vi "COD主界面（列队使用）.vi"() -> (8 "多列列表框":i32(listbox))   [LabVIEW 2016, in "斯坦道CODMn.lvlib"]
uses:
  <vilib>/Analysis/6fits.llb/Curve Fitting Criteria.ctl
  <vilib>/Utility/miscctls.llb/LVPointTypeDef.ctl
  <vilib>/Utility/config.llb/Read Key (I32).vi
  <vilib>/Utility/config.llb/Read Key (Double).vi
  <vilib>/Utility/config.llb/Read Key (Boolean).vi
  <vilib>/Utility/config.llb/Write Key (I32).vi
  <vilib>/Utility/config.llb/Write Key (Double).vi
  <vilib>/Utility/config.llb/Write Key (Boolean).vi
  <vilib>/Waveform/WDTFileIO.llb/Read Waveform from File.vi
  <vilib>/ptbypt/NI_PtbyPt.lvlib
  <vilib>/Utility/config.llb/NI_LVConfig.lvlib
  <vilib>/Analysis/NI_AALPro.lvlib
panel:
  out "氢氧化钠":dbl
  in  "序列号变更":bool
  out "模块版本号":string
  in  "更新程序":bool
  out "进样无液体告警":bool
  out "校准内容显示":string
  out "60分钟超时报警":bool
  in  "远程校准量程":enum16{"L", "H"}(ring)
  in  "远程自动校准浓度":dbl
  in  "仪器参数":bool
  out "CODMn序列号":string
  out "CODMn软件版本：":string
  in  "标样核查量程选择":enum32{"H", "L", "AUTO"}(ring)=enum."AUTO"
  in  "标样浓度":dbl
  in  "零点核查量程选择":enum32{"H", "L", "AUTO"}(ring)=enum."AUTO"
  in  "零点核查浓度":dbl
  out "序列号":string
  in  "采水泵排液时间/s:":i32
  in  "采水泵润洗时间/s:":i32
  in  "采水泵沉淀时间/s:":i32
  in  "采水泵进样时间/s:":i32
  in  "常规版/认证版":enum16{"常规版-酸性", "常规版-碱性", "认证版", "浮台版"}(ring)
  in  "释放串口":bool
  in  "打开串口":bool
  in  "保存参数":dbl[](array[numeric])
  out "报警数字":i16
  out "CODMn工作状态":T1(ring)
  out "ORP-K":string
  out "ORP-B":string
  out "ORP-A":string
  out "x = y?":bool
  out "稀释倍数解释":string
  in  "跨度量程选择":enum32{"H", "L", "AUTO"}(ring)=enum."AUTO"
  in  "跨度液浓度":dbl
  in  "水样：":dbl
  in  "蒸馏水：":dbl
  in  "标液：":dbl
  in  "零点核查样：":dbl
  in  "加标回收样：":dbl
  in  "草酸钠":dbl
  in  "高锰酸钾":dbl
  in  "硫酸":dbl
  out "量程解释说明":string
  in  "高切低阈值:":dbl
  in  "低切高阈值:":dbl
  in  "水样量程选择:":enum16{"L", "H", "自动切换测一次", "自动切换测两次"}(ring)
  in  "氢氧化钠：":dbl
  in  "标准液浓度":dbl
  in  "温度":dbl
  in  "恒温时间":dbl
  in  "当前量程：":enum16{"L", "H"}(ring)
  in  "CODMn零点核查选择":enum16{"零点核查走纯水管", "零点核查走零漂管"}(ring)
  in  "锁定按钮":bool
  in  "低量程稀释倍数:":i8=1
  in  "高量程稀释倍数:":i8=2
  in  "一键写入":bool
  in  "测量模式(公式)":u16(ring)=1 items=["水样测试"=1, "标样核查"=2, "零点核查"=3, "跨度核查"=4, "空白测试"=5, "平行样"=6, "加标回收"=7]
  out "基本量程(显示)":string
  out "测量模式(显示)":string
  out "数据时间":string
  out "断电排液标记":bool
  out "COM":string
  in  "启用5":bool
  in  "校准5":bool
  in  "泵滴定数5":dbl
  in  "浓度5":dbl
  in  "启用4":bool
  in  "校准4":bool
  in  "泵滴定数4":dbl
  in  "浓度4":dbl
  out "波形时间":timestamp
  in  "历史波形":bool
  out "滴定数-ORP值":u16[](array[numeric]) caption="数组"
  in  "关闭 3":bool
  in  "滴定曲线":bool
  out "ORP滴定曲线":u16[](graph)
  out "空白测试标记":bool
  out "跨度核查标记":bool
  in  "量程选择":enum16{"低量程", "高量程", "0-2量程"}(ring)
  in  "手动控制":bool
  in  "选用水样":enum16{"葡萄糖", "草酸钠"}(ring)
  in  "方程系数":cluster{"K":dbl, "b":dbl, "X^2":dbl} {"X^2" format="%#.6g"; "b" format="%#.6g"; "K" format="%#.6g"}
  out "多项式系数":dbl[](array[numeric])
  out "XY图":cluster{"X Values":dbl[], "Y Values":dbl[]}[](graph)
  in  "模型":enum32{"线性", "多项式"}(ring)
  out "启动时间":timestamp format="%<%Y/%m/%d %H:%M:%S>T"
  in  "关闭 2":bool
  out "r^2":dbl format="%.8g"
  out "拟合公式":string
  out "b":dbl format="%#.4g"
  out "K":dbl format="%#.4f"
  in  "启用3":bool
  in  "启用2":bool
  in  "启用1":bool
  in  "校准3":bool
  in  "校准2":bool
  in  "校准1":bool
  in  "泵滴定数3":dbl
  in  "泵滴定数2":dbl
  in  "泵滴定数1":dbl
  in  "浓度3":dbl
  in  "浓度2":dbl
  in  "浓度1":dbl
  in  "写入":bool
  out "零点核查标记":bool
  out "排液故障":bool
  out "进水样超量程":bool
  out "标样核查标记":bool
  out "平行样测量":bool
  out "加标回收测量":bool
  out "质控样测量":bool
  out "待机":bool
  out "校标错误":bool
  out "校零错误":bool
  out "测量错误":bool
  out "草酸钠报警":bool
  out "高锰酸钾报警":bool
  out "加热故障":bool
  out "温控器故障":bool
  out "ORP故障":bool
  out "排液标记":bool
  out "故障标记":bool
  out "校标标记":bool
  out "校零标记":bool
  out "通讯状态":bool
  out "水样测量":bool
  in  "读取":bool
  in  "返回":bool
  in  "校准配置":bool
  in  "零点泵计量数 2":dbl
  in  "标度泵计量数 2":dbl
  out "标度滴定值":dbl
  out "零点滴定值":dbl
  in  "保存":bool
  in  "关闭":bool
  out "仪器时间":timestamp format="%<%Y/%m/%d %H:%M:%S>T"
  out "秒":u16
  out "分":u16
  out "COD浓度（mg/L)":dbl format="%.2g"
  out "进样管":dbl
  out "高锰酸钾":dbl
  out "草酸钠":dbl
  out "硫酸":dbl
  out "实时ORP":dbl
  out "温度℃":dbl
  out "加热":bool
  out "搅拌":bool
  out "进硫酸":bool
  out "进加标回收样":bool
  out "进零点核查样":bool
  out "进标液":bool
  out "进蒸馏水":bool
  out "进水样":bool
  out "进草酸钠":bool
  out "进高锰酸钾":bool
  out "定时启动":bool
  in  "启动":bool
  in  "故障清除":bool
  in  "参数配置":bool
  in  "停止":bool
  in  "单步启动":bool
  out "系统时间":timestamp
  in  "时间校准":bool
  out "模式（受控）":u16
  # "测试时长："
  # "注：遇到加热故障和排液故障时仪器不能正常启动，\n必须排查故障并点击报警清除按钮方可运行。"
  # "mg/L"
  # "基本参数设置"
  # "校零校标结果"
  # "泵计量参数设置"
  # "校零结果："
  # "校零滴定值："
  # "加热恒温温度(℃):"
  # "高锰酸钾："
  # "校标结果："
  # "标度滴定值："
  # "恒温时间(分钟):"
  # "草酸钠："
  # "零点泵计量值："
  # "标准液浓度(mg/L):"
  # "硫酸："
  # "标度泵计量值："
  # "跨度核查浓度："
  # "跨度量程选择："
  # "零点核查浓度："
  # "标样浓度："
  # "零点量程选择："
  # "标样量程选择："
  # "远程校准配置区"
  # "公式读取写入区"
  # "mg/L"
  # "是否启用"
  # "泵滴定数"
  # "浓度"
  # "辅\n助\n计\n算\n区"
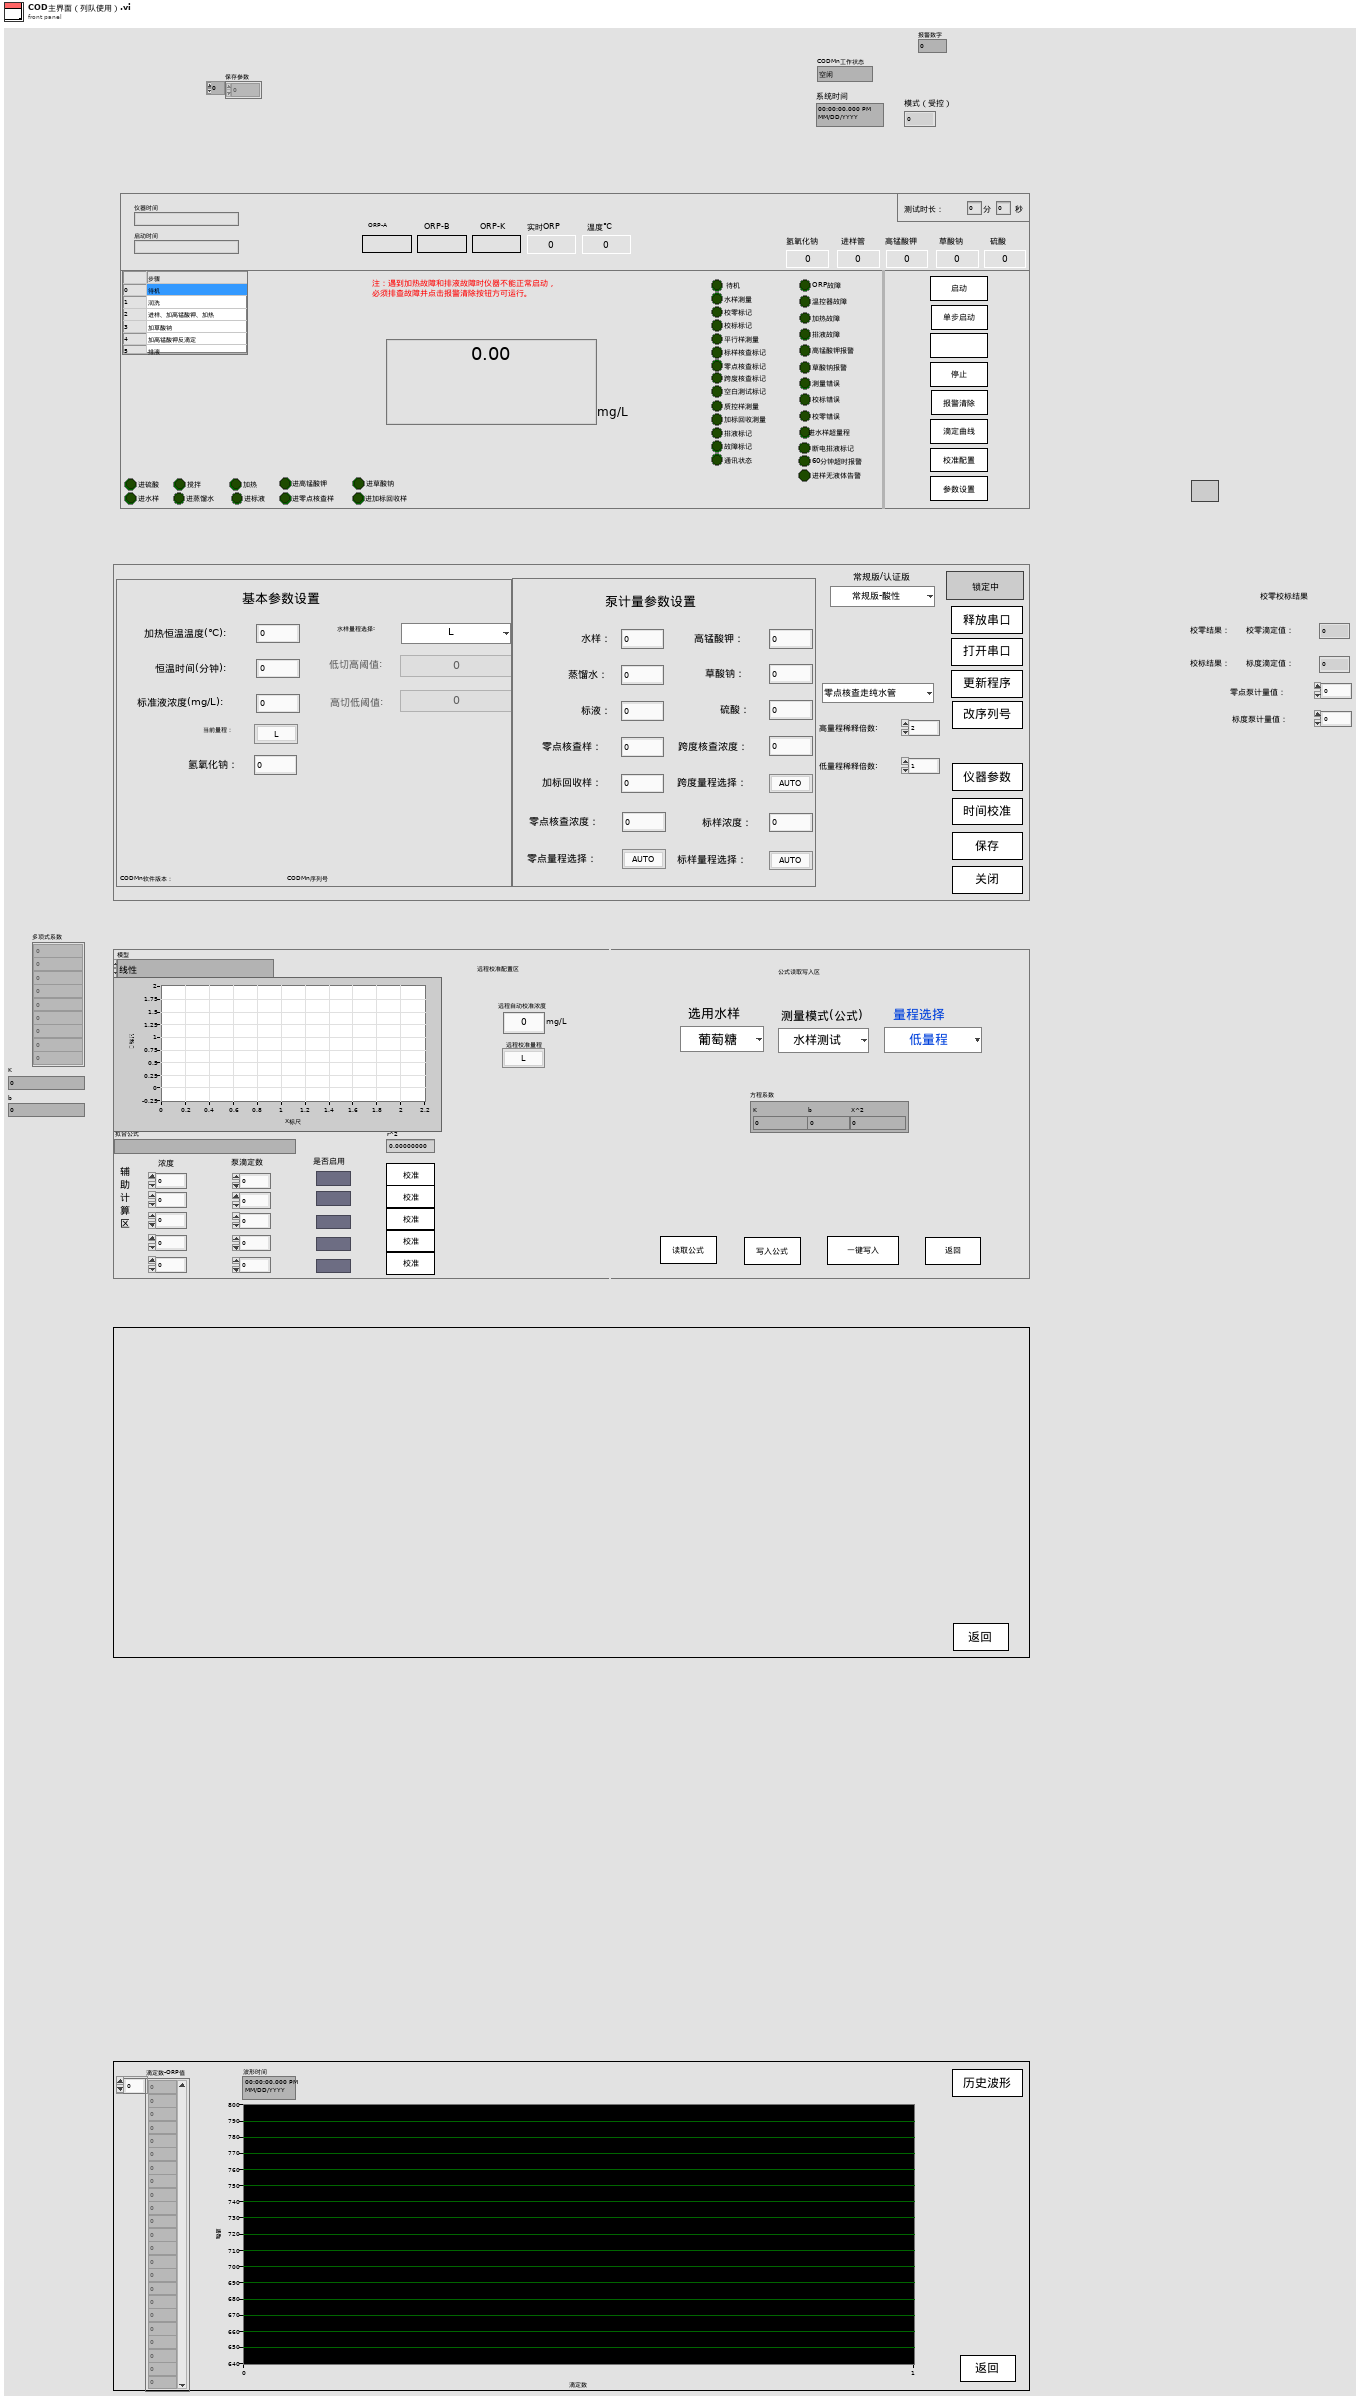
[diagram p1: front panel]
types:
  T1 = enum16{"空闲", "水样测试", "标样核查", "零点核查", "跨度核查", "空白测试", "平行样测试", "质控样", "空白校准", "标样校准", "加标回收"}
  T2 = typedef "LVPointTypeDef.ctl" = cluster{"Horizontal":i16, "Vertical":i16}
  T3 = cluster{"Major":u16, "Minor":u16, "Fix":u16, "Build":u16}
  T4 = typedef "NI_LVConfig.lvlib/Config Data RefNum.ctl" = refnum<k1>
  T5 = cluster{"时间标识":timestamp, "参数":string, "日志信息":string, "流程参数":string}
  T6 = cluster{"时间标识":timestamp, "设备":string, "日志信息":string, "流程参数":string}
  T7 = enum8{"Enabled", "Disabled", "Disabled and Grayed Out"}
  T8 = cluster{"时间":timestamp, "测量模式":string, "数据类型":string, "检测值":sgl, "单位":string, "数据标识":string, "因子编码":string, "标样参考值":sgl, "ORP-A":sgl, "ORP-B":sgl, "ORP-K":sgl, "COD滴定值":sgl, "高锰酸钾滴定数":sgl, "温度":sgl, "量程":sgl, "LastTime":timestamp, "序列号:":string}
  T9 = cluster{"因子编码":u32, "单位":u16, "标样参考值":sgl, "水样数据时间":timestamp, "水样实测值":sgl, "水样数据标识":string, "标样数据时间":timestamp, "标样实测值":sgl, "标样数据标识":string, "空白数据时间":timestamp, "空白实测值":sgl, "空白数据标识":string, "零点核查数据时间":timestamp, "零点核查实测值":sgl, "零点核查数据标识":string, "跨度核查数据时间":timestamp, "跨度核查实测值":sgl, "跨度核查数据标识":string, "加标回收数据时间":timestamp, "加标回收实测值":sgl, "加标回收数据标识":string, "平行样数据时间":timestamp, "平行样实测值":sgl, "平行样数据标识":string}
  T10 = cluster{"控制命令":enum16{"启动测量", "标样核查", "零点核查", "跨度核查", "空白测试", "平行样测试", "加标回收", "空白校准", "标样校准", "初始化（清洗）", "停止测试", "仪器重启", "校时", "模式设置", "测量间隔设置"}, "周期设置类型":enum16{"定点启动", "间隔启动"}, "定时功能启用":bool, "定时间隔":dbl, "24H周期设置":bool[], "零点核查时间":u16, "跨度核查时间":u16, "质控频次":enum16{"关闭", "每天", "星期一", "星期二", "星期三", "星期四", "星期五", "星期六", "星期日"}}
  T11 = cluster{"数组 2[0]":sgl, "数组 2[1]":sgl, "数组 2[2]":sgl, "数组 2[3]":sgl, "数组 2[4]":sgl, "数组 2[5]":sgl, "数组 2[6]":sgl, "数组 2[7]":sgl, "数组 2[8]":sgl, "数组 2[9]":sgl, "数组 2[10]":sgl, "数组 2[11]":sgl, "数组 2[12]":sgl, "数组 2[13]":sgl, "数组 2[14]":sgl, "数组 2[15]":sgl, "数组 2[16]":sgl, "数组 2[17]":sgl, "数组 2[18]":sgl, "数组 2[19]":sgl, "数组 2[20]":sgl, "数组 2[21]":sgl, "数组 2[22]":sgl, "数组 2[23]":sgl, "数组 2[24]":sgl, "数组 2[25]":sgl, "数组 2[26]":sgl, "数组 2[27]":sgl, "数组 2[28]":sgl, "数组 2[29]":sgl, "数组 2[30]":sgl, "数组 2[31]":sgl, "数组 2[32]":sgl, "数组 2[33]":sgl, "数组 2[34]":sgl, "数组 2[35]":sgl, "数组 2[36]":sgl, "数组 2[37]":sgl, "数组 2[38]":sgl, "数组 2[39]":sgl, "数组 2[40]":sgl, "数组 2[41]":sgl}
  T12 = cluster{"ORP故障":bool, "温控器故障":bool, "加热故障":bool, "高锰酸钾报警":bool, "草酸钠报警":bool, "测量错误":bool, "校零错误":bool, "校标错误":bool, " 进水样超量程":bool, "排液阀故障":bool, "60分钟超时报警":bool, "进样无液体报警":bool}
  T13 = cluster{"控制命令":enum16{"启动测量", "标样核查", "零点核查", "跨度核查", "空白测试", "平行样测试", "加标回收", "空白校准", "标样校准", "初始化（清洗）", "停止测试", "仪器重启", "校时", "模式设置", "测量间隔设置"}, "周期设置类型":enum16{"定点启动", "间隔启动"}, "定时功能启用":bool, "定时间隔":dbl, "24H周期设置":bool[], "空白核查时间":u16, "跨度核查时间":u16, "质控频次":enum16{"关闭", "每天", "星期一", "星期二", "星期三", "星期四", "星期五", "星期六", "星期日"}}
  T14 = cluster{"测量量程":dbl, "测量精度":dbl, "测量间隔":dbl, "消解温度":dbl, "消解时长":dbl, "空白校准时间":timestamp, "曲线截距":dbl, "曲线斜率":dbl, "测量检出限":dbl, "测量信号值":dbl, "线性相关系数":dbl, "二次多项式系数":dbl, "标样校准时间":timestamp, "稀释倍数":dbl, "三项式系数":dbl, "空白标定系数":dbl, "量程系数":dbl, "F0/ORPA":dbl, "F1/ORPB":dbl, "F2/ORPK":dbl, "F3":dbl, "F4":dbl, "F5":dbl, "F6":dbl, "F7":dbl, "X0/滴定数":dbl, "量程":dbl}
  T15 = cluster{"确定":bool, "测量量程":dbl, "测量精度":dbl, "测量间隔":dbl, "消解温度":dbl, "消解时长":dbl, "空白校准时间":timestamp, "曲线截距":dbl, "曲线斜率":dbl, "测量检出限":dbl, "测量信号值":dbl, "线性相关系数":dbl, "二次多项式系数":dbl, "标样校准时间":timestamp, "稀释倍数":dbl, "三项式系数":dbl, "空白标定系数":dbl, "量程系数":dbl, "F0/ORPA":dbl, "F1/ORPB":dbl, "F2/ORPK":dbl, "F3":dbl, "F4":dbl, "F5":dbl, "F6":dbl, "F7":dbl, "X0/滴定数":dbl, "量程":dbl}
  T16 = typedef "NI_AALPro.lvlib/Curve Fitting Criteria.ctl" = u16
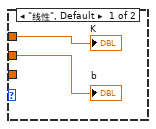
[diagram p5: hidden frame]
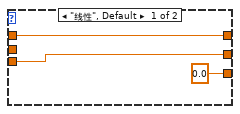
[diagram p7: hidden frame]
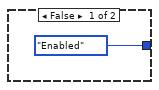
[diagram p8: hidden frame]
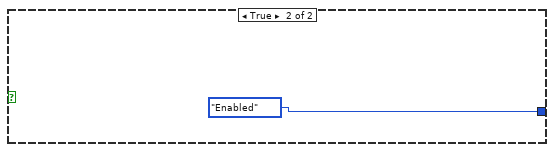
[diagram p9: hidden frame]
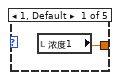
[diagram p14: hidden frame]
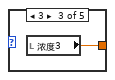
[diagram p15: hidden frame]
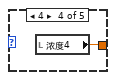
[diagram p16: hidden frame]
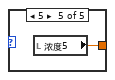
[diagram p17: hidden frame]
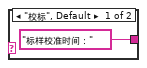
[diagram p18: hidden frame]
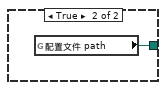
[diagram p19: hidden frame]
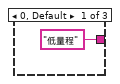
[diagram p20: hidden frame]
diagram:
  n1 = flat-sequence {
    tunnel: [w69] -> w17
    tunnel: [errorcluster {"status"=FALSE, "code"=0, "source"=""} ("错误输出")] -> w54
    tunnel: [w71] -> w16
    frame #0 {
      w93 = "192.168.1.100" ("名称")
      n2 = global write "COD内部交互全局.vi" "量程切换次数"(u8 0 ("量程切换次数")) -> ()
      n3 = global write "COD内部交互全局.vi" "切换量程连续测两次"(FALSE ("切换量程连续测两次")) -> ()
      n4 = global read "COD内部交互全局.vi" "序列号:"() -> (w100:string)
      n5 = property on="窗格" class="Pane"("Origin"=T2 {"Horizontal"=0, "Vertical"=0} ("原点")) -> ()  [unwired: 2 in, 2 out]
      n6 = Empty String/Path?(string/path=w100) -> (empty?=w68:bool)
      n7 = case shown="真" w68 {
        tunnel: w100 -> [w115 _]
        tunnel: [w114 "data\\CODMnSet.ini" ("名称或相对路径")] -> w81
        frame False {
          # "与生产用上位机交互"
          n8 = Concatenate Strings("data\\" ("字符串"), "序列号" ("字符串"), w115, "Set.ini" ("名称或相对路径")) -> (w114:string)
        }
        frame True {
        }
      }
      n9 = String To IP(1:w93) -> (0:w86:u32)
      n10 = IP To String(2:w86) -> (0:w89:string)  [unwired: 1 in]
      n11 = Not Equal?(x=w93, y=w89) -> (x != y?=w94:bool)
      n12 = Concatenate Strings("\\\\" ("字符串"), w89) -> (w88:string)
      n13 = global write "CODMN外部API.vi" "ping"(w94) -> ()
      n14 = String To Path(string=w88) -> (path=w95:path)
      n15 = Build Path(base path=w95, name or relative path=w81) -> (appended path=w90:path)
      n16 = local write "量程选择"(enum16{"低量程", "高量程", "0-2量程"}."低量程" ("量程选择")) -> ()
      n17 = local write "选用水样"(enum16{"葡萄糖", "草酸钠"}."葡萄糖" ("选用水样")) -> ()
      n18 = global write "COD内部交互全局.vi" "配置文件ini"(w81) -> ()
      n19 = case shown="真" w94 {
        tunnel: w90 -> [w105 w109]
        tunnel: [w105 w108] -> w91
        tunnel: [FALSE w107] -> w92
        frame False {
        }
        frame True {
          n20 = call <vilib>:"Check if File or Folder Exists.vi"("path"=w109) -> ("file or folder exists?"=w107:bool, "dup path"=w108:path)  [unwired: 8 in, 1 out]
        }
      }
      n21 = control-ref of="本VI"() -> (w80:refnum<vi>)
      n22 = case shown="假" w92 {
        tunnel: w91 -> [_ w113]
        tunnel: [w111 w113] -> w72
        tunnel: w81 -> [w110 _]
        frame False {
          # "本地文件地址"
          n23 = call <vilib>:"Application Directory.vi"() -> ("Application Directory"=w112:path)
          n24 = Build Path(base path=w112, name or relative path=w110) -> (appended path=w111:path)
        }
        frame True {
          # "网络共享地址"
        }
      }
      n25 = property class="VI"(reference=w80) -> ("Library.Version"=w79:T3)  [unwired: 1 in, 2 out]
      n26 = Unbundle By Name(w79) -> ("Major"=w77:u16, "Minor"=w76:u16, "Fix"=w75:u16, "Build"=w74:u16)
      n27 = Format Into String(format string="模块版本号：%d.%d.%d.%d" ("格式字符串"), w77, w76, w75, w74) -> (resulting string=→"模块版本号":string)  [unwired: 2 in, 1 out]
      n28 = global write "CODMN外部API.vi" "配置文件 path"(w72) -> ()
      n29 = call <vilib>:"Open Config Data.vi"("configuration file path"=w72) -> ("error out"=w82:errorcluster, "refnum"=w83:T4)  [unwired: 8 in, 1 out]
      n30 = vi-ref "斯坦道CODMn.lvlib:CODMn断电保存全局变量.vi"() -> (w96:refnum<vi>)
      n31 = call <userlib>:"Read Panel from INI__ogtk.vi"("error in (no error)"=w82, "VI ref"=w96, "refnum"=w83) -> ("error out"=w84:errorcluster, "refnum out"=w85:T4)  [unwired: 7 in]
      n32 = call <vilib>:"Close Config Data.vi"("error in (no error)"=w84, "refnum"=w85) -> ("error out"=w70:errorcluster)  [unwired: 8 in, 1 out]
      n33 = call <vilib>:"Clear Errors.vi"("error in (no error)"=w70) -> ("error out"=w67:errorcluster)  [unwired: 5 in, 1 out]
      n34 = Read from Text File(file (use dialog)=w72, error in=w67) -> (text=w71:string, error out=w69:errorcluster)  [unwired: 2 in, 2 out]
      "稀释倍数解释" <- "稀释倍数解释：\n稀释倍数选择1，表示不稀释\n默认低量程系数倍数1，高量程系数倍数2\n则低量程为0~8，高量程为0~16" ("稀释倍数解释")
    }
  }
  n35 = Obtain Queue(name (unnamed)="CODMn" ("名称（未命名）"), element data type=cluster{"命令":string} {"命令"="启用模块"} ("元素")) -> (queue out=w64:refnum<queue>, error out=w63:errorcluster)  [unwired: 3 in, 1 out]
  n36 = while {
    tunnel: [w126] -> _
    shift-right: [w124] -> _
    shift-left: w16 -> [w123]
    tunnel: w17 -> [_]
    stop <- FALSE stop-if-true
    n37 = global read "CODMN外部API.vi" "配置文件 path"() -> (w120:path)
    n38 = Wait (ms)(milliseconds to wait=u32 1000 ("等待时间（毫秒）")) -> ()  [unwired: 1 out]
    n39 = Read from Text File(file (use dialog)=w120) -> (text=w124:string, error out=w121:errorcluster)  [unwired: 3 in, 2 out]
    n40 = Not Equal?(x=w124, y=w123) -> (x != y?=w122:bool)
    n41 = case shown="真" w122 {
      tunnel: [w128 w135] -> w126
      tunnel: w120 -> [_ w129]
      tunnel: w121 -> [w128 _]
      frame False {
      }
      frame True {
        # "文件发生改变进行更新，远端和本地都更新"
        n42 = vi-ref "斯坦道CODMn.lvlib:CODMn断电保存全局变量.vi"() -> (w130:refnum<vi>)
        n43 = call <vilib>:"Open Config Data.vi"("configuration file path"=w129) -> ("error out"=w134:errorcluster, "refnum"=w133:T4)  [unwired: 8 in, 1 out]
        n44 = call <userlib>:"Read Panel from INI__ogtk.vi"("error in (no error)"=w134, "VI ref"=w130, "refnum"=w133) -> ("error out"=w132:errorcluster, "refnum out"=w131:T4)  [unwired: 7 in]
        n45 = call <vilib>:"Close Config Data.vi"("error in (no error)"=w132, "refnum"=w131) -> ("error out"=w135:errorcluster)  [unwired: 8 in, 1 out]
      }
    }
  }
  n46 = vi-ref "CODMn通讯.vi"() -> (w55:refnum<vi>)
  n47 = vi-ref "斯坦道CODMn.lvlib:待机状态数据存储写入和切换量程(子VI).vi"() -> (w53:refnum<vi>)
  n48 = vi-ref "斯坦道CODMn.lvlib:定时启动 (子VI).vi"() -> (w40:refnum<vi>)
  n49 = vi-ref "斯坦道CODMn.lvlib:日志报警状态存储 (子VI).vi"() -> (w39:refnum<vi>)
  n50 = vi-ref "斯坦道CODMn.lvlib:高锰酸钾-ORP滴定曲线(子VI).vi"() -> (w26:refnum<vi>)
  n51 = while {
    stop <- FALSE stop-if-true
    # "相差60秒自动校时"
    n52 = global read "运行时序全局变量.vi" "多列列表框"() -> (w137:i32)
    n53 = local read "仪器时间"() -> (w144:timestamp)
    n54 = local read "系统时间"() -> (w145:timestamp)
    n55 = Wait (ms)(milliseconds to wait=u32 1000 ("等待时间（毫秒）")) -> ()  [unwired: 1 out]
    n56 = Build Array(w144) -> (w143:timestamp[])
    n57 = Build Array(w145) -> (w162:timestamp[])
    n58 = Equal?(x=w137, y=u16 5) -> (x = y?=w139:bool)
    n59 = call <vilib>:"Boolean Crossing PtByPt.vi"("direction"=enum16{"either", "false-true", "true-false"}."false-true", "input"=w139) -> ("crossing"=w136:bool)  [unwired: 1 in]
    n60 = call "DateToHex.vi"("DATE"=w143) -> ("数组"=w156:u16[])  [unwired: 10 in]
    n61 = call "DateToHex.vi"("DATE"=w162) -> ("数组"=w161:u16[])  [unwired: 10 in]
    n62 = case shown="真" w136 {
      frame False {
      }
      frame True {
        # "校准结束后自动更新曲线泵滴定数"
        n63 = global read "COD测量模式全局.vi" "测量模式文字实时"() -> (w163:string)
        n64 = global read "COD测量模式全局.vi" "测量模式文字实时"() -> (w168:string)
        n65 = global read "CODMN外部API.vi" "远程反控校准CODMn"() -> (w167:bool)
        n66 = global read "COD内部交互全局.vi" "高锰酸钾"() -> (w171:dbl)
        n67 = Equal?(x=w163, y="校零") -> (x = y?=w164:bool)
        n68 = Equal?(x=w168, y="校标") -> (x = y?=w170:bool)
        n69 = Or(x=w164, y=w170) -> (x .or. y?=w166:bool)
        n70 = case shown="真" w166 {
          tunnel: w171 -> [_ w178]
          tunnel: w163 -> [_ w175]
          frame False {
          }
          frame True {
            w202 = "量程选择" ("section")
            n71 = global read "CODMN外部API.vi" "ping"() -> (w213:bool)
            n72 = case shown="\"校零\"" w175 {
              tunnel: ["标样校准时间：" "空白校准时间："] -> w181
              frame "校标", Default {
              }
              frame "校零" {
              }
            }
            n73 = case shown="假" w213 {
              tunnel: [w222 w225] -> w214
              frame False {
                n74 = global read "COD内部交互全局.vi" "配置文件ini"() -> (w224:string)
                n75 = call <vilib>:"Application Directory.vi"() -> ("Application Directory"=w223:path)
                n76 = Build Path(base path=w223, name or relative path=w224) -> (appended path=w222:path)
              }
              frame True {
                n77 = global read "CODMN外部API.vi" "配置文件 path"() -> (w225:path)
              }
            }
            n78 = Number To Fractional String(number=w178) -> (F-format string=w183:string)  [unwired: 3 in]
            n79 = call <vilib>:"Open Config Data.vi"("configuration file path"=w214) -> ("error out"=w201:errorcluster, "refnum"=w200:T4)  [unwired: 8 in, 1 out]
            n80 = Get Date/Time In Seconds() -> (seconds since 1Jan1904=w179:timestamp)
            n81 = Format Date/Time String(time format string (%c)="%Y/%m/%d %H:%M:%S" ("时间格式字符串(%c)"), seconds (now)=w179) -> (date/time string=w180:string)  [unwired: 1 in]
            n82 = call-poly <vilib>:"Read Key.vi"("section"="标线选择", "error in (no error)"=w201, "key"="选用水样", "refnum"=w200) -> ("error out"=w203:errorcluster, "value"=w196:i32, "refnum out"=w204:T4)  [unwired: 4 in, 1 out]
            n83 = local write "选用水样"(w196) -> ()
            n84 = call-poly <vilib>:"Read Key.vi"("section"=w202, "error in (no error)"=w203, "key"=w202, "refnum"=w204) -> ("error out"=w197:errorcluster, "value"=w199:i32, "refnum out"=w198:T4)  [unwired: 4 in, 1 out]
            n85 = case shown="1" w196 {
              tunnel: ["葡萄糖标线" ("section") "草酸钠标线" ("section")] -> w211
              frame 0, Default {
              }
              frame 1 {
              }
            }
            n86 = local write "量程选择"(w199) -> ()
            n87 = case shown="2" w199 {
              tunnel: ["低量程" "高量程" "0-2量程"] -> w210
              frame 0, Default {
              }
              frame 1 {
              }
              frame 2 {
              }
            }
            n88 = Concatenate Strings(w211, w210) -> (w212:string)
            n89 = call-poly <vilib>:"Read Key.vi"("section"=w212, "error in (no error)"=w197, "key"="当前选用的校准" ("section"), "refnum"=w198) -> ("error out"=w209:errorcluster, "value"=w174:i32, "refnum out"=w208:T4)  [unwired: 4 in, 1 out]
            n90 = call <vilib>:"Close Config Data.vi"("error in (no error)"=w209, "refnum"=w208) -> ()  [unwired: 8 in, 2 out]
            n91 = case shown="2" w174 {
              tunnel: [w215 w216 w217 w218 w219] -> w173
              frame 1, Default {
                n92 = local read "浓度1"() -> (w215:dbl)
              }
              frame 2 {
                n93 = local read "浓度2"() -> (w216:dbl)
              }
              frame 3 {
                n94 = local read "浓度3"() -> (w217:dbl)
              }
              frame 4 {
                n95 = local read "浓度4"() -> (w218:dbl)
              }
              frame 5 {
                n96 = local read "浓度5"() -> (w219:dbl)
              }
            }
            n97 = Number To Fractional String(number=w173) -> (F-format string=w185:string)  [unwired: 3 in]
            n98 = Concatenate Strings("信息：校准结果：\n", "校准浓度：", w185, "滴定数：", w183, w181, w180) -> (w177:string)
            n99 = Bundle(cluster=T5 {"时间标识"=timestamp(0 s since 1904-01-01), "参数"="", "日志信息"="", "流程参数"=""} ("data in"), "时间标识"=w179, "参数"="CODMn" ("table输入"), "日志信息"=w177, "流程参数"="" ("table输入")) -> (w189:T5)
            n100 = call "流程日志字段定义.vi"("table输入"="校准记录", "data in"=w189) -> ("table输出"=w193:string, "columns"=w194:string[], "data out"=w195:T6)  [unwired: 7 in]
            n101 = call "插入数据.vi"("data"=w195, "columns"=w194, "database"="database3.mdb", "table"=w193) -> ()  [unwired: 7 in, 1 out]
            n102 = global write "COD内部交互全局.vi" "当前校准"(w174) -> ()
            n103 = case shown="1, 默认" w174 {
              tunnel: w178 -> [w231 w232 w233 w234 w235]
              frame 1, Default {
                n104 = property on="泵滴定数1" class="DigNum (严格)"("Val(Sgnl)"=w231) -> ()  [unwired: 2 in, 2 out]
              }
              frame 2 {
                n105 = property on="泵滴定数2" class="DigNum (严格)"("Val(Sgnl)"=w232) -> ()  [unwired: 2 in, 2 out]
              }
              frame 3 {
                n106 = property on="泵滴定数3" class="DigNum (严格)"("Val(Sgnl)"=w233) -> ()  [unwired: 2 in, 2 out]
              }
              frame 4 {
                n107 = property on="泵滴定数4" class="DigNum (严格)"("Val(Sgnl)"=w234) -> ()  [unwired: 2 in, 2 out]
              }
              frame 5 {
                n108 = property on="泵滴定数5" class="DigNum (严格)"("Val(Sgnl)"=w235) -> ()  [unwired: 2 in, 2 out]
              }
            }
          }
        }
        n109 = case shown="真" w167 {
          frame False {
          }
          frame True {
            # "校准完自动写入公式"
            n110 = global write "CODMN外部API.vi" "远程反控校准CODMn"(FALSE ("远程反控校准CODMn")) -> ()
          }
        }
      }
    }
    n111 = Index Array(array=w156, index=2 ("索引")) -> (element=w158:u16)
    n112 = Index Array(array=w161, index=2 ("索引")) -> (element=w159:u16)
    n113 = Split Number(x=w158) -> (hi(x)=w152:u8)  [unwired: 1 out]
    n114 = Split Number(x=w159) -> (hi(x)=w155:u8)  [unwired: 1 out]
    n115 = To Byte Integer(number=w152) -> (8bit integer=w151:i8)
    n116 = To Byte Integer(number=w155) -> (8bit integer=w154:i8)
    n117 = Subtract(x=w151, y=w154) -> (x-y=w153:i8)
    n118 = Absolute Value(x=w153) -> (abs(x)=w150:i8)
    n119 = local read "通讯状态"() -> (w147:bool)
    n120 = Greater Or Equal?(x=w150, y=i8 5) -> (x >= y?=w148:bool)
    n121 = And(x=w148, y=w147) -> (x .and. y?=w146:bool)
    n122 = case shown="真" w146 {
      frame False {
      }
      frame True {
        # "相差60秒时间自动校准"
        n123 = flat-sequence {
          frame #0 {
            n124 = property on="时间校准" class="Bool (严格)"("Val(Sgnl)"=TRUE ("值(信号)")) -> ()  [unwired: 2 in, 2 out]
          }
          frame #1 {
            n125 = Wait (ms)(milliseconds to wait=u32 500 ("等待时间（毫秒）")) -> ()  [unwired: 1 out]
          }
          frame #2 {
            n126 = property on="时间校准" class="Bool (严格)"("Val(Sgnl)"=FALSE ("值(信号)")) -> ()  [unwired: 2 in, 2 out]
          }
        }
      }
    }
  }
  n127 = while {
    tunnel: w17 -> [_]
    stop <- FALSE stop-if-true
    # "赋值循环"
    n128 = flat-sequence {
      frame #0 {
        # "测量数据区"
        n129 = global read "COD内部交互全局.vi" "data"() -> (w483:T8)
        n130 = global read "COD测量模式全局.vi" "测量模式文字实时"() -> (w469:string)
        "测量模式(显示)" <- w469
        n131 = global read "CODMn断电保存全局变量.vi" "测量数据区"() -> (w478:T9)
        n132 = Unbundle By Name(w483) -> ("时间"=w482:timestamp, "检测值"=w481:sgl, "数据标识"=w480:string)
        n133 = case shown="\"水样测试\"" w469 {
          tunnel: w478 -> [w484 w489 w494 w499 w504 w509 w514 w519 w524 w529]
          tunnel: [w484 w488 w493 w495 w503 w508 w513 w518 w520 w528] -> w479
          tunnel: w482 -> [_ w487 w492 w498 w502 w507 w512 w517 w523 w527]
          tunnel: w481 -> [_ w486 w491 w497 w501 w506 w511 w516 w522 w526]
          tunnel: w480 -> [_ w485 w490 w496 w500 w505 w510 w515 w521 w525]
          frame "", Default {
          }
          frame "水样测试" {
            n134 = Bundle By Name(cluster=w489, "水样数据时间"=w487, "水样实测值"=w486, "水样数据标识"=w485) -> (w488:T9)
          }
          frame "标样核查" {
            n135 = Bundle By Name(cluster=w494, "标样数据时间"=w492, "标样实测值"=w491, "标样数据标识"=w490) -> (w493:T9)
          }
          frame "跨度核查" {
            n136 = Bundle By Name(cluster=w499, "跨度核查数据时间"=w498, "跨度核查实测值"=w497, "跨度核查数据标识"=w496) -> (w495:T9)
          }
          frame "零点核查" {
            n137 = Bundle By Name(cluster=w504, "零点核查数据时间"=w502, "零点核查实测值"=w501, "零点核查数据标识"=w500) -> (w503:T9)
          }
          frame "空白测试" {
            n138 = Bundle By Name(cluster=w509, "空白数据时间"=w507, "空白实测值"=w506, "空白数据标识"=w505) -> (w508:T9)
          }
          frame "加标回收" {
            n139 = Bundle By Name(cluster=w514, "加标回收数据时间"=w512, "加标回收实测值"=w511, "加标回收数据标识"=w510) -> (w513:T9)
          }
          frame "平行样" {
            n140 = Bundle By Name(cluster=w519, "平行样数据时间"=w517, "平行样实测值"=w516, "平行样数据标识"=w515) -> (w518:T9)
          }
          frame "校零" {
            n141 = Bundle By Name(cluster=w524, "空白数据时间"=w523, "空白实测值"=w522, "空白数据标识"=w521) -> (w520:T9)
          }
          frame "校标" {
            n142 = Bundle By Name(cluster=w529, "标样数据时间"=w527, "标样实测值"=w526, "标样数据标识"=w525) -> (w528:T9)
          }
        }
        n143 = Unbundle By Name(w478) -> ("水样实测值"=w475:sgl)
        n144 = feedback-in #1(w478) -> ()
        n145 = feedback #1(w478) -> (w477:T9)
        n146 = global read "CODMn断电保存全局变量.vi" "水样测试量程"() -> (w471:enum16{"L", "H"})
        n147 = Unbundle By Name(w477) -> ("水样实测值"=w476:sgl)
        n148 = feedback #2(w471) -> (w472:enum16{"L", "H"})
        n149 = feedback-in #2(w471) -> ()
        n150 = Not Equal?(x=w472, y=w471) -> (x != y?=w470:bool)
        n151 = Not Equal?(x=w475, y=w476) -> (x != y?=w474:bool)
        n152 = global write "CODMn断电保存全局变量.vi" "测量数据区"(w479) -> ()
        n153 = Or(x=w474, y=w470) -> (x .or. y?=w473:bool)
        n154 = case shown="真" w473 {
          frame False {
          }
          frame True {
            # "水样值发送改变存储本地"
            n155 = call "配置文件保存.vi"() -> ()  [unwired: 12 in]
          }
        }
      }
    }
    n156 = flat-sequence {
      frame #0 {
        # "局部变量给内部交互用全局变量"
        n157 = local read "温度℃"() -> (w265:dbl)
        n158 = local read "COD浓度（mg/L)"() -> (w271:dbl)
        n159 = local read "CODMn工作状态"() -> (w274:T1)
        n160 = local read "多列列表框"() -> (w272:i32)
        n161 = local read "标准液浓度"() -> (w270:dbl)
        n162 = local read "高锰酸钾报警"() -> (w268:bool)
        n163 = local read "断电排液标记"() -> (w267:bool)
        n164 = local read "实时ORP"() -> (w264:dbl)
        n165 = local read "故障标记"() -> (w273:bool)
        n166 = local read "高锰酸钾"() -> (w266:dbl)
        n167 = global write "COD内部交互全局.vi" "实时温度"(w265) -> ()
        n168 = local read "待机"() -> (w269:bool)
        n169 = global write "运行时序全局变量.vi" "多列列表框"(w272) -> ()
        n170 = global write "COD内部交互全局.vi" "故障标记"(w273) -> ()
        n171 = global write "COD内部交互全局.vi" "ORP显示"(w264) -> ()
        n172 = global write "COD浓度全局变量.vi" "标准液浓度"(w270) -> ()
        n173 = global write "COD内部交互全局.vi" "高锰酸钾"(w266) -> ()
        n174 = global write "COD内部交互全局.vi" "待机"(w269) -> ()
        n175 = global write "COD测量模式全局.vi" "CODMn工作状态"(w274) -> ()
        n176 = global write "COD内部交互全局.vi" "高锰酸钾报警"(w268) -> ()
        n177 = global write "COD内部交互全局.vi" "断电排液标记"(w267) -> ()
        n178 = global write "COD浓度全局变量.vi" "COD浓度（mg/L)"(w271) -> ()
      }
    }
    n179 = flat-sequence {
      frame #0 {
        # "断电保存全局给局部变量"
        n180 = global read "CODMn断电保存全局变量.vi" "高切低阈值:"() -> (w544:dbl)
        n181 = global read "CODMn断电保存全局变量.vi" "低切高阈值:"() -> (w543:dbl)
        n182 = global read "CODMn断电保存全局变量.vi" "跨度液浓度"() -> (w541:dbl)
        n183 = global read "COD内部交互全局.vi" "波形时间"() -> (→"波形时间":timestamp)
        n184 = global read "CODMn断电保存全局变量.vi" "启动时间"() -> (→"启动时间":timestamp)
        n185 = global read "CODMn断电保存全局变量.vi" "标样浓度"() -> (w539:dbl)
        n186 = global read "CODMn断电保存全局变量.vi" "定时控制"() -> (w534:T10)
        n187 = global read "CODMn断电保存全局变量.vi" "CODMn跨度量程选择"() -> (w545:enum32{"H", "L", "AUTO"})
        n188 = global read "CODMn断电保存全局变量.vi" "标样核查量程选择"() -> (w536:enum32{"H", "L", "AUTO"})
        n189 = global read "CODMn断电保存全局变量.vi" "零点核查量程选择"() -> (w538:enum32{"H", "L", "AUTO"})
        n190 = global read "CODMn断电保存全局变量.vi" "测量模式(公式)"() -> (w546:u16)
        n191 = global read "COD内部交互全局.vi" "滴定数-ORP值"() -> (→"滴定数-ORP值":u16[])
        n192 = global read "CODMn断电保存全局变量.vi" "常规版/认证版"() -> (w540:enum16{"常规版-酸性", "常规版-碱性", "认证版", "浮台版"})
        n193 = global read "CODMn断电保存全局变量.vi" "自动切换量程:"() -> (w542:enum16{"L", "H", "自动切换测一次", "自动切换测两次"})
        n194 = global read "CODMn断电保存全局变量.vi" "零点核查浓度"() -> (w537:dbl)
        n195 = global read "COD内部交互全局.vi" "ORP滴定曲线"() -> (→"ORP滴定曲线":u16[])
        n196 = local write "高切低阈值:"(w544) -> ()
        n197 = local write "标样浓度"(w539) -> ()
        n198 = Unbundle By Name(w534) -> ("定时功能启用"=→"定时启动":bool)
        n199 = local write "跨度液浓度"(w541) -> ()
        n200 = local write "低切高阈值:"(w543) -> ()
        n201 = local write "标样核查量程选择"(w536) -> ()
        n202 = local write "水样量程选择:"(w542) -> ()
        n203 = local write "常规版/认证版"(w540) -> ()
        n204 = local write "零点核查浓度"(w537) -> ()
        n205 = local write "零点核查量程选择"(w538) -> ()
        n206 = local write "测量模式(公式)"(w546) -> ()
        n207 = local write "跨度量程选择"(w545) -> ()
      }
    }
    n208 = flat-sequence {
      frame #0 {
        # "保存参数赋值"
        n209 = Multiply(x="温度", y=10.0) -> (x*y=w249:dbl)
        n210 = Multiply(x="标准液浓度", y=100.0) -> (x*y=w246:dbl)
        n211 = Build Array(w249, "恒温时间", w246, "氢氧化钠：", "当前量程：", "水样：", "蒸馏水：", "标液：", "零点核查样：", "加标回收样：", "高锰酸钾", "草酸钠", "硫酸", "零点泵计量数 2", "标度泵计量数 2", "高量程稀释倍数:", "低量程稀释倍数:", "CODMn零点核查选择") -> (w243:dbl[])
        n212 = local write "保存参数"(w243) -> ()
      }
    }
    n213 = flat-sequence {
      frame #0 {
        # "显示量程说明"
        n214 = global read "COD内部交互全局.vi" "通讯状态"() -> (→"通讯状态":bool)
        n215 = global read "CODMn断电保存全局变量.vi" "MB通信方式选择"() -> (w547:enum16{"串口", "TCP"})
        n216 = local read "低量程稀释倍数:"() -> (w561:i8)
        n217 = local read "高量程稀释倍数:"() -> (w551:i8)
        n218 = case shown="\"TCP\"" w547 {
          tunnel: [w564 w565] -> w552
          frame "串口", Default {
            n219 = global read "CODMn断电保存全局变量.vi" "VISA resource name"() -> (w564:refnum<visa-resource-name>)
          }
          frame "TCP" {
            n220 = global read "CODMn断电保存全局变量.vi" "IP"() -> (w565:string)
          }
        }
        "COM" <- w552
        n221 = Multiply(x=w561, y=i8 8) -> (x*y=w553:i8)
        n222 = Multiply(x=w551, y=i8 8) -> (x*y=w549:i8)
        n223 = Number To Decimal String(number=w553) -> (decimal integer string=w558:string)  [unwired: 1 in]
        n224 = Number To Decimal String(number=w549) -> (decimal integer string=w556:string)  [unwired: 1 in]
        n225 = Concatenate Strings("L低量程范围:0~" ("量程解释说明"), w558, "(mg/L)\n\nH高量程范围:" ("量程解释说明"), "0" ("字符串"), "~" ("量程解释说明"), w556, "(mg/L)" ("量程解释说明")) -> (→"量程解释说明":string)
      }
    }
    n226 = flat-sequence {
      frame #0 {
        # "参数赋值（只在读取参数时候改变一次）"
        n227 = global read "COD内部交互全局.vi" "读取浮台参数显示"() -> (w276:bool)
        n228 = global read "COD内部交互全局.vi" "读取浮台参数"() -> (w275:u16[])
        n229 = global read "COD内部交互全局.vi" "读取参数显示"() -> (w277:bool)
        n230 = global read "COD内部交互全局.vi" "读取参数"() -> (w278:u16[])
        n231 = case shown="真" w276 {
          tunnel: w275 -> [_ w284]
          frame False {
          }
          frame True {
            n232 = Index Array(array=w284) -> (element #1=w283:u16, element #2=w282:u16, element #3=w281:u16, element #4=w280:u16)  [unwired: 4 in]
            n233 = global write "COD内部交互全局.vi" "读取浮台参数显示"(FALSE ("读取参数显示")) -> ()
            n234 = local write "采水泵进样时间/s:"(w283) -> ()
            n235 = local write "采水泵润洗时间/s:"(w282) -> ()
            n236 = local write "采水泵沉淀时间/s:"(w281) -> ()
            n237 = local write "采水泵排液时间/s:"(w280) -> ()
          }
        }
        n238 = case shown="真" w277 {
          tunnel: w278 -> [_ w302]
          frame False {
          }
          frame True {
            n239 = Index Array(array=w302) -> (element #1=w311:u16, element #2=w323:u16, element #3=w307:u16, element #4=w285:u16, element #5=w310:u16, element #6=w309:u16, element #7=w322:u16, element #8=w321:u16, element #9=w320:u16, element #10=w319:u16, element #11=w318:u16, element #12=w317:u16, element #13=w316:u16, element #14=w315:u16, element #15=w314:u16, element #16=w305:u16, element #17=w304:u16, element #18=w303:u16, element #19=w300:u16, element #20=w299:u16, element #21=w298:u16, element #22=w297:u16, element #23=w296:u16, element #27=w292:u16, element #28=w291:u16, element #29=w290:u16, element #30=w289:u16, element #31=w288:u16)  [unwired: 31 in, 3 out]
            n240 = global write "COD内部交互全局.vi" "读取参数显示"(FALSE ("读取参数显示")) -> ()
            n241 = local write "水样："(w309) -> ()
            n242 = local write "标液："(w321) -> ()
            n243 = local write "硫酸"(w316) -> ()
            n244 = local write "零点核查样："(w320) -> ()
            n245 = local write "加标回收样："(w319) -> ()
            n246 = local write "当前量程："(w310) -> ()
            n247 = local write "蒸馏水："(w322) -> ()
            n248 = local write "恒温时间"(w323) -> ()
            n249 = local write "高锰酸钾"(w318) -> ()
            n250 = local write "草酸钠"(w317) -> ()
            n251 = local write "零点泵计量数 2"(w315) -> ()
            n252 = local write "标度泵计量数 2"(w314) -> ()
            n253 = local write "高量程稀释倍数:"(w305) -> ()
            n254 = local write "低量程稀释倍数:"(w304) -> ()
            n255 = local write "CODMn零点核查选择"(w303) -> ()
            n256 = Build Array(w300, w299, w298, w297, w296) -> (w295:u16[])
            n257 = Build Array(w292, w291, w290, w289, w288) -> (w287:u16[])
            n258 = Divide(x=w311, y=u16 10) -> (x/y=w312:dbl)
            n259 = Divide(x=w307, y=u16 100) -> (x/y=w306:dbl)
            n260 = local write "氢氧化钠："(w285) -> ()
            n261 = local write "温度"(w312) -> ()
            n262 = local write "标准液浓度"(w306) -> ()
            n263 = call "HexToString.vi"("数组"=w287) -> ("字符串"=w286:string)  [unwired: 10 in]
            "CODMn序列号" <- w286
            "序列号" <- w286
            n264 = call "FATEK_HexToString.vi"("数组"=w295) -> ("STRING"=w294:string[])  [unwired: 10 in]
            n265 = Index Array(array=w294) -> (element=→"CODMn软件版本：":string)  [unwired: 1 in]
            n266 = global write "COD内部交互全局.vi" "序列号:"(w286) -> ()
          }
        }
      }
    }
    n267 = flat-sequence {
      frame #0 {
        # "权限隐藏和显示功能"
        n268 = local read "x = y?"() -> (w567:bool)
        n269 = property on="更新程序" class="Bool (严格)"("Visible"=w567) -> ()  [unwired: 2 in, 2 out]
        n270 = property on="释放串口" class="Bool"("Visible"=w567) -> ()  [unwired: 2 in, 2 out]
        n271 = property on="打开串口" class="Bool"("Visible"=w567) -> ()  [unwired: 2 in, 2 out]
        n272 = property on="序列号变更" class="Bool"("Visible"=w567) -> ()  [unwired: 2 in, 2 out]
        n273 = property on="常规版/认证版" class="Enum (严格)"("Visible"=w567) -> ()  [unwired: 2 in, 2 out]
        n274 = property on="CODMn零点核查选择" class="Enum (严格)"("Visible"=w567) -> ()  [unwired: 2 in, 2 out]
        n275 = property on="低量程稀释倍数:" class="DigNum (严格)"("Visible"=w567) -> ()  [unwired: 2 in, 2 out]
        n276 = property on="稀释倍数解释" class="Str"("Visible"=w567) -> ()  [unwired: 2 in, 2 out]
        n277 = property on="高量程稀释倍数:" class="DigNum (严格)"("Visible"=w567) -> ()  [unwired: 2 in, 2 out]
        n278 = local read "常规版/认证版"() -> (w582:enum16{"常规版-酸性", "常规版-碱性", "认证版", "浮台版"})
        n279 = case shown="\"浮台版\"" w582 {
          tunnel: [T7."Enabled" ("禁用") T7."Enabled" ("禁用") T7."Disabled and Grayed Out" ("禁用") T7."Enabled" ("禁用")] -> w581
          tunnel: [i32[] [2] ("禁用项[]") i32[] [2] ("禁用项[]") i32[] [] ("禁用项[]") i32[] [2] ("禁用项[]")] -> w580
          tunnel: [w591 w596 T7."Disabled and Grayed Out" ("禁用") w607] -> w579
          tunnel: [w590 FALSE FALSE TRUE] -> w578
          tunnel: [w591 w596 T7."Disabled and Grayed Out" ("禁用") w607] -> w568
          tunnel: [w590 TRUE FALSE FALSE] -> w566
          frame "常规版-酸性", Default {
            w590 = FALSE
            w591 = T7."Enabled" ("禁用")
          }
          frame "常规版-碱性" {
            w596 = T7."Enabled" ("禁用")
          }
          frame "认证版" {
            w602 = u16 1 items=["水样测试"=1, "标样核查"=2, "零点核查"=3, "跨度核查"=4, "空白测试"=5, "平行样"=6, "加标回收"=7] ("测量模式(公式)")
            n280 = global write "CODMn断电保存全局变量.vi" "测量模式(公式)"(w602) -> ()
          }
          frame "浮台版" {
            w607 = T7."Enabled" ("禁用")
          }
        }
        n281 = control-ref of="水样："() -> (w577:refnum<vi>)
        n282 = control-ref of="蒸馏水："() -> (w576:refnum<vi>)
        n283 = control-ref of="标液："() -> (w575:refnum<vi>)
        n284 = control-ref of="零点核查样："() -> (w574:refnum<vi>)
        n285 = control-ref of="加标回收样："() -> (w573:refnum<vi>)
        n286 = local read "水样量程选择:"() -> (w584:enum16{"L", "H", "自动切换测一次", "自动切换测两次"})
        n287 = control-ref of="量程解释说明"() -> (w571:refnum<vi>)
        n288 = control-ref of="氢氧化钠："() -> (w572:refnum<vi>)
        n289 = Not Equal To 0?(x=w584) -> (x != 0?=w583:bool)
        n290 = control-ref of="进样管"() -> (w569:refnum<vi>)
        n291 = Build Array(w577, w576, w575, w574, w573, w571, w572, w569) -> (w570:refnum<vi>[])
        n292 = Select(t=T7."Enabled" ("禁用"), s=w583, f=T7."Disabled and Grayed Out" ("禁用")) -> (s? t:f=w585:T7)
        n293 = for {
          tunnel: w570 -> [w589] mode=indexing
          tunnel: w568 -> [w588]
          n294 = property class="Ctl"(reference=w589, "DisabledEnum"=w588) -> ()  [unwired: 1 in, 2 out]
        }
        n295 = property on="低切高阈值:" class="DigNum (严格)"("DisabledEnum"=w585) -> ()  [unwired: 2 in, 2 out]
        n296 = property on="高切低阈值:" class="DigNum (严格)"("DisabledEnum"=w585) -> ()  [unwired: 2 in, 2 out]
        n297 = property on="采水泵润洗时间/s:" class="DigNum (严格)"("Visible"=w578) -> ()  [unwired: 2 in, 2 out]
        n298 = property on="采水泵沉淀时间/s:" class="DigNum (严格)"("Visible"=w578) -> ()  [unwired: 2 in, 2 out]
        n299 = property on="采水泵排液时间/s:" class="DigNum (严格)"("Visible"=w578) -> ()  [unwired: 2 in, 2 out]
        n300 = property on="采水泵进样时间/s:" class="DigNum (严格)"("Visible"=w578) -> ()  [unwired: 2 in, 2 out]
        n301 = property on="一键写入" class="Bool (严格)"("DisabledEnum"=w579) -> ()  [unwired: 2 in, 2 out]
        n302 = property on="量程选择" class="Enum (严格)"("Disabled Items []"=w580) -> ()  [unwired: 2 in, 2 out]
        n303 = property on="测量模式(公式)" class="Ring (严格)"("DisabledEnum"=w581) -> ()  [unwired: 2 in, 2 out]
        n304 = property on="氢氧化钠：" class="DigNum (严格)"("Visible"=w566) -> ()  [unwired: 2 in, 2 out]
        n305 = property on="氢氧化钠" class="DigNum (严格)"("Visible"=w566) -> ()  [unwired: 2 in, 2 out]
      }
    }
    n306 = flat-sequence {
      frame #0 {
        # "公式读取显示（只在读取公式的时候改变一次）"
        n307 = global read "COD内部交互全局.vi" "读取公式显示"() -> (w324:bool)
        n308 = case shown="真" w324 {
          frame False {
          }
          frame True {
            n309 = global write "COD内部交互全局.vi" "读取公式显示"(FALSE ("读取参数显示")) -> ()
            n310 = global read "COD内部交互全局.vi" "读取公式"() -> (w334:u16[])
            n311 = Array Subset(array=w334, index=10 ("索引"), length=84 ("长度")) -> (w329:u16[])
            n312 = One Button Dialog(message="公式读取成功！" ("消息")) -> ()  [unwired: 1 in, 1 out]
            n313 = local read "测量模式(公式)"() -> (w332:u16)
            n314 = call "浮点CDAB转换COD.vi"("数组"=w329) -> ("数组 2"=w330:sgl[])  [unwired: 10 in]
            n315 = Array To Cluster(array=w330) -> (cluster=w333:T11)
            n316 = case shown="1" w332 {
              tunnel: [cluster{"X":dbl, "b":dbl, "X^2":dbl} {"X"=999.0, "b"=999.0, "X^2"=999.0} ("方程系数") w337 w356 w375 w394 w413 w432 w451] -> w331
              tunnel: w333 -> [_ w336 w355 w374 w393 w412 w431 w450]
              frame 0, Default {
              }
              frame 1 {
                n317 = local read "量程选择"() -> (w339:enum16{"低量程", "高量程", "0-2量程"})
                n318 = case shown="\"低量程\", 默认" w339 {
                  tunnel: w336 -> [w346 w350 w354]
                  tunnel: [w345 w349 w353] -> w342
                  tunnel: [w344 w348 w352] -> w341
                  tunnel: [w343 w347 w351] -> w340
                  frame "低量程", Default {
                    n319 = Unbundle By Name(w346) -> ("数组 2[0]"=w345:sgl, "数组 2[1]"=w344:sgl, "数组 2[2]"=w343:sgl)
                  }
                  frame "高量程" {
                    n320 = Unbundle By Name(w350) -> ("数组 2[3]"=w349:sgl, "数组 2[4]"=w348:sgl, "数组 2[5]"=w347:sgl)
                  }
                  frame "0-2量程" {
                    n321 = Unbundle By Name(w354) -> ("数组 2[6]"=w353:sgl, "数组 2[7]"=w352:sgl, "数组 2[8]"=w351:sgl)
                  }
                }
                n322 = Bundle By Name(cluster=cluster{"X":dbl, "b":dbl, "X^2":dbl} {"X"=0.0, "b"=0.0, "X^2"=0.0} ("方程系数"), "X"=w342, "b"=w341, "X^2"=w340) -> (w337:cluster{"X":dbl, "b":dbl, "X^2":dbl})
              }
              frame 2 {
                n323 = local read "量程选择"() -> (w358:enum16{"低量程", "高量程", "0-2量程"})
                n324 = case shown="\"高量程\"" w358 {
                  tunnel: w355 -> [w365 w369 w373]
                  tunnel: [w364 w368 w372] -> w361
                  tunnel: [w363 w367 w371] -> w360
                  tunnel: [w362 w366 w370] -> w359
                  frame "低量程", Default {
                    n325 = Unbundle By Name(w365) -> ("数组 2[6]"=w364:sgl, "数组 2[7]"=w363:sgl, "数组 2[8]"=w362:sgl)
                  }
                  frame "高量程" {
                    n326 = Unbundle By Name(w369) -> ("数组 2[9]"=w368:sgl, "数组 2[10]"=w367:sgl, "数组 2[11]"=w366:sgl)
                  }
                  frame "0-2量程" {
                    n327 = Unbundle By Name(w373) -> ("数组 2[6]"=w372:sgl, "数组 2[7]"=w371:sgl, "数组 2[8]"=w370:sgl)
                  }
                }
                n328 = Bundle By Name(cluster=cluster{"X":dbl, "b":dbl, "X^2":dbl} {"X"=0.0, "b"=0.0, "X^2"=0.0} ("方程系数"), "X"=w361, "b"=w360, "X^2"=w359) -> (w356:cluster{"X":dbl, "b":dbl, "X^2":dbl})
              }
              frame 3 {
                n329 = local read "量程选择"() -> (w377:enum16{"低量程", "高量程", "0-2量程"})
                n330 = case shown="\"高量程\"" w377 {
                  tunnel: w374 -> [w384 w388 w392]
                  tunnel: [w383 w387 w391] -> w380
                  tunnel: [w382 w386 w390] -> w379
                  tunnel: [w381 w385 w389] -> w378
                  frame "低量程", Default {
                    n331 = Unbundle By Name(w384) -> ("数组 2[12]"=w383:sgl, "数组 2[13]"=w382:sgl, "数组 2[14]"=w381:sgl)
                  }
                  frame "高量程" {
                    n332 = Unbundle By Name(w388) -> ("数组 2[15]"=w387:sgl, "数组 2[16]"=w386:sgl, "数组 2[17]"=w385:sgl)
                  }
                  frame "0-2量程" {
                    n333 = Unbundle By Name(w392) -> ("数组 2[6]"=w391:sgl, "数组 2[7]"=w390:sgl, "数组 2[8]"=w389:sgl)
                  }
                }
                n334 = Bundle By Name(cluster=cluster{"X":dbl, "b":dbl, "X^2":dbl} {"X"=0.0, "b"=0.0, "X^2"=0.0} ("方程系数"), "X"=w380, "b"=w379, "X^2"=w378) -> (w375:cluster{"X":dbl, "b":dbl, "X^2":dbl})
              }
              frame 4 {
                n335 = local read "量程选择"() -> (w396:enum16{"低量程", "高量程", "0-2量程"})
                n336 = case shown="\"高量程\"" w396 {
                  tunnel: w393 -> [w403 w407 w411]
                  tunnel: [w402 w406 w410] -> w399
                  tunnel: [w401 w405 w409] -> w398
                  tunnel: [w400 w404 w408] -> w397
                  frame "低量程", Default {
                    n337 = Unbundle By Name(w403) -> ("数组 2[18]"=w402:sgl, "数组 2[19]"=w401:sgl, "数组 2[20]"=w400:sgl)
                  }
                  frame "高量程" {
                    n338 = Unbundle By Name(w407) -> ("数组 2[21]"=w406:sgl, "数组 2[22]"=w405:sgl, "数组 2[23]"=w404:sgl)
                  }
                  frame "0-2量程" {
                    n339 = Unbundle By Name(w411) -> ("数组 2[6]"=w410:sgl, "数组 2[7]"=w409:sgl, "数组 2[8]"=w408:sgl)
                  }
                }
                n340 = Bundle By Name(cluster=cluster{"X":dbl, "b":dbl, "X^2":dbl} {"X"=0.0, "b"=0.0, "X^2"=0.0} ("方程系数"), "X"=w399, "b"=w398, "X^2"=w397) -> (w394:cluster{"X":dbl, "b":dbl, "X^2":dbl})
              }
              frame 5 {
                n341 = local read "量程选择"() -> (w415:enum16{"低量程", "高量程", "0-2量程"})
                n342 = case shown="\"高量程\"" w415 {
                  tunnel: w412 -> [w422 w426 w430]
                  tunnel: [w421 w425 w429] -> w418
                  tunnel: [w420 w424 w428] -> w417
                  tunnel: [w419 w423 w427] -> w416
                  frame "低量程", Default {
                    n343 = Unbundle By Name(w422) -> ("数组 2[24]"=w421:sgl, "数组 2[25]"=w420:sgl, "数组 2[26]"=w419:sgl)
                  }
                  frame "高量程" {
                    n344 = Unbundle By Name(w426) -> ("数组 2[27]"=w425:sgl, "数组 2[28]"=w424:sgl, "数组 2[29]"=w423:sgl)
                  }
                  frame "0-2量程" {
                    n345 = Unbundle By Name(w430) -> ("数组 2[6]"=w429:sgl, "数组 2[7]"=w428:sgl, "数组 2[8]"=w427:sgl)
                  }
                }
                n346 = Bundle By Name(cluster=cluster{"X":dbl, "b":dbl, "X^2":dbl} {"X"=0.0, "b"=0.0, "X^2"=0.0} ("方程系数"), "X"=w418, "b"=w417, "X^2"=w416) -> (w413:cluster{"X":dbl, "b":dbl, "X^2":dbl})
              }
              frame 6 {
                n347 = local read "量程选择"() -> (w434:enum16{"低量程", "高量程", "0-2量程"})
                n348 = case shown="\"高量程\"" w434 {
                  tunnel: w431 -> [w441 w445 w449]
                  tunnel: [w440 w444 w448] -> w437
                  tunnel: [w439 w443 w447] -> w436
                  tunnel: [w438 w442 w446] -> w435
                  frame "低量程", Default {
                    n349 = Unbundle By Name(w441) -> ("数组 2[30]"=w440:sgl, "数组 2[31]"=w439:sgl, "数组 2[32]"=w438:sgl)
                  }
                  frame "高量程" {
                    n350 = Unbundle By Name(w445) -> ("数组 2[33]"=w444:sgl, "数组 2[34]"=w443:sgl, "数组 2[35]"=w442:sgl)
                  }
                  frame "0-2量程" {
                    n351 = Unbundle By Name(w449) -> ("数组 2[6]"=w448:sgl, "数组 2[7]"=w447:sgl, "数组 2[8]"=w446:sgl)
                  }
                }
                n352 = Bundle By Name(cluster=cluster{"X":dbl, "b":dbl, "X^2":dbl} {"X"=0.0, "b"=0.0, "X^2"=0.0} ("方程系数"), "X"=w437, "b"=w436, "X^2"=w435) -> (w432:cluster{"X":dbl, "b":dbl, "X^2":dbl})
              }
              frame 7 {
                n353 = local read "量程选择"() -> (w453:enum16{"低量程", "高量程", "0-2量程"})
                n354 = case shown="\"高量程\"" w453 {
                  tunnel: w450 -> [w460 w464 w468]
                  tunnel: [w459 w463 w467] -> w456
                  tunnel: [w458 w462 w466] -> w455
                  tunnel: [w457 w461 w465] -> w454
                  frame "低量程", Default {
                    n355 = Unbundle By Name(w460) -> ("数组 2[36]"=w459:sgl, "数组 2[37]"=w458:sgl, "数组 2[38]"=w457:sgl)
                  }
                  frame "高量程" {
                    n356 = Unbundle By Name(w464) -> ("数组 2[39]"=w463:sgl, "数组 2[40]"=w462:sgl, "数组 2[41]"=w461:sgl)
                  }
                  frame "0-2量程" {
                    n357 = Unbundle By Name(w468) -> ("数组 2[6]"=w467:sgl, "数组 2[7]"=w466:sgl, "数组 2[8]"=w465:sgl)
                  }
                }
                n358 = Bundle By Name(cluster=cluster{"X":dbl, "b":dbl, "X^2":dbl} {"X"=0.0, "b"=0.0, "X^2"=0.0} ("方程系数"), "X"=w456, "b"=w455, "X^2"=w454) -> (w451:cluster{"X":dbl, "b":dbl, "X^2":dbl})
              }
            }
            n359 = local write "方程系数"(w331) -> ()
          }
        }
      }
    }
    n360 = Wait (ms)(milliseconds to wait=u32 1000 ("等待时间（毫秒）")) -> ()  [unwired: 1 out]
  }
  n361 = while {
    tunnel: w64 -> [w620]
    tunnel: w63 -> [w619]
    tunnel: w17 -> [_]
    stop <- FALSE stop-if-true
    # "主循环界面显示"
    n362 = flat-sequence {
      frame #0 {
        # "A，B，K"
        # "CODMn读取状态"
        n363 = global read "COD内部交互全局.vi" "ORP、时间"() -> (w749:u16[])
        n364 = To Word Integer(number=w749) -> (16bit integer=w770:i16[])
        n365 = Split 1D Array(array=w770, index=3 ("索引")) -> (first subarray=w751:i16[], second subarray=w769:i16[])
        n366 = Index Array(array=w751) -> (element #1=w755:i16, element #2=w754:i16, element #3=w753:i16)  [unwired: 3 in]
        n367 = Index Array(array=w769) -> (element #1=w764:i16, element #2=w768:i16, element #3=w767:i16, element #4=w766:i16)  [unwired: 4 in]
        n368 = To Single Precision Float(number=w766) -> (single precision float=w757:sgl)
        n369 = Build Array(w755, w754, w753) -> (w752:i16[])
        n370 = To Single Precision Float(number=w764) -> (single precision float=w763:sgl)
        n371 = To Single Precision Float(number=w768) -> (single precision float=w762:sgl)
        n372 = To Single Precision Float(number=w767) -> (single precision float=w758:sgl)
        n373 = call "HexToDate.vi"("数组"=w752) -> ("DATE"=w756:timestamp[])  [unwired: 10 in]
        n374 = Number To Decimal String(number=w762) -> (decimal integer string=→"ORP-A":string)  [unwired: 1 in]
        n375 = Number To Decimal String(number=w758) -> (decimal integer string=→"ORP-B":string)  [unwired: 1 in]
        n376 = Number To Decimal String(number=w757) -> (decimal integer string=→"ORP-K":string)  [unwired: 1 in]
        n377 = Divide(x=w763, y=sgl 100.0) -> (x/y=→"COD浓度（mg/L)":sgl)
        n378 = Index Array(array=w756) -> (element=w750:timestamp)  [unwired: 1 in]
        n379 = Format Date/Time String(seconds (now)=w750) -> (date/time string=→"数据时间":string)  [unwired: 2 in]
      }
    }
    n380 = flat-sequence {
      frame #0 {
        # "测量状态显示"
        n381 = global read "COD内部交互全局.vi" "测量状态"() -> (w669:u16[])
        n382 = To Word Integer(number=w669) -> (16bit integer=w679:i16[])
        n383 = Index Array(array=w679, index #1=0 ("索引"), index #4=3 ("索引"), index #14=13 ("索引"), index #15=14 ("索引"), index #21=20 ("索引"), index #32=31 ("索引")) -> (element #1=w683:i16, element #2=w682:i16, element #3=w681:i16, element #4=w665:i16, element #5=→"模式（受控）":i16, element #6=→"进样管":i16, element #7=→"高锰酸钾":i16, element #8=→"草酸钠":i16, element #9=→"硫酸":i16, element #10=w678:i16, element #11=w698:i16, element #12=w674:i16, element #13=→"报警数字":i16, element #14=w704:i16, element #15=w689:i16, element #16=→"多列列表框":i16, element #20=→"氢氧化钠":i16, element #21=w662:i16, element #33=→"分":i16, element #34=→"秒":i16)  [unwired: 28 in, 14 out]
        "CODMn工作状态" <- w665
        n384 = global write "COD内部交互全局.vi" "基本量程实时读取"(w662) -> ()
        n385 = Build Array(w683, w682, w681) -> (w684:i16[])
        n386 = To Single Precision Float(number=w678) -> (single precision float=→"实时ORP":sgl)
        n387 = Number To Decimal String(number=w662) -> (decimal integer string=→"基本量程(显示)":string)  [unwired: 1 in]
        n388 = Equal?(x=w674, y=u16 1) -> (x = y?=→"排液标记":bool)
        n389 = Equal?(x=w674, y=u16 2) -> (x = y?=→"断电排液标记":bool)
        n390 = Divide(x=w698, y=u16 10) -> (x/y=→"温度℃":dbl)
        n391 = Divide(x=w704, y=u16 1000) -> (x/y=→"零点滴定值":dbl)
        n392 = Divide(x=w689, y=u16 1000) -> (x/y=→"标度滴定值":dbl)
        n393 = Equal?(x=w665, y=T1."水样测试" ("CODMn工作状态")) -> (x = y?=w663:bool)
        n394 = call "HexToDate.vi"("数组"=w684) -> ("DATE"=w680:timestamp[])  [unwired: 10 in]
        n395 = case shown="真" w663 {
          tunnel: w662 -> [_ w707]
          frame False {
          }
          frame True {
            n396 = global write "CODMn断电保存全局变量.vi" "水样测试量程"(w707) -> ()
          }
        }
        n397 = Index Array(array=w680) -> (element=→"仪器时间":timestamp)  [unwired: 1 in]
      }
    }
    n398 = flat-sequence {
      frame #0 {
        # "报警状态显示"
        n399 = global read "COD内部交互全局.vi" "报警点位"() -> (w722:bool[])
        n400 = Index Array(array=w722, index #1=0 ("索引")) -> (element #1=w719:bool, element #2=w718:bool, element #3=w717:bool, element #4=w716:bool, element #5=w715:bool, element #6=w714:bool, element #7=w713:bool, element #8=w712:bool, element #9=w711:bool, element #11=w710:bool, element #13=w709:bool, element #14=w708:bool)  [unwired: 13 in, 2 out]
        "ORP故障" <- w719
        "温控器故障" <- w718
        "加热故障" <- w711
        "高锰酸钾报警" <- w713
        "草酸钠报警" <- w712
        "测量错误" <- w717
        "校零错误" <- w716
        "校标错误" <- w715
        "进水样超量程" <- w714
        "排液故障" <- w710
        "60分钟超时报警" <- w709
        "进样无液体告警" <- w708
        n401 = Compound Arithmetic op=OR ("复合运算")(w719, w718, w711, w713, w712, w717, w715, w716, w714, w710, w709) -> (→"故障标记":bool)
        n402 = Bundle By Name(cluster=T12 {"ORP故障"=FALSE, "温控器故障"=FALSE, "加热故障"=FALSE, "高锰酸钾报警"=FALSE, "草酸钠报警"=FALSE, "测量错误"=FALSE, "校零错误"=FALSE, "校标错误"=FALSE, " 进水样超量程"=FALSE, "排液阀故障"=FALSE, "60分钟超时报警"=FALSE, "进样无液体报警"=FALSE} ("报警簇"), "ORP故障"=w719, "温控器故障"=w718, "加热故障"=w711, "高锰酸钾报警"=w713, "草酸钠报警"=w712, "测量错误"=w717, "校零错误"=w716, "校标错误"=w715, "进水样超量程"=w714, "排液阀故障"=w710, "60分钟超时报警"=w709, "进样无液体报警"=w708) -> (w720:T12)
        n403 = global write "COD内部交互全局.vi" "报警簇"(w720) -> ()
      }
    }
    n404 = flat-sequence {
      frame #0 {
        # "CODMn读取状态"
        n405 = global read "COD内部交互全局.vi" "温度"() -> (w746:bool[])
        n406 = global read "COD内部交互全局.vi" "M输出点"() -> (w745:bool[])
        n407 = Index Array(array=w746) -> (element=→"加热":bool)  [unwired: 1 in]
        n408 = Index Array(array=w745) -> (element #1=→"搅拌":bool, element #4=→"进水样":bool, element #5=→"进蒸馏水":bool, element #6=→"进标液":bool, element #7=→"进零点核查样":bool, element #8=→"进加标回收样":bool, element #9=→"进高锰酸钾":bool, element #10=→"进草酸钠":bool, element #11=→"进硫酸":bool)  [unwired: 11 in, 2 out]
      }
    }
    n409 = flat-sequence {
      frame #0 {
        # "工作状态显示"
        n410 = local read "CODMn工作状态"() -> (w630:T1)
        n411 = case shown="\"标样校准\"" w630 {
          tunnel: [_ u16 0 ("y") u16 1 ("y") u16 2 ("y") u16 3 ("y") u16 4 ("y") u16 6 ("y") _ u16 7 ("y") u16 8 ("y") u16 5 ("y")] -> w629
          frame "空闲", Default {
          }
          frame "水样测试" {
          }
          frame "标样核查" {
          }
          frame "零点核查" {
          }
          frame "跨度核查" {
          }
          frame "空白测试" {
          }
          frame "平行样测试" {
          }
          frame "质控样" {
          }
          frame "空白校准" {
          }
          frame "标样校准" {
          }
          frame "加标回收" {
          }
        }
        n412 = Equal?(x=w630, y=u16 8) -> (x = y?=→"校零标记":bool)
        n413 = Equal?(x=w630, y=u16 4) -> (x = y?=→"跨度核查标记":bool)
        n414 = Equal?(x=w630, y=u16 0) -> (x = y?=→"待机":bool)
        n415 = Equal?(x=w630, y=u16 3) -> (x = y?=→"零点核查标记":bool)
        n416 = Equal?(x=w630, y=u16 7) -> (x = y?=→"质控样测量":bool)
        n417 = Equal?(x=w630, y=u16 1) -> (x = y?=→"水样测量":bool)
        n418 = Equal?(x=w630, y=u16 2) -> (x = y?=→"标样核查标记":bool)
        n419 = Equal?(x=w630, y=u16 6) -> (x = y?=→"平行样测量":bool)
        n420 = Equal?(x=w630, y=u16 9) -> (x = y?=→"校标标记":bool)
        n421 = Equal?(x=w630, y=u16 5) -> (x = y?=→"空白测试标记":bool)
        n422 = Equal?(x=w630, y=u16 10) -> (x = y?=→"加标回收测量":bool)
        n423 = global write "COD内部交互全局.vi" "测量模式数字"(w629) -> ()
      }
    }
    n424 = Get Date/Time In Seconds() -> (seconds since 1Jan1904=→"系统时间":timestamp)
    n425 = First Call?() -> (First Call?: T/F=w618:bool)
    n426 = Wait (ms)(milliseconds to wait=u32 1000 ("等待时间（毫秒）")) -> ()  [unwired: 1 out]
    n427 = case shown="真" w618 {
      tunnel: w620 -> [w726 w731]
      tunnel: w619 -> [w725 w730]
      tunnel: [w726 w729] -> w616
      tunnel: [w725 w728] -> w615
      frame False {
      }
      frame True {
        n428 = Bundle By Name(cluster=cluster{"命令":string} {"命令"=""} ("元素"), "命令"="CODMn读取参数" ("名称（未命名）")) -> (w734:cluster{"命令":string})
        n429 = Enqueue Element(queue=w731, element=w734, timeout in ms (-1)=1000 ("超时毫秒(-1)"), error in (no error)=w730) -> (queue out=w729:refnum<queue>, error out=w728:errorcluster)  [unwired: 1 out]
      }
    }
    n430 = Get Queue Status(queue=w616, error in (no error)=w615) -> (queue out=w612:refnum<queue>, error out=w611:errorcluster, # elements in queue=w614:i32)  [unwired: 1 in, 5 out]
    n431 = Equal To 0?(x=w614) -> (x = 0?=w613:bool)
    n432 = case shown="真" w613 {
      tunnel: w612 -> [_ w624]
      tunnel: w611 -> [_ w623]
      frame False {
      }
      frame True {
        n433 = Bundle By Name(cluster=cluster{"命令":string} {"命令"=""} ("元素"), "命令"="CODMn读取" ("名称（未命名）")) -> (w626:cluster{"命令":string})
        n434 = Enqueue Element(queue=w624, element=w626, timeout in ms (-1)=1000 ("超时毫秒(-1)"), error in (no error)=w623) -> ()  [unwired: 3 out]
      }
    }
  }
  n435 = while {
    stop <- FALSE stop-if-true
    # "数字键盘输入"
    n436 = event shown="[23] \"泵滴定数1\": 鼠标按下" {
      selector: _ -> [_ _ _ _ _ _ _ _ _ _ _ _ _ _ _ _ _ _ _ _ _ _ _ _ _ _ _ _ _ _]
      dyn-events: _ -> [_ _ _ _ _ _ _ _ _ _ _ _ _ _ _ _ _ _ _ _ _ _ _ _ _ _ _ _ _ _]
      timeout: _ -> [_ _ _ _ _ _ _ _ _ _ _ _ _ _ _ _ _ _ _ _ _ _ _ _ _ _ _ _ _ _]
      event Timeout {
        n437 = event-data() -> ()  [unwired: 1 in, 3 out]
      }
      event "温度": Mouse Down {
        n438 = event-data() -> ()  [unwired: 1 in, 8 out]
        n439 = local read "温度"() -> (w774:dbl)
        n440 = call "数字键盘.vi"("OldNumber"=w774) -> ("NewNumber"=w773:sgl)
        n441 = local write "温度"(w773) -> ()
      }
      event "恒温时间": Mouse Down {
        n442 = event-data() -> ()  [unwired: 1 in, 8 out]
        n443 = local read "恒温时间"() -> (w775:dbl)
        n444 = call "数字键盘.vi"("OldNumber"=w775) -> ("NewNumber"=w776:sgl)
        n445 = local write "恒温时间"(w776) -> ()
      }
      event "标准液浓度": Mouse Down {
        n446 = event-data() -> ()  [unwired: 1 in, 8 out]
        n447 = local read "标准液浓度"() -> (w778:dbl)
        n448 = call "数字键盘.vi"("OldNumber"=w778) -> ("NewNumber"=w777:sgl)
        n449 = local write "标准液浓度"(w777) -> ()
      }
      event "氢氧化钠：": Mouse Down {
        n450 = event-data() -> ()  [unwired: 1 in, 8 out]
        n451 = local read "氢氧化钠："() -> (w779:dbl)
        n452 = call "数字键盘.vi"("OldNumber"=w779) -> ("NewNumber"=w780:sgl)
        n453 = local write "氢氧化钠："(w780) -> ()
      }
      event "水样：": Mouse Down {
        n454 = event-data() -> ()  [unwired: 1 in, 8 out]
        n455 = local read "水样："() -> (w781:dbl)
        n456 = call "数字键盘.vi"("OldNumber"=w781) -> ("NewNumber"=w782:sgl)
        n457 = local write "水样："(w782) -> ()
      }
      event "蒸馏水：": Mouse Down {
        n458 = event-data() -> ()  [unwired: 1 in, 8 out]
        n459 = local read "蒸馏水："() -> (w783:dbl)
        n460 = call "数字键盘.vi"("OldNumber"=w783) -> ("NewNumber"=w784:sgl)
        n461 = local write "蒸馏水："(w784) -> ()
      }
      event "标液：": Mouse Down {
        n462 = event-data() -> ()  [unwired: 1 in, 8 out]
        n463 = local read "标液："() -> (w785:dbl)
        n464 = call "数字键盘.vi"("OldNumber"=w785) -> ("NewNumber"=w786:sgl)
        n465 = local write "标液："(w786) -> ()
      }
      event "零点核查样：": Mouse Down {
        n466 = event-data() -> ()  [unwired: 1 in, 8 out]
        n467 = local read "零点核查样："() -> (w787:dbl)
        n468 = call "数字键盘.vi"("OldNumber"=w787) -> ("NewNumber"=w788:sgl)
        n469 = local write "零点核查样："(w788) -> ()
      }
      event "加标回收样：": Mouse Down {
        n470 = event-data() -> ()  [unwired: 1 in, 8 out]
        n471 = local read "加标回收样："() -> (w789:dbl)
        n472 = call "数字键盘.vi"("OldNumber"=w789) -> ("NewNumber"=w790:sgl)
        n473 = local write "加标回收样："(w790) -> ()
      }
      event "草酸钠": Mouse Down {
        n474 = event-data() -> ()  [unwired: 1 in, 8 out]
        n475 = local read "草酸钠"() -> (w791:dbl)
        n476 = call "数字键盘.vi"("OldNumber"=w791) -> ("NewNumber"=w792:sgl)
        n477 = local write "草酸钠"(w792) -> ()
      }
      event "高锰酸钾": Mouse Down {
        n478 = event-data() -> ()  [unwired: 1 in, 8 out]
        n479 = local read "高锰酸钾"() -> (w793:dbl)
        n480 = call "数字键盘.vi"("OldNumber"=w793) -> ("NewNumber"=w794:sgl)
        n481 = local write "高锰酸钾"(w794) -> ()
      }
      event "硫酸": Mouse Down {
        n482 = event-data() -> ()  [unwired: 1 in, 8 out]
        n483 = local read "硫酸"() -> (w795:dbl)
        n484 = call "数字键盘.vi"("OldNumber"=w795) -> ("NewNumber"=w796:sgl)
        n485 = local write "硫酸"(w796) -> ()
      }
      event "零点泵计量数 2": Mouse Down {
        n486 = event-data() -> ()  [unwired: 1 in, 8 out]
        n487 = local read "零点泵计量数 2"() -> (w797:dbl)
        n488 = call "数字键盘.vi"("OldNumber"=w797) -> ("NewNumber"=w798:sgl)
        n489 = local write "零点泵计量数 2"(w798) -> ()
      }
      event "标度泵计量数 2": Mouse Down {
        n490 = event-data() -> ()  [unwired: 1 in, 8 out]
        n491 = local read "标度泵计量数 2"() -> (w799:dbl)
        n492 = call "数字键盘.vi"("OldNumber"=w799) -> ("NewNumber"=w800:sgl)
        n493 = local write "标度泵计量数 2"(w800) -> ()
      }
      event "高量程稀释倍数:": Mouse Down {
        n494 = event-data() -> ()  [unwired: 1 in, 8 out]
        n495 = local read "高量程稀释倍数:"() -> (w802:i8)
        n496 = call "数字键盘.vi"("OldNumber"=w802) -> ("NewNumber"=w801:sgl)
        n497 = local write "高量程稀释倍数:"(w801) -> ()
      }
      event "低量程稀释倍数:": Mouse Down {
        n498 = event-data() -> ()  [unwired: 1 in, 8 out]
        n499 = local read "低量程稀释倍数:"() -> (w804:i8)
        n500 = call "数字键盘.vi"("OldNumber"=w804) -> ("NewNumber"=w803:sgl)
        n501 = local write "低量程稀释倍数:"(w803) -> ()
      }
      event "浓度1": Mouse Down {
        n502 = event-data() -> ()  [unwired: 1 in, 8 out]
        n503 = local read "浓度1"() -> (w806:dbl)
        n504 = call "数字键盘.vi"("OldNumber"=w806) -> ("NewNumber"=w805:sgl)
        n505 = property on="浓度1" class="DigNum (严格)"("Val(Sgnl)"=w805) -> ()  [unwired: 2 in, 2 out]
      }
      event "浓度2": Mouse Down {
        n506 = event-data() -> ()  [unwired: 1 in, 8 out]
        n507 = local read "浓度2"() -> (w808:dbl)
        n508 = call "数字键盘.vi"("OldNumber"=w808) -> ("NewNumber"=w807:sgl)
        n509 = property on="浓度2" class="DigNum (严格)"("Val(Sgnl)"=w807) -> ()  [unwired: 2 in, 2 out]
      }
      event "浓度3": Mouse Down {
        n510 = event-data() -> ()  [unwired: 1 in, 8 out]
        n511 = local read "浓度3"() -> (w810:dbl)
        n512 = call "数字键盘.vi"("OldNumber"=w810) -> ("NewNumber"=w809:sgl)
        n513 = property on="浓度3" class="DigNum (严格)"("Val(Sgnl)"=w809) -> ()  [unwired: 2 in, 2 out]
      }
      event "浓度4": Mouse Down {
        n514 = event-data() -> ()  [unwired: 1 in, 8 out]
        n515 = local read "浓度4"() -> (w812:dbl)
        n516 = call "数字键盘.vi"("OldNumber"=w812) -> ("NewNumber"=w811:sgl)
        n517 = property on="浓度4" class="DigNum (严格)"("Val(Sgnl)"=w811) -> ()  [unwired: 2 in, 2 out]
      }
      event "浓度5": Mouse Down {
        n518 = event-data() -> ()  [unwired: 1 in, 8 out]
        n519 = local read "浓度5"() -> (w814:dbl)
        n520 = call "数字键盘.vi"("OldNumber"=w814) -> ("NewNumber"=w813:sgl)
        n521 = property on="浓度5" class="DigNum (严格)"("Val(Sgnl)"=w813) -> ()  [unwired: 2 in, 2 out]
      }
      event "跨度液浓度", "零点核查浓度", "标样浓度": Mouse Down {
        n522 = event-data() -> ("CtlRef"=w818:refnum<vi>)  [unwired: 1 in, 7 out]
        n523 = property class="DigNum (严格)"(reference=w818) -> (reference out=w815:refnum<vi>, "Value"=w817:dbl)  [unwired: 1 in, 1 out]
        n524 = call "数字键盘.vi"("OldNumber"=w817) -> ("NewNumber"=w816:sgl)
        n525 = property class="DigNum (严格)"(reference=w815, "Val(Sgnl)"=w816) -> ()  [unwired: 1 in, 2 out]
      }
      event "泵滴定数1": Mouse Down {
        n526 = event-data() -> ()  [unwired: 1 in, 8 out]
        n527 = local read "泵滴定数1"() -> (w820:dbl)
        n528 = call "数字键盘.vi"("OldNumber"=w820) -> ("NewNumber"=w819:sgl)
        n529 = property on="泵滴定数1" class="DigNum (严格)"("Val(Sgnl)"=w819) -> ()  [unwired: 2 in, 2 out]
      }
      event "泵滴定数2": Mouse Down {
        n530 = event-data() -> ()  [unwired: 1 in, 8 out]
        n531 = local read "泵滴定数2"() -> (w822:dbl)
        n532 = call "数字键盘.vi"("OldNumber"=w822) -> ("NewNumber"=w821:sgl)
        n533 = property on="泵滴定数2" class="DigNum (严格)"("Val(Sgnl)"=w821) -> ()  [unwired: 2 in, 2 out]
      }
      event "泵滴定数3": Mouse Down {
        n534 = event-data() -> ()  [unwired: 1 in, 8 out]
        n535 = local read "泵滴定数3"() -> (w824:dbl)
        n536 = call "数字键盘.vi"("OldNumber"=w824) -> ("NewNumber"=w823:sgl)
        n537 = property on="泵滴定数3" class="DigNum (严格)"("Val(Sgnl)"=w823) -> ()  [unwired: 2 in, 2 out]
      }
      event "泵滴定数4": Mouse Down {
        n538 = event-data() -> ()  [unwired: 1 in, 8 out]
        n539 = local read "泵滴定数4"() -> (w826:dbl)
        n540 = call "数字键盘.vi"("OldNumber"=w826) -> ("NewNumber"=w825:sgl)
        n541 = property on="泵滴定数4" class="DigNum (严格)"("Val(Sgnl)"=w825) -> ()  [unwired: 2 in, 2 out]
      }
      event "泵滴定数5": Mouse Down {
        n542 = event-data() -> ()  [unwired: 1 in, 8 out]
        n543 = local read "泵滴定数5"() -> (w828:dbl)
        n544 = call "数字键盘.vi"("OldNumber"=w828) -> ("NewNumber"=w827:sgl)
        n545 = property on="泵滴定数5" class="DigNum (严格)"("Val(Sgnl)"=w827) -> ()  [unwired: 2 in, 2 out]
      }
      event "低切高阈值:", "高切低阈值:": Mouse Down {
        n546 = event-data() -> ("CtlRef"=w832:refnum<vi>)  [unwired: 1 in, 7 out]
        n547 = property class="DigNum (严格)"(reference=w832) -> (reference out=w831:refnum<vi>, "Value"=w830:dbl)  [unwired: 1 in, 1 out]
        n548 = call "数字键盘.vi"("OldNumber"=w830) -> ("NewNumber"=w829:sgl)
        n549 = property class="DigNum (严格)"(reference=w831, "Val(Sgnl)"=w829) -> ()  [unwired: 1 in, 2 out]
      }
      event "远程自动校准浓度": Mouse Down {
        n550 = event-data() -> ("CtlRef"=w833:refnum<vi>)  [unwired: 1 in, 7 out]
        n551 = One Button Dialog(message="请输入其中一个在拟合公式中的非零浓度，用于远程校标！" ("消息")) -> (true=w835:bool)  [unwired: 1 in]
        n552 = case shown="真" w835 {
          tunnel: w833 -> [_ w842]
          frame False {
          }
          frame True {
            n553 = property class="DigNum (严格)"(reference=w842) -> (reference out=w837:refnum<vi>, "Value"=w843:dbl)  [unwired: 1 in, 1 out]
            n554 = global read "COD内部交互全局.vi" "启用的浓度数组"() -> (w839:dbl[])
            n555 = call "数字键盘.vi"("OldNumber"=w843) -> ("NewNumber"=w836:sgl)
            n556 = Search 1D Array(1D array=w839, element=w836) -> (index of element=w840:i32)  [unwired: 1 in]
            n557 = Equal?(x=w840, y=-1) -> (x = y?=w838:bool)
            n558 = case shown="真" w838 {
              tunnel: w837 -> [w845 _]
              tunnel: w836 -> [w844 _]
              frame False {
                n559 = property class="DigNum (严格)"(reference=w845, "Val(Sgnl)"=w844) -> ()  [unwired: 1 in, 2 out]
              }
              frame True {
                n560 = One Button Dialog(message="该浓度不属于校准浓度范围，请重新输入！" ("消息")) -> ()  [unwired: 1 in, 1 out]
              }
            }
          }
        }
      }
    }
  }
  n561 = while {
    tunnel: w64 -> [w848]
    tunnel: w63 -> [w847]
    stop <- FALSE stop-if-true
    # "主线事件"
    n562 = event shown="[17] \"仪器参数\": 值改变" {
      selector: _ -> [_ _ _ _ _ _ _ _ _ _ _ _ _ _ _ _ _ _ _ _ _ _ _ _ _ _ _ _ _ _ _ _ _ _ _]
      dyn-events: _ -> [_ _ _ _ _ _ _ _ _ _ _ _ _ _ _ _ _ _ _ _ _ _ _ _ _ _ _ _ _ _ _ _ _ _ _]
      timeout: _ -> [_ _ _ _ _ _ _ _ _ _ _ _ _ _ _ _ _ _ _ _ _ _ _ _ _ _ _ _ _ _ _ _ _ _ _]
      tunnel: w848 -> [_ _ _ _ _ w937 _ _ _ _ _ _ _ _ _ _ _ _ _ _ _ w1379 _ _ _ w1591 _ _ _ _ w1864 w1871 w1893 w1936 _]
      tunnel: w847 -> [_ _ _ _ _ w936 _ _ _ _ _ _ _ _ _ _ _ _ _ _ _ w1376 _ _ _ w1590 _ _ _ _ w1863 w1870 w1892 w1935 _]
      event "单步启动": Value Change {
        n563 = event-data() -> ()  [unwired: 1 in, 6 out]
        n564 = call "CODMn手动控制框.vi"() -> ()  [unwired: 12 in]
      }
      event "启动": Mouse Down {
        n565 = event-data() -> ()  [unwired: 1 in, 8 out]
        n566 = global read "COD内部交互全局.vi" "基本量程实时读取"() -> (w852:enum16{"L", "H", "AUTO"})
        n567 = call "启动测量模式选择对话框.vi"("量程选择"=w852) -> ("标样浓度输出"=w850:dbl, "量程选择输出"=w851:enum16{"L", "H", "AUTO"}, "启动选择输出"=w856:u16)  [unwired: 8 in]
        n568 = Not Equal?(x=w856, y=u16 8) -> (x != y?=w853:bool)
        n569 = Not Equal?(x=w856, y=u16 7) -> (x != y?=w854:bool)
        n570 = And(x=w854, y=w853) -> (x .and. y?=w858:bool)
        n571 = case shown="真" w858 {
          tunnel: w856 -> [_ w871]
          tunnel: w851 -> [_ w862]
          tunnel: w850 -> [_ w860]
          frame False {
            n572 = One Button Dialog(message="请到校准配置里面进行校准操作！" ("消息")) -> ()  [unwired: 1 in, 1 out]
          }
          frame True {
            n573 = Not Equal?(x=w871, y=u16 9) -> (x != y?=w866:bool)
            n574 = case shown="\"AUTO\"" w862 {
              tunnel: [w872 w876 errorcluster {"status"=FALSE, "code"=0, "source"=""} ("error out")] -> w861
              frame "L", Default {
                n575 = call "CODMnMB_api.vi"("STEP"=enum16{"open", "read", "write", "close"}."write", "values"=u16[] [0], "starting address"=u16 4276) -> ("error out"=w872:errorcluster)  [unwired: 6 in, 2 out]
              }
              frame "H" {
                n576 = call "CODMnMB_api.vi"("STEP"=enum16{"open", "read", "write", "close"}."write", "values"=u16[] [1], "starting address"=u16 4276) -> ("error out"=w876:errorcluster)  [unwired: 6 in, 2 out]
              }
              frame "AUTO" {
              }
            }
            n577 = global write "CODMN外部API.vi" "手动启动CODMn"(w866) -> ()
            n578 = case shown="1" w871 {
              tunnel: [u16 4608 ("address") u16 4608 ("address") u16 4608 ("address") u16 4608 ("address") u16 4608 ("address") u16 4608 ("address") u16 4608 ("address") u16 4608 ("address") u16 4608 ("address") u16 4608 ("address")] -> w864
              tunnel: [u16 1 ("address") u16 2 ("address") u16 3 ("address") u16 4 ("address") u16 5 ("address") u16 7 ("address") u16 6 ("address") u16 8 ("address") u16 9 ("address") u16 0 ("address")] -> w868
              tunnel: w860 -> [_ w884 _ _ _ _ _ _ _ _]
              frame 0 {
              }
              frame 1 {
                n579 = property on="标样浓度" class="DigNum (严格)"("Val(Sgnl)"=w884) -> ()  [unwired: 2 in, 2 out]
              }
              frame 2 {
              }
              frame 3 {
              }
              frame 4 {
              }
              frame 5 {
              }
              frame 6 {
              }
              frame 7 {
              }
              frame 8 {
              }
              frame 9, Default {
              }
            }
            n580 = Insert Into Array(array=u16[] [] ("values"), index=0 ("索引"), new element=w868) -> (w863:u16[])
            n581 = call "CODMnMB_api.vi"("STEP"=enum16{"open", "read", "write", "close"}."write", "Error in"=w861, "values"=w863, "starting address"=w864) -> ()  [unwired: 5 in, 3 out]
          }
        }
      }
      event "停止": Value Change {
        n582 = event-data() -> ()  [unwired: 1 in, 6 out]
        n583 = Two Button Dialog(message="确认是否停止？" ("消息"), 1:"否" ("F按钮名称（“取消”）"), 2:"是" ("T按钮名称（“确定”）")) -> (T button?=w904:bool)
        n584 = case shown="真" w904 {
          frame False {
          }
          frame True {
            n585 = Obtain Notifier(name (unnamed)="CODMn" ("名称（未命名）"), notification data type=FALSE) -> (notifier out=w910:refnum<notifier>, error out=w908:errorcluster)  [unwired: 2 in, 1 out]
            n586 = Send Notification(notification=TRUE ("通知"), notifier=w910, error in (no error)=w908) -> (notifier out=w907:refnum<notifier>, error out=w906:errorcluster)
            n587 = Release Notifier(notifier=w907, error in (no error)=w906) -> ()  [unwired: 1 in, 3 out]
            n588 = call "CODMnMB_api.vi"("STEP"=enum16{"open", "read", "write", "close"}."write", "values"=u16[] [11], "starting address"=u16 4608) -> ()  [unwired: 6 in, 3 out]
          }
        }
      }
      event "手动控制": Value Change {
        n589 = event-data() -> ()  [unwired: 1 in, 6 out]
        n590 = call "数字密码键盘.vi"() -> ("NewNumber"=w916:sgl)  [unwired: 1 in]
        n591 = Equal?(x=w916, y=8.0) -> (x = y?=w917:bool)
        n592 = case shown="假" w917 {
          frame False {
            n593 = call "窗口弹出对话框(子VI).vi"("消息"="密码错误") -> ()  [unwired: 10 in, 1 out]
          }
          frame True {
          }
        }
      }
      event "锁定按钮": Mouse Down {
        n594 = event-data() -> ("CtlRef"=w922:refnum<vi>)  [unwired: 1 in, 7 out]
        n595 = property class="Bool (严格)"(reference=w922) -> ("Value"=w921:bool)  [unwired: 1 in, 2 out]
        n596 = case shown="真" w921 {
          selector: w921 -> [w923 _]
          tunnel: [w923 w927] -> w920
          frame False {
          }
          frame True {
            n597 = call "数字密码键盘.vi"() -> ("NewNumber"=w924:sgl)  [unwired: 1 in]
            n598 = Equal?(x=w924, y=23506.0) -> (x = y?=w928:bool)
            n599 = Equal?(x=w924, y=8.0) -> (x = y?=w925:bool)
            n600 = Or(x=w928, y=w925) -> (x .or. y?=w927:bool)
            n601 = case shown="假" w927 {
              selector: w927 -> [w931 _]
              frame False {
                n602 = local write "锁定按钮"(w931) -> ()
                n603 = One Button Dialog(message="密码错误!" ("消息")) -> ()  [unwired: 1 in, 1 out]
              }
              frame True {
                n604 = One Button Dialog(message="解锁成功!" ("消息")) -> ()  [unwired: 1 in, 1 out]
              }
            }
          }
        }
        "x = y?" <- w920
      }
      event "参数配置": Value Change {
        (unwired) u16 20 ("number of holding registers")
        (unwired) u16 4272 ("starting address")
        n605 = event-data() -> ()  [unwired: 1 in, 6 out]
        n606 = global read "CODMN外部API.vi" "ping"() -> (w935:bool)
        n607 = property on="窗格" class="Pane"("Origin"=T2 {"Horizontal"=0, "Vertical"=650} ("原点")) -> ()  [unwired: 2 in, 2 out]
        n608 = case shown="假" w935 {
          tunnel: [w947 w950] -> w934
          frame False {
            n609 = global read "COD内部交互全局.vi" "配置文件ini"() -> (w949:string)
            n610 = call <vilib>:"Application Directory.vi"() -> ("Application Directory"=w948:path)
            n611 = Build Path(base path=w948, name or relative path=w949) -> (appended path=w947:path)
          }
          frame True {
            n612 = global read "CODMN外部API.vi" "配置文件 path"() -> (w950:path)
          }
        }
        n613 = Bundle By Name(cluster=cluster{"命令":string} {"命令"=""} ("元素"), "命令"="CODMn读取参数" ("名称（未命名）")) -> (w938:cluster{"命令":string})
        n614 = call <vilib>:"Open Config Data.vi"("configuration file path"=w934) -> ("error out"=w944:errorcluster, "refnum"=w941:T4)  [unwired: 8 in, 1 out]
        n615 = Enqueue Element(queue=w937, element=w938, error in (no error)=w936) -> ()  [unwired: 1 in, 3 out]
        n616 = vi-ref "斯坦道CODMn.lvlib:CODMn断电保存全局变量.vi"() -> (w942:refnum<vi>)
        n617 = call <userlib>:"Read Panel from INI__ogtk.vi"("error in (no error)"=w944, "VI ref"=w942, "refnum"=w941) -> ("error out"=w945:errorcluster, "refnum out"=w943:T4)  [unwired: 7 in]
        n618 = call <vilib>:"Close Config Data.vi"("error in (no error)"=w945, "refnum"=w943) -> ("error out"=w933:errorcluster)  [unwired: 8 in, 1 out]
        n619 = call <vilib>:"Clear Errors.vi"("error in (no error)"=w933) -> ()  [unwired: 5 in, 2 out]
      }
      event "保存": Mouse Down {
        n620 = event-data() -> ()  [unwired: 1 in, 8 out]
        n621 = local read "通讯状态"() -> (w951:bool)
        n622 = Two Button Dialog(message="确定保存参数，保存参数将会替换原有参数！" ("消息")) -> (T button?=w953:bool)  [unwired: 2 in]
        n623 = case shown="真" w953 {
          tunnel: w951 -> [_ w954]
          frame False {
          }
          frame True {
            n624 = case shown="真" w954 {
              frame False {
                n625 = One Button Dialog(message="保存失败，当前无通讯！" ("消息")) -> ()  [unwired: 1 in, 1 out]
              }
              frame True {
                n626 = One Button Dialog(message="参数保存成功！" ("消息")) -> ()  [unwired: 1 in, 1 out]
                n627 = Build Array("采水泵进样时间/s:", "采水泵润洗时间/s:", "采水泵沉淀时间/s:", "采水泵排液时间/s:") -> (w957:i32[])
                n628 = call "CODMnMB_api.vi"("STEP"=enum16{"open", "read", "write", "close"}."write", "values"="保存参数", "starting address"=u16 4272) -> ("error out"=w963:errorcluster)  [unwired: 6 in, 2 out]
                n629 = call "CODMnMB_api.vi"("STEP"=enum16{"open", "read", "write", "close"}."write", "Error in"=w963, "values"=w957, "starting address"=u16 5596) -> ()  [unwired: 5 in, 3 out]
              }
            }
          }
        }
      }
      event "常规版/认证版": Value Change {
        n630 = event-data() -> ()  [unwired: 1 in, 6 out]
        n631 = flat-sequence {
          frame #0 {
            n632 = global write "CODMn断电保存全局变量.vi" "常规版/认证版"("常规版/认证版") -> ()
          }
          frame #1 {
            n633 = call "配置文件保存.vi"() -> ()  [unwired: 12 in]
          }
        }
      }
      event "校准配置": Value Change {
        w978 = "量程选择" ("section")
        n634 = event-data() -> ()  [unwired: 1 in, 6 out]
        n635 = global read "CODMN外部API.vi" "ping"() -> (w982:bool)
        n636 = property on="窗格" class="Pane"("Origin"=T2 {"Horizontal"=0, "Vertical"=1300} ("原点")) -> ()  [unwired: 2 in, 2 out]
        n637 = case shown="假" w982 {
          tunnel: [w1060 w1063] -> w981
          frame False {
            n638 = global read "COD内部交互全局.vi" "配置文件ini"() -> (w1062:string)
            n639 = call <vilib>:"Application Directory.vi"() -> ("Application Directory"=w1061:path)
            n640 = Build Path(base path=w1061, name or relative path=w1062) -> (appended path=w1060:path)
          }
          frame True {
            n641 = global read "CODMN外部API.vi" "配置文件 path"() -> (w1063:path)
          }
        }
        n642 = call <vilib>:"Open Config Data.vi"("configuration file path"=w981) -> ("error out"=w999:errorcluster, "refnum"=w1000:T4)  [unwired: 8 in, 1 out]
        n643 = call-poly <vilib>:"Read Key.vi"("section"="CODMn模型选择" ("key"), "error in (no error)"=w999, "key"="线性和多项式", "refnum"=w1000) -> ("error out"=w996:errorcluster, "value"=w998:i32, "refnum out"=w997:T4)  [unwired: 4 in, 1 out]
        n644 = local write "模型"(w998) -> ()
        n645 = call-poly <vilib>:"Read Key.vi"("section"="标线选择", "error in (no error)"=w996, "key"="选用水样", "refnum"=w997) -> ("error out"=w979:errorcluster, "value"=w983:i32, "refnum out"=w980:T4)  [unwired: 4 in, 1 out]
        n646 = local write "选用水样"(w983) -> ()
        n647 = case shown="0, 默认" w983 {
          tunnel: ["葡萄糖标线" ("section") "草酸钠标线" ("section")] -> w1005
          frame 0, Default {
          }
          frame 1 {
          }
        }
        n648 = call-poly <vilib>:"Read Key.vi"("section"=w978, "error in (no error)"=w979, "key"=w978, "refnum"=w980) -> ("error out"=w976:errorcluster, "value"=w975:i32, "refnum out"=w977:T4)  [unwired: 4 in, 1 out]
        n649 = local write "量程选择"(w975) -> ()
        n650 = case shown="2" w975 {
          tunnel: ["低量程" "高量程" "0-2量程"] -> w1004
          frame 0, Default {
          }
          frame 1 {
          }
          frame 2 {
          }
        }
        n651 = Concatenate Strings(w1005, w1004) -> (w1003:string)
        n652 = call-poly <vilib>:"Read Key.vi"("section"=w1003, "error in (no error)"=w976, "key"="浓度1", "refnum"=w977) -> ("error out"=w1030:errorcluster, "value"=w1028:dbl, "refnum out"=w1029:T4)  [unwired: 4 in, 1 out]
        n653 = local write "浓度1"(w1028) -> ()
        n654 = call-poly <vilib>:"Read Key.vi"("section"=w1003, "error in (no error)"=w1030, "key"="浓度2", "refnum"=w1029) -> ("error out"=w1044:errorcluster, "value"=w1031:dbl, "refnum out"=w1043:T4)  [unwired: 4 in, 1 out]
        n655 = local write "浓度2"(w1031) -> ()
        n656 = call-poly <vilib>:"Read Key.vi"("section"=w1003, "error in (no error)"=w1044, "key"="浓度3", "refnum"=w1043) -> ("error out"=w1045:errorcluster, "value"=w1033:dbl, "refnum out"=w1042:T4)  [unwired: 4 in, 1 out]
        n657 = local write "浓度3"(w1033) -> ()
        n658 = call-poly <vilib>:"Read Key.vi"("section"=w1003, "error in (no error)"=w1045, "key"="泵滴定数1", "refnum"=w1042) -> ("error out"=w1046:errorcluster, "value"=w1035:dbl, "refnum out"=w1041:T4)  [unwired: 4 in, 1 out]
        n659 = local write "泵滴定数1"(w1035) -> ()
        n660 = call-poly <vilib>:"Read Key.vi"("section"=w1003, "error in (no error)"=w1046, "key"="泵滴定数2", "refnum"=w1041) -> ("error out"=w1040:errorcluster, "value"=w1038:dbl, "refnum out"=w1047:T4)  [unwired: 4 in, 1 out]
        n661 = local write "泵滴定数2"(w1038) -> ()
        n662 = call-poly <vilib>:"Read Key.vi"("section"=w1003, "error in (no error)"=w1040, "key"="泵滴定数3", "refnum"=w1047) -> ("error out"=w1052:errorcluster, "value"=w1051:dbl, "refnum out"=w1048:T4)  [unwired: 4 in, 1 out]
        n663 = local write "泵滴定数3"(w1051) -> ()
        n664 = call-poly <vilib>:"Read Key.vi"("section"=w1003, "error in (no error)"=w1052, "key"="浓度4", "refnum"=w1048) -> ("error out"=w1053:errorcluster, "value"=w989:dbl, "refnum out"=w1049:T4)  [unwired: 4 in, 1 out]
        n665 = local write "浓度4"(w989) -> ()
        n666 = call-poly <vilib>:"Read Key.vi"("section"=w1003, "error in (no error)"=w1053, "key"="浓度5", "refnum"=w1049) -> ("error out"=w994:errorcluster, "value"=w988:dbl, "refnum out"=w995:T4)  [unwired: 4 in, 1 out]
        n667 = local write "浓度5"(w988) -> ()
        n668 = call-poly <vilib>:"Read Key.vi"("section"=w1003, "error in (no error)"=w994, "key"="泵滴定数4", "refnum"=w995) -> ("error out"=w1054:errorcluster, "value"=w987:dbl, "refnum out"=w1050:T4)  [unwired: 4 in, 1 out]
        n669 = local write "泵滴定数4"(w987) -> ()
        n670 = call-poly <vilib>:"Read Key.vi"("section"=w1003, "error in (no error)"=w1054, "key"="泵滴定数5", "refnum"=w1050) -> ("error out"=w992:errorcluster, "value"=w986:dbl, "refnum out"=w993:T4)  [unwired: 4 in, 1 out]
        n671 = local write "泵滴定数5"(w986) -> ()
        n672 = call-poly <vilib>:"Read Key.vi"("section"=w1003, "error in (no error)"=w992, "key"="当前选用的校准", "refnum"=w993) -> ("error out"=w1024:errorcluster, "refnum out"=w1025:T4)  [unwired: 4 in, 2 out]
        n673 = call-poly <vilib>:"Read Key.vi"("section"=w1003, "error in (no error)"=w1024, "key"="启用1", "refnum"=w1025) -> ("error out"=w1021:errorcluster, "value"=w1010:bool, "refnum out"=w1022:T4)  [unwired: 4 in, 1 out]
        n674 = local write "启用1"(w1010) -> ()
        n675 = call-poly <vilib>:"Read Key.vi"("section"=w1003, "error in (no error)"=w1021, "key"="启用2", "refnum"=w1022) -> ("error out"=w1019:errorcluster, "value"=w1009:bool, "refnum out"=w1020:T4)  [unwired: 4 in, 1 out]
        n676 = local write "启用2"(w1009) -> ()
        n677 = call-poly <vilib>:"Read Key.vi"("section"=w1003, "error in (no error)"=w1019, "key"="启用3", "refnum"=w1020) -> ("error out"=w1017:errorcluster, "value"=w1008:bool, "refnum out"=w1018:T4)  [unwired: 4 in, 1 out]
        n678 = local write "启用3"(w1008) -> ()
        n679 = call-poly <vilib>:"Read Key.vi"("section"=w1003, "error in (no error)"=w1017, "key"="启用4", "refnum"=w1018) -> ("error out"=w1015:errorcluster, "value"=w985:bool, "refnum out"=w1016:T4)  [unwired: 4 in, 1 out]
        n680 = local write "启用4"(w985) -> ()
        n681 = call-poly <vilib>:"Read Key.vi"("section"=w1003, "error in (no error)"=w1015, "key"="启用5", "refnum"=w1016) -> ("error out"=w990:errorcluster, "value"=w984:bool, "refnum out"=w991:T4)  [unwired: 4 in, 1 out]
        n682 = local write "启用5"(w984) -> ()
        n683 = call <vilib>:"Close Config Data.vi"("error in (no error)"=w990, "refnum"=w991) -> ("error out"=w969:errorcluster, "file path"=w970:path)  [unwired: 8 in]
        n684 = Open/Create/Replace File(file path (use dialog)=w970, error in=w969) -> (refnum out=w972:refnum<file>, error out=w971:errorcluster)  [unwired: 4 in, 1 out]
        n685 = Flush File(refnum=w972, error in=w971) -> (refnum out=w973:refnum<file>, error out=w974:errorcluster)
        n686 = Close File(refnum=w973, error in=w974) -> ()  [unwired: 2 out]
      }
      event "选用水样": Value Change {
        (unwired) "浓度6" ("key")
        n687 = event-data() -> ()  [unwired: 1 in, 6 out]
        n688 = local read "量程选择"() -> (w1097:enum16{"低量程", "高量程", "0-2量程"})
        n689 = property on="窗格" class="Pane"("Origin"=T2 {"Horizontal"=0, "Vertical"=1300} ("原点")) -> ()  [unwired: 2 in, 2 out]
        n690 = case shown="\"葡萄糖\", 默认" "选用水样" {
          tunnel: ["葡萄糖标线" ("section") "草酸钠标线" ("section")] -> w1099
          frame "葡萄糖", Default {
          }
          frame "草酸钠" {
          }
        }
        n691 = global read "CODMN外部API.vi" "ping"() -> (w1083:bool)
        n692 = case shown="\"0-2量程\"" w1097 {
          tunnel: ["低量程" "高量程" "0-2量程"] -> w1098
          frame "低量程", Default {
          }
          frame "高量程" {
          }
          frame "0-2量程" {
          }
        }
        n693 = case shown="假" w1083 {
          tunnel: [w1152 w1155] -> w1082
          frame False {
            n694 = global read "COD内部交互全局.vi" "配置文件ini"() -> (w1154:string)
            n695 = call <vilib>:"Application Directory.vi"() -> ("Application Directory"=w1153:path)
            n696 = Build Path(base path=w1153, name or relative path=w1154) -> (appended path=w1152:path)
          }
          frame True {
            n697 = global read "CODMN外部API.vi" "配置文件 path"() -> (w1155:path)
          }
        }
        n698 = Concatenate Strings(w1099, w1098) -> (w1096:string)
        n699 = call <vilib>:"Open Config Data.vi"("configuration file path"=w1082) -> ("error out"=w1078:errorcluster, "refnum"=w1079:T4)  [unwired: 8 in, 1 out]
        n700 = call-poly <vilib>:"Write Key.vi"("section"="标线选择", "error in (no error)"=w1078, "value"="选用水样", "key"="选用水样", "refnum"=w1079) -> ("error out"=w1075:errorcluster, "refnum out"=w1076:T4)  [unwired: 4 in, 1 out]
        n701 = call-poly <vilib>:"Read Key.vi"("section"=w1096, "error in (no error)"=w1075, "key"="浓度1", "refnum"=w1076) -> ("error out"=w1122:errorcluster, "value"=w1120:dbl, "refnum out"=w1121:T4)  [unwired: 4 in, 1 out]
        n702 = local write "浓度1"(w1120) -> ()
        n703 = call-poly <vilib>:"Read Key.vi"("section"=w1096, "error in (no error)"=w1122, "key"="浓度2", "refnum"=w1121) -> ("error out"=w1136:errorcluster, "value"=w1123:dbl, "refnum out"=w1135:T4)  [unwired: 4 in, 1 out]
        n704 = local write "浓度2"(w1123) -> ()
        n705 = call-poly <vilib>:"Read Key.vi"("section"=w1096, "error in (no error)"=w1136, "key"="浓度3", "refnum"=w1135) -> ("error out"=w1137:errorcluster, "value"=w1125:dbl, "refnum out"=w1134:T4)  [unwired: 4 in, 1 out]
        n706 = local write "浓度3"(w1125) -> ()
        n707 = call-poly <vilib>:"Read Key.vi"("section"=w1096, "error in (no error)"=w1137, "key"="泵滴定数1", "refnum"=w1134) -> ("error out"=w1138:errorcluster, "value"=w1127:dbl, "refnum out"=w1133:T4)  [unwired: 4 in, 1 out]
        n708 = local write "泵滴定数1"(w1127) -> ()
        n709 = call-poly <vilib>:"Read Key.vi"("section"=w1096, "error in (no error)"=w1138, "key"="泵滴定数2", "refnum"=w1133) -> ("error out"=w1132:errorcluster, "value"=w1130:dbl, "refnum out"=w1139:T4)  [unwired: 4 in, 1 out]
        n710 = local write "泵滴定数2"(w1130) -> ()
        n711 = call-poly <vilib>:"Read Key.vi"("section"=w1096, "error in (no error)"=w1132, "key"="泵滴定数3", "refnum"=w1139) -> ("error out"=w1144:errorcluster, "value"=w1143:dbl, "refnum out"=w1140:T4)  [unwired: 4 in, 1 out]
        n712 = local write "泵滴定数3"(w1143) -> ()
        n713 = call-poly <vilib>:"Read Key.vi"("section"=w1096, "error in (no error)"=w1144, "key"="浓度4", "refnum"=w1140) -> ("error out"=w1145:errorcluster, "value"=w1091:dbl, "refnum out"=w1141:T4)  [unwired: 4 in, 1 out]
        n714 = local write "浓度4"(w1091) -> ()
        n715 = call-poly <vilib>:"Read Key.vi"("section"=w1096, "error in (no error)"=w1145, "key"="浓度5", "refnum"=w1141) -> ("error out"=w1094:errorcluster, "value"=w1090:dbl, "refnum out"=w1095:T4)  [unwired: 4 in, 1 out]
        n716 = local write "浓度5"(w1090) -> ()
        n717 = call-poly <vilib>:"Read Key.vi"("section"=w1096, "error in (no error)"=w1094, "key"="泵滴定数4", "refnum"=w1095) -> ("error out"=w1146:errorcluster, "value"=w1089:dbl, "refnum out"=w1142:T4)  [unwired: 4 in, 1 out]
        n718 = local write "泵滴定数4"(w1089) -> ()
        n719 = call-poly <vilib>:"Read Key.vi"("section"=w1096, "error in (no error)"=w1146, "key"="泵滴定数5", "refnum"=w1142) -> ("error out"=w1092:errorcluster, "value"=w1088:dbl, "refnum out"=w1093:T4)  [unwired: 4 in, 1 out]
        n720 = local write "泵滴定数5"(w1088) -> ()
        n721 = call-poly <vilib>:"Read Key.vi"("section"=w1096, "error in (no error)"=w1092, "key"="当前选用的校准", "refnum"=w1093) -> ("error out"=w1116:errorcluster, "refnum out"=w1117:T4)  [unwired: 4 in, 2 out]
        n722 = call-poly <vilib>:"Read Key.vi"("section"=w1096, "error in (no error)"=w1116, "key"="启用1", "refnum"=w1117) -> ("error out"=w1113:errorcluster, "value"=w1102:bool, "refnum out"=w1114:T4)  [unwired: 4 in, 1 out]
        n723 = local write "启用1"(w1102) -> ()
        n724 = call-poly <vilib>:"Read Key.vi"("section"=w1096, "error in (no error)"=w1113, "key"="启用2", "refnum"=w1114) -> ("error out"=w1111:errorcluster, "value"=w1101:bool, "refnum out"=w1112:T4)  [unwired: 4 in, 1 out]
        n725 = local write "启用2"(w1101) -> ()
        n726 = call-poly <vilib>:"Read Key.vi"("section"=w1096, "error in (no error)"=w1111, "key"="启用3", "refnum"=w1112) -> ("error out"=w1109:errorcluster, "value"=w1100:bool, "refnum out"=w1110:T4)  [unwired: 4 in, 1 out]
        n727 = local write "启用3"(w1100) -> ()
        n728 = call-poly <vilib>:"Read Key.vi"("section"=w1096, "error in (no error)"=w1109, "key"="启用4", "refnum"=w1110) -> ("error out"=w1107:errorcluster, "value"=w1085:bool, "refnum out"=w1108:T4)  [unwired: 4 in, 1 out]
        n729 = local write "启用4"(w1085) -> ()
        n730 = call-poly <vilib>:"Read Key.vi"("section"=w1096, "error in (no error)"=w1107, "key"="启用5", "refnum"=w1108) -> ("error out"=w1086:errorcluster, "value"=w1084:bool, "refnum out"=w1087:T4)  [unwired: 4 in, 1 out]
        n731 = local write "启用5"(w1084) -> ()
        n732 = call <vilib>:"Close Config Data.vi"("error in (no error)"=w1086, "refnum"=w1087) -> ("error out"=w1069:errorcluster, "file path"=w1070:path)  [unwired: 8 in]
        n733 = Open/Create/Replace File(file path (use dialog)=w1070, error in=w1069) -> (refnum out=w1072:refnum<file>, error out=w1071:errorcluster)  [unwired: 4 in, 1 out]
        n734 = Flush File(refnum=w1072, error in=w1071) -> (refnum out=w1073:refnum<file>, error out=w1074:errorcluster)
        n735 = Close File(refnum=w1073, error in=w1074) -> ()  [unwired: 2 out]
      }
      event "量程选择": Value Change {
        w1172 = "量程选择" ("section")
        n736 = event-data() -> ()  [unwired: 1 in, 6 out]
        n737 = local read "选用水样"() -> (w1190:enum16{"葡萄糖", "草酸钠"})
        n738 = property on="窗格" class="Pane"("Origin"=T2 {"Horizontal"=0, "Vertical"=1300} ("原点")) -> ()  [unwired: 2 in, 2 out]
        n739 = case shown="\"葡萄糖\", 默认" w1190 {
          tunnel: ["葡萄糖标线" ("section") "草酸钠标线" ("section")] -> w1189
          frame "葡萄糖", Default {
          }
          frame "草酸钠" {
          }
        }
        n740 = case shown="\"0-2量程\"" "量程选择" {
          tunnel: ["低量程" "高量程" "0-2量程"] -> w1187
          frame "低量程", Default {
          }
          frame "高量程" {
          }
          frame "0-2量程" {
          }
        }
        n741 = global read "CODMN外部API.vi" "ping"() -> (w1174:bool)
        n742 = case shown="假" w1174 {
          tunnel: [w1243 w1246] -> w1173
          frame False {
            n743 = global read "COD内部交互全局.vi" "配置文件ini"() -> (w1245:string)
            n744 = call <vilib>:"Application Directory.vi"() -> ("Application Directory"=w1244:path)
            n745 = Build Path(base path=w1244, name or relative path=w1245) -> (appended path=w1243:path)
          }
          frame True {
            n746 = global read "CODMN外部API.vi" "配置文件 path"() -> (w1246:path)
          }
        }
        n747 = Concatenate Strings(w1189, w1187) -> (w1188:string)
        n748 = call <vilib>:"Open Config Data.vi"("configuration file path"=w1173) -> ("error out"=w1171:errorcluster, "refnum"=w1170:T4)  [unwired: 8 in, 1 out]
        n749 = call-poly <vilib>:"Write Key.vi"("section"=w1172, "error in (no error)"=w1171, "value"="量程选择", "key"=w1172, "refnum"=w1170) -> ("error out"=w1167:errorcluster, "refnum out"=w1169:T4)  [unwired: 4 in, 1 out]
        n750 = call-poly <vilib>:"Read Key.vi"("section"=w1188, "error in (no error)"=w1167, "key"="浓度1", "refnum"=w1169) -> ("error out"=w1213:errorcluster, "value"=w1211:dbl, "refnum out"=w1212:T4)  [unwired: 4 in, 1 out]
        n751 = local write "浓度1"(w1211) -> ()
        n752 = call-poly <vilib>:"Read Key.vi"("section"=w1188, "error in (no error)"=w1213, "key"="浓度2", "refnum"=w1212) -> ("error out"=w1227:errorcluster, "value"=w1214:dbl, "refnum out"=w1226:T4)  [unwired: 4 in, 1 out]
        n753 = local write "浓度2"(w1214) -> ()
        n754 = call-poly <vilib>:"Read Key.vi"("section"=w1188, "error in (no error)"=w1227, "key"="浓度3", "refnum"=w1226) -> ("error out"=w1228:errorcluster, "value"=w1216:dbl, "refnum out"=w1225:T4)  [unwired: 4 in, 1 out]
        n755 = local write "浓度3"(w1216) -> ()
        n756 = call-poly <vilib>:"Read Key.vi"("section"=w1188, "error in (no error)"=w1228, "key"="泵滴定数1", "refnum"=w1225) -> ("error out"=w1229:errorcluster, "value"=w1218:dbl, "refnum out"=w1224:T4)  [unwired: 4 in, 1 out]
        n757 = local write "泵滴定数1"(w1218) -> ()
        n758 = call-poly <vilib>:"Read Key.vi"("section"=w1188, "error in (no error)"=w1229, "key"="泵滴定数2", "refnum"=w1224) -> ("error out"=w1223:errorcluster, "value"=w1221:dbl, "refnum out"=w1230:T4)  [unwired: 4 in, 1 out]
        n759 = local write "泵滴定数2"(w1221) -> ()
        n760 = call-poly <vilib>:"Read Key.vi"("section"=w1188, "error in (no error)"=w1223, "key"="泵滴定数3", "refnum"=w1230) -> ("error out"=w1235:errorcluster, "value"=w1234:dbl, "refnum out"=w1231:T4)  [unwired: 4 in, 1 out]
        n761 = local write "泵滴定数3"(w1234) -> ()
        n762 = call-poly <vilib>:"Read Key.vi"("section"=w1188, "error in (no error)"=w1235, "key"="浓度4", "refnum"=w1231) -> ("error out"=w1236:errorcluster, "value"=w1178:dbl, "refnum out"=w1232:T4)  [unwired: 4 in, 1 out]
        n763 = local write "浓度4"(w1178) -> ()
        n764 = call-poly <vilib>:"Read Key.vi"("section"=w1188, "error in (no error)"=w1236, "key"="浓度5", "refnum"=w1232) -> ("error out"=w1185:errorcluster, "value"=w1177:dbl, "refnum out"=w1186:T4)  [unwired: 4 in, 1 out]
        n765 = local write "浓度5"(w1177) -> ()
        n766 = call-poly <vilib>:"Read Key.vi"("section"=w1188, "error in (no error)"=w1185, "key"="泵滴定数4", "refnum"=w1186) -> ("error out"=w1237:errorcluster, "value"=w1176:dbl, "refnum out"=w1233:T4)  [unwired: 4 in, 1 out]
        n767 = local write "泵滴定数4"(w1176) -> ()
        n768 = call-poly <vilib>:"Read Key.vi"("section"=w1188, "error in (no error)"=w1237, "key"="泵滴定数5", "refnum"=w1233) -> ("error out"=w1183:errorcluster, "value"=w1175:dbl, "refnum out"=w1184:T4)  [unwired: 4 in, 1 out]
        n769 = local write "泵滴定数5"(w1175) -> ()
        n770 = call-poly <vilib>:"Read Key.vi"("section"=w1188, "error in (no error)"=w1183, "key"="当前选用的校准", "refnum"=w1184) -> ("error out"=w1207:errorcluster, "refnum out"=w1208:T4)  [unwired: 4 in, 2 out]
        n771 = call-poly <vilib>:"Read Key.vi"("section"=w1188, "error in (no error)"=w1207, "key"="启用1", "refnum"=w1208) -> ("error out"=w1204:errorcluster, "value"=w1193:bool, "refnum out"=w1205:T4)  [unwired: 4 in, 1 out]
        n772 = local write "启用1"(w1193) -> ()
        n773 = call-poly <vilib>:"Read Key.vi"("section"=w1188, "error in (no error)"=w1204, "key"="启用2", "refnum"=w1205) -> ("error out"=w1202:errorcluster, "value"=w1192:bool, "refnum out"=w1203:T4)  [unwired: 4 in, 1 out]
        n774 = local write "启用2"(w1192) -> ()
        n775 = call-poly <vilib>:"Read Key.vi"("section"=w1188, "error in (no error)"=w1202, "key"="启用3", "refnum"=w1203) -> ("error out"=w1200:errorcluster, "value"=w1191:bool, "refnum out"=w1201:T4)  [unwired: 4 in, 1 out]
        n776 = local write "启用3"(w1191) -> ()
        n777 = call-poly <vilib>:"Read Key.vi"("section"=w1188, "error in (no error)"=w1200, "key"="启用4", "refnum"=w1201) -> ("error out"=w1198:errorcluster, "value"=w1180:bool, "refnum out"=w1199:T4)  [unwired: 4 in, 1 out]
        n778 = local write "启用4"(w1180) -> ()
        n779 = call-poly <vilib>:"Read Key.vi"("section"=w1188, "error in (no error)"=w1198, "key"="启用5", "refnum"=w1199) -> ("error out"=w1181:errorcluster, "value"=w1179:bool, "refnum out"=w1182:T4)  [unwired: 4 in, 1 out]
        n780 = local write "启用5"(w1179) -> ()
        n781 = call <vilib>:"Close Config Data.vi"("error in (no error)"=w1181, "refnum"=w1182) -> ("error out"=w1161:errorcluster, "file path"=w1162:path)  [unwired: 8 in]
        n782 = Open/Create/Replace File(file path (use dialog)=w1162, error in=w1161) -> (refnum out=w1164:refnum<file>, error out=w1163:errorcluster)  [unwired: 4 in, 1 out]
        n783 = Flush File(refnum=w1164, error in=w1163) -> (refnum out=w1165:refnum<file>, error out=w1166:errorcluster)
        n784 = Close File(refnum=w1165, error in=w1166) -> ()  [unwired: 2 out]
      }
      event "返回": Value Change {
        w1273 = "CODMn" ("section")
        n785 = event-data() -> ()  [unwired: 1 in, 6 out]
        n786 = property on="窗格" class="Pane"("Origin"=T2 {"Horizontal"=0, "Vertical"=0} ("原点")) -> ()  [unwired: 2 in, 2 out]
        n787 = global read "CODMN外部API.vi" "ping"() -> (w1259:bool)
        n788 = case shown="假" w1259 {
          tunnel: [w1324 w1327] -> w1258
          frame False {
            n789 = global read "COD内部交互全局.vi" "配置文件ini"() -> (w1326:string)
            n790 = call <vilib>:"Application Directory.vi"() -> ("Application Directory"=w1325:path)
            n791 = Build Path(base path=w1325, name or relative path=w1326) -> (appended path=w1324:path)
          }
          frame True {
            n792 = global read "CODMN外部API.vi" "配置文件 path"() -> (w1327:path)
          }
        }
        n793 = call <vilib>:"Open Config Data.vi"("configuration file path"=w1258) -> ("error out"=w1322:errorcluster, "refnum"=w1323:T4)  [unwired: 8 in, 1 out]
        n794 = local read "浓度1"() -> (w1320:dbl)
        n795 = call-poly <vilib>:"Write Key.vi"("section"=w1273, "error in (no error)"=w1322, "value"=w1320, "key"="浓度1", "refnum"=w1323) -> ("error out"=w1319:errorcluster, "refnum out"=w1318:T4)  [unwired: 4 in, 1 out]
        n796 = local read "浓度2"() -> (w1304:dbl)
        n797 = call-poly <vilib>:"Write Key.vi"("section"=w1273, "error in (no error)"=w1319, "value"=w1304, "key"="浓度2", "refnum"=w1318) -> ("error out"=w1317:errorcluster, "refnum out"=w1316:T4)  [unwired: 4 in, 1 out]
        n798 = local read "浓度3"() -> (w1300:dbl)
        n799 = local read "泵滴定数1"() -> (w1298:dbl)
        n800 = call-poly <vilib>:"Write Key.vi"("section"=w1273, "error in (no error)"=w1317, "value"=w1300, "key"="浓度3", "refnum"=w1316) -> ("error out"=w1315:errorcluster, "refnum out"=w1314:T4)  [unwired: 4 in, 1 out]
        n801 = local read "泵滴定数2"() -> (w1296:dbl)
        n802 = call-poly <vilib>:"Write Key.vi"("section"=w1273, "error in (no error)"=w1315, "value"=w1298, "key"="泵滴定数1", "refnum"=w1314) -> ("error out"=w1313:errorcluster, "refnum out"=w1312:T4)  [unwired: 4 in, 1 out]
        n803 = local read "泵滴定数3"() -> (w1294:dbl)
        n804 = call-poly <vilib>:"Write Key.vi"("section"=w1273, "error in (no error)"=w1313, "value"=w1296, "key"="泵滴定数2", "refnum"=w1312) -> ("error out"=w1311:errorcluster, "refnum out"=w1310:T4)  [unwired: 4 in, 1 out]
        n805 = call-poly <vilib>:"Write Key.vi"("section"=w1273, "error in (no error)"=w1311, "value"=w1294, "key"="泵滴定数3", "refnum"=w1310) -> ("error out"=w1309:errorcluster, "refnum out"=w1308:T4)  [unwired: 4 in, 1 out]
        n806 = local read "浓度4"() -> (w1261:dbl)
        n807 = call-poly <vilib>:"Write Key.vi"("section"=w1273, "error in (no error)"=w1309, "value"=w1261, "key"="浓度4", "refnum"=w1308) -> ("error out"=w1302:errorcluster, "refnum out"=w1303:T4)  [unwired: 4 in, 1 out]
        n808 = local read "浓度5"() -> (w1260:dbl)
        n809 = local read "泵滴定数4"() -> (w1262:dbl)
        n810 = call-poly <vilib>:"Write Key.vi"("section"=w1273, "error in (no error)"=w1302, "value"=w1260, "key"="浓度5", "refnum"=w1303) -> ("error out"=w1270:errorcluster, "refnum out"=w1271:T4)  [unwired: 4 in, 1 out]
        n811 = local read "泵滴定数5"() -> (w1263:dbl)
        n812 = call-poly <vilib>:"Write Key.vi"("section"=w1273, "error in (no error)"=w1270, "value"=w1262, "key"="泵滴定数4", "refnum"=w1271) -> ("error out"=w1307:errorcluster, "refnum out"=w1306:T4)  [unwired: 4 in, 1 out]
        n813 = call-poly <vilib>:"Write Key.vi"("section"=w1273, "error in (no error)"=w1307, "value"=w1263, "key"="泵滴定数5", "refnum"=w1306) -> ("error out"=w1268:errorcluster, "refnum out"=w1269:T4)  [unwired: 4 in, 1 out]
        n814 = local read "启用1"() -> (w1282:bool)
        n815 = call-poly <vilib>:"Write Key.vi"("section"=w1273, "error in (no error)"=w1268, "value"=w1282, "key"="启用1", "refnum"=w1269) -> ("error out"=w1278:errorcluster, "refnum out"=w1281:T4)  [unwired: 4 in, 1 out]
        n816 = local read "启用2"() -> (w1279:bool)
        n817 = call-poly <vilib>:"Write Key.vi"("section"=w1273, "error in (no error)"=w1278, "value"=w1279, "key"="启用2", "refnum"=w1281) -> ("error out"=w1289:errorcluster, "refnum out"=w1288:T4)  [unwired: 4 in, 1 out]
        n818 = local read "启用3"() -> (w1277:bool)
        n819 = call-poly <vilib>:"Write Key.vi"("section"=w1273, "error in (no error)"=w1289, "value"=w1277, "key"="启用3", "refnum"=w1288) -> ("error out"=w1287:errorcluster, "refnum out"=w1286:T4)  [unwired: 4 in, 1 out]
        n820 = local read "启用4"() -> (w1265:bool)
        n821 = call-poly <vilib>:"Write Key.vi"("section"=w1273, "error in (no error)"=w1287, "value"=w1265, "key"="启用4", "refnum"=w1286) -> ("error out"=w1285:errorcluster, "refnum out"=w1284:T4)  [unwired: 4 in, 1 out]
        n822 = local read "启用5"() -> (w1264:bool)
        n823 = call-poly <vilib>:"Write Key.vi"("section"=w1273, "error in (no error)"=w1285, "value"=w1264, "key"="启用5", "refnum"=w1284) -> ("error out"=w1266:errorcluster, "refnum out"=w1267:T4)  [unwired: 4 in, 1 out]
        n824 = call <vilib>:"Close Config Data.vi"("error in (no error)"=w1266, "refnum"=w1267) -> ("error out"=w1252:errorcluster, "file path"=w1253:path)  [unwired: 8 in]
        n825 = Open/Create/Replace File(file path (use dialog)=w1253, error in=w1252) -> (refnum out=w1255:refnum<file>, error out=w1254:errorcluster)  [unwired: 4 in, 1 out]
        n826 = Flush File(refnum=w1255, error in=w1254) -> (refnum out=w1256:refnum<file>, error out=w1257:errorcluster)
        n827 = Close File(refnum=w1256, error in=w1257) -> ()  [unwired: 2 out]
      }
      event "关闭", "关闭 2", "关闭 3": Value Change {
        n828 = event-data() -> ()  [unwired: 1 in, 6 out]
        n829 = property on="窗格" class="Pane"("Origin"=T2 {"Horizontal"=0, "Vertical"=0} ("原点")) -> ()  [unwired: 2 in, 2 out]
      }
      event Application Instance Close {
        n830 = event-data() -> ()  [unwired: 1 in, 4 out]
      }
      event "时间校准": Value Change {
        n831 = event-data() -> ()  [unwired: 1 in, 6 out]
        n832 = Get Date/Time In Seconds() -> (seconds since 1Jan1904=w1337:timestamp)
        n833 = Build Array(w1337) -> (w1336:timestamp[])
        n834 = call "DateToHex.vi"("DATE"=w1336) -> ("数组"=w1334:u16[])  [unwired: 10 in]
        n835 = Insert Into Array(array=u16[] [1] ("values"), index=1 ("索引"), new element=w1334) -> (w1330:u16[])
        n836 = call "CODMnMB_api.vi"("STEP"=enum16{"open", "read", "write", "close"}."write", "values"=w1330, "starting address"=u16 4612) -> ("error out"=w1329:errorcluster)  [unwired: 6 in, 2 out]
        n837 = call <vilib>:"Clear Errors.vi"("error in (no error)"=w1329) -> ()  [unwired: 5 in, 2 out]
      }
      event "故障清除": Value Change {
        n838 = event-data() -> ()  [unwired: 1 in, 6 out]
        n839 = call "CODMnMB_api.vi"("STEP"=enum16{"open", "read", "write", "close"}."write", "values"=u16[] [1], "starting address"=u16 4611) -> ()  [unwired: 6 in, 3 out]
      }
      event "定时启动": Mouse Down {
        n840 = event-data() -> ()  [unwired: 1 in, 8 out]
        n841 = flat-sequence {
          frame #0 {
            n842 = global read "CODMn断电保存全局变量.vi" "间隔已启动次数"() -> (w1342:dbl)
            n843 = global read "CODMn断电保存全局变量.vi" "间隔设定次数"() -> (w1341:dbl)
            n844 = global read "CODMn断电保存全局变量.vi" "定时控制"() -> (w1344:T10)
            n845 = call "周期设置.vi"("间隔已启动次数"=w1342, "间隔设定启动次数"=w1341, "定时控制输入"=w1344) -> ("定时控制输出"=w1343:T13)  [unwired: 8 in]
            n846 = global write "CODMn断电保存全局变量.vi" "定时控制"(w1343) -> ()
          }
          frame #1 {
            n847 = call "配置文件保存.vi"() -> ()  [unwired: 12 in]
          }
        }
      }
      event "仪器参数": Value Change {
        n848 = event-data() -> ()  [unwired: 1 in, 6 out]
        n849 = global read "CODMn断电保存全局变量.vi" "CODMn仪器参数"() -> (w1345:T14)
        n850 = call "仪器参数设置.vi"("氨氮仪器参数"=w1345) -> ("仪器参数设置输出"=w1346:T15)  [unwired: 10 in]
        n851 = Unbundle By Name(w1346) -> ("确定"=w1347:bool)
        n852 = case shown="真" w1347 {
          tunnel: w1346 -> [_ w1349]
          tunnel: w1345 -> [_ w1348]
          frame False {
          }
          frame True {
            n853 = flat-sequence {
              tunnel: w1349 -> [w1366]
              tunnel: w1348 -> [w1365]
              frame #0 {
                n854 = Unbundle By Name(w1366) -> ("测量量程"=w1364:dbl, "测量精度"=w1363:dbl, "测量间隔"=w1362:dbl, "消解温度"=w1361:dbl, "消解时长"=w1360:dbl, "空白校准时间"=w1359:timestamp, "曲线截距"=w1358:dbl, "曲线斜率"=w1357:dbl, "测量检出限"=w1356:dbl, "测量信号值"=w1355:dbl, "线性相关系数"=w1354:dbl, "二次多项式系数"=w1353:dbl, "标样校准时间"=w1352:timestamp, "稀释倍数"=w1351:dbl)
                n855 = Bundle By Name(cluster=w1365, "测量量程"=w1364, "测量精度"=w1363, "测量间隔"=w1362, "消解温度"=w1361, "消解时长"=w1360, "空白校准时间"=w1359, "曲线截距"=w1358, "曲线斜率"=w1357, "测量检出限"=w1356, "测量信号值"=w1355, "线性相关系数"=w1354, "二次多项式系数"=w1353, "标样校准时间"=w1352, "稀释倍数"=w1351) -> (w1350:T14)
                n856 = global write "CODMn断电保存全局变量.vi" "CODMn仪器参数"(w1350) -> ()
              }
              frame #1 {
                n857 = call "配置文件保存.vi"() -> ()  [unwired: 12 in]
              }
            }
          }
        }
      }
      event "远程自动校准浓度", "远程校准量程": Value Change {
        n858 = event-data() -> ()  [unwired: 1 in, 6 out]
        n859 = flat-sequence {
          frame #0 {
            n860 = global write "CODMn断电保存全局变量.vi" "远程校准量程"("远程校准量程") -> ()
            n861 = global write "CODMn断电保存全局变量.vi" "远程自动校准浓度"("远程自动校准浓度") -> ()
          }
          frame #1 {
            n862 = call "配置文件保存.vi"() -> ()  [unwired: 12 in]
          }
        }
      }
      event "测量模式(公式)": Value Change {
        n863 = event-data() -> ()  [unwired: 1 in, 6 out]
        n864 = flat-sequence {
          frame #0 {
            n865 = global write "CODMn断电保存全局变量.vi" "测量模式(公式)"("测量模式(公式)") -> ()
          }
          frame #1 {
            n866 = call "配置文件保存.vi"() -> ()  [unwired: 12 in]
          }
        }
      }
      event "跨度量程选择", "跨度液浓度", "零点核查量程选择", "零点核查浓度", "标样浓度", "标样核查量程选择": Value Change {
        n867 = event-data() -> ()  [unwired: 1 in, 6 out]
        n868 = flat-sequence {
          frame #0 {
            n869 = global write "CODMn断电保存全局变量.vi" "标样浓度"("标样浓度") -> ()
            n870 = global write "CODMn断电保存全局变量.vi" "零点核查浓度"("零点核查浓度") -> ()
            n871 = global write "CODMn断电保存全局变量.vi" "跨度液浓度"("跨度液浓度") -> ()
            n872 = global write "CODMn断电保存全局变量.vi" "CODMn跨度量程选择"("跨度量程选择") -> ()
            n873 = global write "CODMn断电保存全局变量.vi" "标样核查量程选择"("标样核查量程选择") -> ()
            n874 = global write "CODMn断电保存全局变量.vi" "零点核查量程选择"("零点核查量程选择") -> ()
          }
          frame #1 {
            n875 = call "配置文件保存.vi"() -> ()  [unwired: 12 in]
          }
        }
      }
      event "校准1", "校准2", "校准3", "校准4", "校准5": Value Change {
        n876 = event-data() -> ()  [unwired: 1 in, 6 out]
        n877 = flat-sequence {
          tunnel: w1379 -> [w1388]
          tunnel: [w1388] -> w1381
          tunnel: w1376 -> [w1387]
          tunnel: [w1387] -> w1378
          tunnel: w1381 -> [w1424]
          tunnel: [w1424] -> w1380
          tunnel: w1378 -> [w1423]
          tunnel: [w1423] -> w1377
          tunnel: w1380 -> [w1451]
          tunnel: w1377 -> [w1450]
          frame #0 {
            n878 = Build Array("校准1", "校准2", "校准3", "校准4", "校准5") -> (w1391:bool[])
            n879 = for {
              tunnel: w1391 -> [w1406] mode=indexing
              tunnel: [w1398] -> w1382
              i -> [w1399]
              n880 = case shown="4" w1399 {
                tunnel: ["浓度1" "浓度2" "浓度3" "浓度4" "浓度5"] -> w1402
                frame 0, Default {
                }
                frame 1 {
                }
                frame 2 {
                }
                frame 3 {
                }
                frame 4 {
                }
              }
              n881 = Multiply(x=w1402, y=100.0) -> (x*y=w1400:dbl)
              n882 = Insert Into Array(array=u16[] [] ("values"), index=0 ("索引"), new element=w1400) -> (w1403:u16[])
              n883 = case shown="真" w1406 {
                tunnel: w1403 -> [_ w1415]
                tunnel: w1399 -> [_ w1417]
                tunnel: [_ w1412] -> w1398
                frame False {
                }
                frame True {
                  n884 = Increment(x=w1417) -> (x+1=w1413:i32)
                  n885 = global write "COD内部交互全局.vi" "当前校准"(w1413) -> ()
                  n886 = call "CODMnMB_api.vi"("STEP"=enum16{"open", "read", "write", "close"}."write", "values"=w1415, "starting address"=u16 4274) -> ("error out"=w1412:errorcluster)  [unwired: 6 in, 2 out]
                }
              }
            }
            n887 = local read "量程选择"() -> (w1384:enum16{"低量程", "高量程", "0-2量程"})
            n888 = case shown="\"高量程\"" w1384 {
              tunnel: [u16[] [0] ("values") u16[] [1] ("values") u16[] [0] ("values")] -> w1383
              frame "低量程", Default {
              }
              frame "高量程" {
              }
              frame "0-2量程" {
              }
            }
            n889 = call "CODMnMB_api.vi"("STEP"=enum16{"open", "read", "write", "close"}."write", "Error in"=w1382, "values"=w1383, "starting address"=u16 4276) -> ()  [unwired: 5 in, 3 out]
          }
          frame #1 {
            n890 = global read "COD内部交互全局.vi" "当前校准"() -> (w1425:i32)
            n891 = case shown="5" w1425 {
              tunnel: [w1433 w1434 w1435 w1436 w1437] -> w1421
              frame 1, Default {
                n892 = local read "浓度1"() -> (w1433:dbl)
              }
              frame 2 {
                n893 = local read "浓度2"() -> (w1434:dbl)
              }
              frame 3 {
                n894 = local read "浓度3"() -> (w1435:dbl)
              }
              frame 4 {
                n895 = local read "浓度4"() -> (w1436:dbl)
              }
              frame 5 {
                n896 = local read "浓度5"() -> (w1437:dbl)
              }
            }
            n897 = Number To Decimal String(number=w1421) -> (decimal integer string=w1420:string)  [unwired: 1 in]
            n898 = Concatenate Strings("仪器校准中!\n当前校准浓度为:", w1420, "mg/L" ("字符串")) -> (w1418:string)
            n899 = Not Equal To 0?(x=w1421) -> (x != 0?=w1429:bool)
            n900 = global write "COD内部交互全局.vi" "校准内容显示"(w1418) -> ()
            n901 = case shown="真" w1429 {
              tunnel: [u16 8 ("address") u16 9 ("address")] -> w1432
              tunnel: ["校零" ("测量模式") "校标" ("测量模式")] -> _
              frame False {
              }
              frame True {
              }
            }
            n902 = Insert Into Array(array=u16[] [] ("values"), index=0 ("索引"), new element=w1432) -> (w1426:u16[])
            n903 = call "CODMnMB_api.vi"("STEP"=enum16{"open", "read", "write", "close"}."write", "values"=w1426, "starting address"=u16 4608 ("address")) -> ()  [unwired: 6 in, 3 out]
          }
          frame #2 {
            n904 = local read "选用水样"() -> (w1459:enum16{"葡萄糖", "草酸钠"})
            n905 = global read "CODMN外部API.vi" "ping"() -> (w1449:bool)
            n906 = case shown="假" w1449 {
              tunnel: [w1467 w1470] -> w1448
              frame False {
                n907 = global read "COD内部交互全局.vi" "配置文件ini"() -> (w1469:string)
                n908 = call <vilib>:"Application Directory.vi"() -> ("Application Directory"=w1468:path)
                n909 = Build Path(base path=w1468, name or relative path=w1469) -> (appended path=w1467:path)
              }
              frame True {
                n910 = global read "CODMN外部API.vi" "配置文件 path"() -> (w1470:path)
              }
            }
            n911 = local read "量程选择"() -> (w1458:enum16{"低量程", "高量程", "0-2量程"})
            n912 = case shown="\"葡萄糖\", 默认" w1459 {
              tunnel: ["葡萄糖标线" ("section") "草酸钠标线" ("section")] -> w1460
              frame "葡萄糖", Default {
              }
              frame "草酸钠" {
              }
            }
            n913 = Bundle By Name(cluster=cluster{"命令":string} {"命令"=""} ("元素"), "命令"="CODMn读取参数" ("名称（未命名）")) -> (w1455:cluster{"命令":string})
            n914 = case shown="\"0-2量程\"" w1458 {
              tunnel: ["低量程" "高量程" "0-2量程"] -> w1461
              frame "低量程", Default {
              }
              frame "高量程" {
              }
              frame "0-2量程" {
              }
            }
            n915 = global read "COD内部交互全局.vi" "当前校准"() -> (w1456:i32)
            n916 = Enqueue Element(queue=w1451, element=w1455, timeout in ms (-1)=1000 ("超时毫秒(-1)"), error in (no error)=w1450) -> ()  [unwired: 3 out]
            n917 = Concatenate Strings(w1460, w1461) -> (w1457:string)
            n918 = call <vilib>:"Open Config Data.vi"("configuration file path"=w1448) -> ("error out"=w1465:errorcluster, "refnum"=w1466:T4)  [unwired: 8 in, 1 out]
            n919 = call-poly <vilib>:"Write Key.vi"("section"=w1457, "error in (no error)"=w1465, "value"=w1456, "key"="当前选用的校准" ("section"), "refnum"=w1466) -> ("error out"=w1462:errorcluster, "refnum out"=w1463:T4)  [unwired: 4 in, 1 out]
            n920 = call <vilib>:"Close Config Data.vi"("error in (no error)"=w1462, "refnum"=w1463) -> ("error out"=w1442:errorcluster, "file path"=w1443:path)  [unwired: 8 in]
            n921 = Open/Create/Replace File(file path (use dialog)=w1443, error in=w1442) -> (refnum out=w1445:refnum<file>, error out=w1444:errorcluster)  [unwired: 4 in, 1 out]
            n922 = Flush File(refnum=w1445, error in=w1444) -> (refnum out=w1446:refnum<file>, error out=w1447:errorcluster)
            n923 = Close File(refnum=w1446, error in=w1447) -> ()  [unwired: 2 out]
          }
        }
      }
      event "水样量程选择:", "低切高阈值:", "高切低阈值:": Value Change {
        n924 = event-data() -> ()  [unwired: 1 in, 6 out]
        n925 = flat-sequence {
          frame #0 {
            n926 = global write "CODMn断电保存全局变量.vi" "高切低阈值:"("高切低阈值:") -> ()
            n927 = global write "CODMn断电保存全局变量.vi" "自动切换量程:"("水样量程选择:") -> ()
            n928 = global write "CODMn断电保存全局变量.vi" "低切高阈值:"("低切高阈值:") -> ()
          }
          frame #1 {
            n929 = call "配置文件保存.vi"() -> ()  [unwired: 12 in]
          }
        }
      }
      event "模型": Value Change {
        n930 = event-data() -> ()  [unwired: 1 in, 6 out]
        n931 = global read "CODMN外部API.vi" "ping"() -> (w1486:bool)
        n932 = case shown="假" w1486 {
          tunnel: [w1494 w1497] -> w1485
          frame False {
            n933 = global read "COD内部交互全局.vi" "配置文件ini"() -> (w1496:string)
            n934 = call <vilib>:"Application Directory.vi"() -> ("Application Directory"=w1495:path)
            n935 = Build Path(base path=w1495, name or relative path=w1496) -> (appended path=w1494:path)
          }
          frame True {
            n936 = global read "CODMN外部API.vi" "配置文件 path"() -> (w1497:path)
          }
        }
        n937 = call <vilib>:"Open Config Data.vi"("configuration file path"=w1485) -> ("error out"=w1492:errorcluster, "refnum"=w1493:T4)  [unwired: 8 in, 1 out]
        n938 = local read "模型"() -> (w1487:enum32{"线性", "多项式"})
        n939 = call-poly <vilib>:"Write Key.vi"("section"="CODMn模型选择" ("key"), "error in (no error)"=w1492, "value"=w1487, "key"="线性和多项式", "refnum"=w1493) -> ("error out"=w1488:errorcluster, "refnum out"=w1489:T4)  [unwired: 4 in, 1 out]
        n940 = call <vilib>:"Close Config Data.vi"("error in (no error)"=w1488, "refnum"=w1489) -> ("error out"=w1479:errorcluster, "file path"=w1480:path)  [unwired: 8 in]
        n941 = Open/Create/Replace File(file path (use dialog)=w1480, error in=w1479) -> (refnum out=w1482:refnum<file>, error out=w1481:errorcluster)  [unwired: 4 in, 1 out]
        n942 = Flush File(refnum=w1482, error in=w1481) -> (refnum out=w1483:refnum<file>, error out=w1484:errorcluster)
        n943 = Close File(refnum=w1483, error in=w1484) -> ()  [unwired: 2 out]
      }
      event "浓度1", "浓度2", "浓度3", "泵滴定数1", "泵滴定数2", "泵滴定数3", "启用1", "启用2", "启用3", "浓度4", "浓度5", "泵滴定数4", "泵滴定数5", "启用4", "启用5": Value Change {
        n944 = event-data() -> ()  [unwired: 1 in, 6 out]
        n945 = local read "选用水样"() -> (w1521:enum16{"葡萄糖", "草酸钠"})
        n946 = local read "量程选择"() -> (w1520:enum16{"低量程", "高量程", "0-2量程"})
        n947 = case shown="\"葡萄糖\", 默认" w1521 {
          tunnel: ["葡萄糖标线" ("section") "草酸钠标线" ("section")] -> w1527
          frame "葡萄糖", Default {
          }
          frame "草酸钠" {
          }
        }
        n948 = case shown="\"0-2量程\"" w1520 {
          tunnel: ["低量程" "高量程" "0-2量程"] -> w1518
          frame "低量程", Default {
          }
          frame "高量程" {
          }
          frame "0-2量程" {
          }
        }
        n949 = global read "CODMN外部API.vi" "ping"() -> (w1505:bool)
        n950 = case shown="假" w1505 {
          tunnel: [w1578 w1581] -> w1504
          frame False {
            n951 = global read "COD内部交互全局.vi" "配置文件ini"() -> (w1580:string)
            n952 = call <vilib>:"Application Directory.vi"() -> ("Application Directory"=w1579:path)
            n953 = Build Path(base path=w1579, name or relative path=w1580) -> (appended path=w1578:path)
          }
          frame True {
            n954 = global read "CODMN外部API.vi" "配置文件 path"() -> (w1581:path)
          }
        }
        n955 = Concatenate Strings(w1527, w1518) -> (w1519:string)
        n956 = call <vilib>:"Open Config Data.vi"("configuration file path"=w1504) -> ("error out"=w1576:errorcluster, "refnum"=w1577:T4)  [unwired: 8 in, 1 out]
        n957 = local read "浓度1"() -> (w1574:dbl)
        n958 = call-poly <vilib>:"Write Key.vi"("section"=w1519, "error in (no error)"=w1576, "value"=w1574, "key"="浓度1", "refnum"=w1577) -> ("error out"=w1573:errorcluster, "refnum out"=w1572:T4)  [unwired: 4 in, 1 out]
        n959 = local read "浓度2"() -> (w1558:dbl)
        n960 = call-poly <vilib>:"Write Key.vi"("section"=w1519, "error in (no error)"=w1573, "value"=w1558, "key"="浓度2", "refnum"=w1572) -> ("error out"=w1571:errorcluster, "refnum out"=w1570:T4)  [unwired: 4 in, 1 out]
        n961 = local read "浓度3"() -> (w1554:dbl)
        n962 = local read "泵滴定数1"() -> (w1552:dbl)
        n963 = call-poly <vilib>:"Write Key.vi"("section"=w1519, "error in (no error)"=w1571, "value"=w1554, "key"="浓度3", "refnum"=w1570) -> ("error out"=w1569:errorcluster, "refnum out"=w1568:T4)  [unwired: 4 in, 1 out]
        n964 = local read "泵滴定数2"() -> (w1550:dbl)
        n965 = call-poly <vilib>:"Write Key.vi"("section"=w1519, "error in (no error)"=w1569, "value"=w1552, "key"="泵滴定数1", "refnum"=w1568) -> ("error out"=w1567:errorcluster, "refnum out"=w1566:T4)  [unwired: 4 in, 1 out]
        n966 = local read "泵滴定数3"() -> (w1548:dbl)
        n967 = call-poly <vilib>:"Write Key.vi"("section"=w1519, "error in (no error)"=w1567, "value"=w1550, "key"="泵滴定数2", "refnum"=w1566) -> ("error out"=w1565:errorcluster, "refnum out"=w1564:T4)  [unwired: 4 in, 1 out]
        n968 = call-poly <vilib>:"Write Key.vi"("section"=w1519, "error in (no error)"=w1565, "value"=w1548, "key"="泵滴定数3", "refnum"=w1564) -> ("error out"=w1563:errorcluster, "refnum out"=w1562:T4)  [unwired: 4 in, 1 out]
        n969 = local read "浓度4"() -> (w1517:dbl)
        n970 = call-poly <vilib>:"Write Key.vi"("section"=w1519, "error in (no error)"=w1563, "value"=w1517, "key"="浓度4", "refnum"=w1562) -> ("error out"=w1556:errorcluster, "refnum out"=w1557:T4)  [unwired: 4 in, 1 out]
        n971 = local read "浓度5"() -> (w1516:dbl)
        n972 = local read "泵滴定数4"() -> (w1513:dbl)
        n973 = call-poly <vilib>:"Write Key.vi"("section"=w1519, "error in (no error)"=w1556, "value"=w1516, "key"="浓度5", "refnum"=w1557) -> ("error out"=w1514:errorcluster, "refnum out"=w1515:T4)  [unwired: 4 in, 1 out]
        n974 = local read "泵滴定数5"() -> (w1512:dbl)
        n975 = call-poly <vilib>:"Write Key.vi"("section"=w1519, "error in (no error)"=w1514, "value"=w1513, "key"="泵滴定数4", "refnum"=w1515) -> ("error out"=w1561:errorcluster, "refnum out"=w1560:T4)  [unwired: 4 in, 1 out]
        n976 = call-poly <vilib>:"Write Key.vi"("section"=w1519, "error in (no error)"=w1561, "value"=w1512, "key"="泵滴定数5", "refnum"=w1560) -> ("error out"=w1510:errorcluster, "refnum out"=w1511:T4)  [unwired: 4 in, 1 out]
        n977 = local read "启用1"() -> (w1536:bool)
        n978 = call-poly <vilib>:"Write Key.vi"("section"=w1519, "error in (no error)"=w1510, "value"=w1536, "key"="启用1", "refnum"=w1511) -> ("error out"=w1532:errorcluster, "refnum out"=w1535:T4)  [unwired: 4 in, 1 out]
        n979 = local read "启用2"() -> (w1533:bool)
        n980 = call-poly <vilib>:"Write Key.vi"("section"=w1519, "error in (no error)"=w1532, "value"=w1533, "key"="启用2", "refnum"=w1535) -> ("error out"=w1543:errorcluster, "refnum out"=w1542:T4)  [unwired: 4 in, 1 out]
        n981 = local read "启用3"() -> (w1531:bool)
        n982 = call-poly <vilib>:"Write Key.vi"("section"=w1519, "error in (no error)"=w1543, "value"=w1531, "key"="启用3", "refnum"=w1542) -> ("error out"=w1541:errorcluster, "refnum out"=w1540:T4)  [unwired: 4 in, 1 out]
        n983 = local read "启用4"() -> (w1506:bool)
        n984 = call-poly <vilib>:"Write Key.vi"("section"=w1519, "error in (no error)"=w1541, "value"=w1506, "key"="启用4", "refnum"=w1540) -> ("error out"=w1539:errorcluster, "refnum out"=w1538:T4)  [unwired: 4 in, 1 out]
        n985 = local read "启用5"() -> (w1507:bool)
        n986 = local read "选用水样"() -> (w1526:enum16{"葡萄糖", "草酸钠"})
        n987 = call-poly <vilib>:"Write Key.vi"("section"=w1519, "error in (no error)"=w1539, "value"=w1507, "key"="启用5", "refnum"=w1538) -> ("error out"=w1508:errorcluster, "refnum out"=w1509:T4)  [unwired: 4 in, 1 out]
        n988 = call-poly <vilib>:"Write Key.vi"("section"="标线选择", "error in (no error)"=w1508, "value"=w1526, "key"="选用水样", "refnum"=w1509) -> ("error out"=w1523:errorcluster, "refnum out"=w1524:T4)  [unwired: 4 in, 1 out]
        n989 = call <vilib>:"Close Config Data.vi"("error in (no error)"=w1523, "refnum"=w1524) -> ("error out"=w1498:errorcluster, "file path"=w1499:path)  [unwired: 8 in]
        n990 = Open/Create/Replace File(file path (use dialog)=w1499, error in=w1498) -> (refnum out=w1501:refnum<file>, error out=w1500:errorcluster)  [unwired: 4 in, 1 out]
        n991 = Flush File(refnum=w1501, error in=w1500) -> (refnum out=w1502:refnum<file>, error out=w1503:errorcluster)
        n992 = Close File(refnum=w1502, error in=w1503) -> ()  [unwired: 2 out]
      }
      event "读取": Value Change {
        (unwired) u16 94 ("number of holding registers")
        (unwired) u16 4616 ("starting address")
        n993 = event-data() -> ()  [unwired: 1 in, 6 out]
        n994 = Bundle By Name(cluster=cluster{"命令":string} {"命令"=""} ("元素"), "命令"="CODMn读取公式" ("名称（未命名）")) -> (w1587:cluster{"命令":string})
        n995 = Enqueue Element(queue=w1591, element=w1587, error in (no error)=w1590) -> ()  [unwired: 1 in, 3 out]
      }
      event "写入": Mouse Down {
        n996 = event-data() -> ()  [unwired: 1 in, 8 out]
        n997 = Two Button Dialog(message="是否将上方方程系数K、B、X^2的值写入，写入会覆盖原有公式！" ("消息")) -> (T button?=w1592:bool)  [unwired: 2 in]
        n998 = case shown="真" w1592 {
          frame False {
          }
          frame True {
            n999 = local read "模型"() -> (w1603:enum32{"线性", "多项式"})
            n1000 = case shown="\"多项式\"" w1603 {
              tunnel: [w1632 w1676] -> w1601
              tunnel: [w1631 w1675] -> w1600
              frame "线性", Default {
                (unwired) "线性" ("table输入")
                n1001 = local read "测量模式(公式)"() -> (w1633:u16)
                n1002 = case shown="1" w1633 {
                  tunnel: [u16 4626 ("starting address") w1640 w1645 w1650 w1655 w1660 w1665 w1670] -> w1632
                  frame 0, Default {
                  }
                  frame 1 {
                    n1003 = local read "量程选择"() -> (w1639:enum16{"低量程", "高量程", "0-2量程"})
                    n1004 = case shown="\"低量程\", 默认" w1639 {
                      tunnel: [u16 4626 ("starting address") u16 4632 ("starting address") u16 4638 ("starting address")] -> w1640
                      frame "低量程", Default {
                      }
                      frame "高量程" {
                      }
                      frame "0-2量程" {
                      }
                    }
                  }
                  frame 2 {
                    n1005 = local read "量程选择"() -> (w1644:enum16{"低量程", "高量程", "0-2量程"})
                    n1006 = case shown="\"低量程\", 默认" w1644 {
                      tunnel: [u16 4638 ("starting address") u16 4644 ("starting address") u16 4638 ("starting address")] -> w1645
                      frame "低量程", Default {
                      }
                      frame "高量程" {
                      }
                      frame "0-2量程" {
                      }
                    }
                  }
                  frame 3 {
                    n1007 = local read "量程选择"() -> (w1649:enum16{"低量程", "高量程", "0-2量程"})
                    n1008 = case shown="\"低量程\", 默认" w1649 {
                      tunnel: [u16 4650 ("starting address") u16 4656 ("starting address") u16 4638 ("starting address")] -> w1650
                      frame "低量程", Default {
                      }
                      frame "高量程" {
                      }
                      frame "0-2量程" {
                      }
                    }
                  }
                  frame 4 {
                    n1009 = local read "量程选择"() -> (w1654:enum16{"低量程", "高量程", "0-2量程"})
                    n1010 = case shown="\"低量程\", 默认" w1654 {
                      tunnel: [u16 4662 ("starting address") u16 4668 ("starting address") u16 4638 ("starting address")] -> w1655
                      frame "低量程", Default {
                      }
                      frame "高量程" {
                      }
                      frame "0-2量程" {
                      }
                    }
                  }
                  frame 5 {
                    n1011 = local read "量程选择"() -> (w1659:enum16{"低量程", "高量程", "0-2量程"})
                    n1012 = case shown="\"低量程\", 默认" w1659 {
                      tunnel: [u16 4674 ("starting address") u16 4680 ("starting address") u16 4638 ("starting address")] -> w1660
                      frame "低量程", Default {
                      }
                      frame "高量程" {
                      }
                      frame "0-2量程" {
                      }
                    }
                  }
                  frame 6 {
                    n1013 = local read "量程选择"() -> (w1664:enum16{"低量程", "高量程", "0-2量程"})
                    n1014 = case shown="\"低量程\", 默认" w1664 {
                      tunnel: [u16 4686 ("starting address") u16 4692 ("starting address") u16 4638 ("starting address")] -> w1665
                      frame "低量程", Default {
                      }
                      frame "高量程" {
                      }
                      frame "0-2量程" {
                      }
                    }
                  }
                  frame 7 {
                    n1015 = local read "量程选择"() -> (w1669:enum16{"低量程", "高量程", "0-2量程"})
                    n1016 = case shown="\"低量程\", 默认" w1669 {
                      tunnel: [u16 4698 ("starting address") u16 4704 ("starting address") u16 4638 ("starting address")] -> w1670
                      frame "低量程", Default {
                      }
                      frame "高量程" {
                      }
                      frame "0-2量程" {
                      }
                    }
                  }
                }
                n1017 = local read "K"() -> (w1637:dbl)
                n1018 = local read "b"() -> (w1636:dbl)
                n1019 = Build Array(w1637, w1636, 0.0 ("元素")) -> (w1635:dbl[])
                n1020 = call "浮点转CDAB整形cod.vi"("浮点数"=w1635) -> ("CDAB整形输出"=w1631:u16[])  [unwired: 10 in]
              }
              frame "多项式" {
                (unwired) "多项式" ("table输入")
                # "b,k,c"
                n1021 = local read "多项式系数"() -> (w1681:dbl[])
                n1022 = local read "测量模式(公式)"() -> (w1677:u16)
                n1023 = Index Array(array=w1681) -> (element #1=w1679:dbl, element #2=w1674:dbl, element #3=w1678:dbl)  [unwired: 3 in]
                n1024 = case shown="1" w1677 {
                  tunnel: [u16 4626 ("starting address") w1684 w1689 w1694 w1699 w1704 w1709 w1714] -> w1676
                  frame 0, Default {
                  }
                  frame 1 {
                    n1025 = local read "量程选择"() -> (w1683:enum16{"低量程", "高量程", "0-2量程"})
                    n1026 = case shown="\"低量程\", 默认" w1683 {
                      tunnel: [u16 4626 ("starting address") u16 4632 ("starting address") u16 4638 ("starting address")] -> w1684
                      frame "低量程", Default {
                      }
                      frame "高量程" {
                      }
                      frame "0-2量程" {
                      }
                    }
                  }
                  frame 2 {
                    n1027 = local read "量程选择"() -> (w1688:enum16{"低量程", "高量程", "0-2量程"})
                    n1028 = case shown="\"低量程\", 默认" w1688 {
                      tunnel: [u16 4638 ("starting address") u16 4644 ("starting address") u16 4638 ("starting address")] -> w1689
                      frame "低量程", Default {
                      }
                      frame "高量程" {
                      }
                      frame "0-2量程" {
                      }
                    }
                  }
                  frame 3 {
                    n1029 = local read "量程选择"() -> (w1693:enum16{"低量程", "高量程", "0-2量程"})
                    n1030 = case shown="\"低量程\", 默认" w1693 {
                      tunnel: [u16 4650 ("starting address") u16 4656 ("starting address") u16 4638 ("starting address")] -> w1694
                      frame "低量程", Default {
                      }
                      frame "高量程" {
                      }
                      frame "0-2量程" {
                      }
                    }
                  }
                  frame 4 {
                    n1031 = local read "量程选择"() -> (w1698:enum16{"低量程", "高量程", "0-2量程"})
                    n1032 = case shown="\"低量程\", 默认" w1698 {
                      tunnel: [u16 4662 ("starting address") u16 4668 ("starting address") u16 4638 ("starting address")] -> w1699
                      frame "低量程", Default {
                      }
                      frame "高量程" {
                      }
                      frame "0-2量程" {
                      }
                    }
                  }
                  frame 5 {
                    n1033 = local read "量程选择"() -> (w1703:enum16{"低量程", "高量程", "0-2量程"})
                    n1034 = case shown="\"低量程\", 默认" w1703 {
                      tunnel: [u16 4674 ("starting address") u16 4680 ("starting address") u16 4638 ("starting address")] -> w1704
                      frame "低量程", Default {
                      }
                      frame "高量程" {
                      }
                      frame "0-2量程" {
                      }
                    }
                  }
                  frame 6 {
                    n1035 = local read "量程选择"() -> (w1708:enum16{"低量程", "高量程", "0-2量程"})
                    n1036 = case shown="\"低量程\", 默认" w1708 {
                      tunnel: [u16 4686 ("starting address") u16 4692 ("starting address") u16 4638 ("starting address")] -> w1709
                      frame "低量程", Default {
                      }
                      frame "高量程" {
                      }
                      frame "0-2量程" {
                      }
                    }
                  }
                  frame 7 {
                    n1037 = local read "量程选择"() -> (w1713:enum16{"低量程", "高量程", "0-2量程"})
                    n1038 = case shown="\"低量程\", 默认" w1713 {
                      tunnel: [u16 4698 ("starting address") u16 4704 ("starting address") u16 4638 ("starting address")] -> w1714
                      frame "低量程", Default {
                      }
                      frame "高量程" {
                      }
                      frame "0-2量程" {
                      }
                    }
                  }
                }
                n1039 = Build Array(w1674, w1679, w1678) -> (w1680:dbl[])
                n1040 = call "浮点转CDAB整形cod.vi"("浮点数"=w1680) -> ("CDAB整形输出"=w1675:u16[])  [unwired: 10 in]
              }
            }
            n1041 = local read "多项式系数"() -> (w1597:dbl[])
            n1042 = call "CODMnMB_api.vi"("STEP"=enum16{"open", "read", "write", "close"}."write", "values"=w1600, "starting address"=w1601) -> ("error out"=w1599:errorcluster)  [unwired: 6 in, 2 out]
            n1043 = Index Array(array=w1597) -> (element #1=w1596:dbl, element #2=w1595:dbl, element #3=w1594:dbl)  [unwired: 3 in]
            n1044 = case shown="无错误" w1599 {
              tunnel: ["写入成功！" "写入失败！"] -> w1598
              tunnel: w1596 -> [w1609 _]
              tunnel: w1595 -> [w1608 _]
              tunnel: w1594 -> [w1607 _]
              frame No Error {
                n1045 = Number To Fractional String(number=w1609) -> (F-format string=w1605:string)  [unwired: 3 in]
                n1046 = Number To Fractional String(number=w1608) -> (F-format string=w1606:string)  [unwired: 3 in]
                n1047 = Number To Fractional String(number=w1607) -> (F-format string=w1604:string)  [unwired: 3 in]
                n1048 = property on="模型" class="Enum (严格)"() -> ("RingText.Text"=w1619:string)  [unwired: 2 in, 2 out]
                n1049 = property on="测量模式(公式)" class="Ring (严格)"() -> ("RingText.Text"=w1618:string)  [unwired: 2 in, 2 out]
                n1050 = property on="量程选择" class="Enum (严格)"() -> ("RingText.Text"=w1617:string)  [unwired: 2 in, 2 out]
                n1051 = Concatenate Strings("变更后:" ("table输入"), "K:" ("字符串"), w1606, "B:" ("字符串"), w1605, "X^2:" ("字符串"), w1604) -> (w1610:string)
                n1052 = Concatenate Strings(w1619, w1618, w1617, "公式改变" ("日志信息")) -> (w1611:string)
                n1053 = Get Date/Time In Seconds() -> (seconds since 1Jan1904=w1623:timestamp)
                n1054 = Bundle(cluster=T5 {"时间标识"=timestamp(0 s since 1904-01-01), "参数"="", "日志信息"="", "流程参数"=""} ("data in"), "时间标识"=w1623, "参数"="CODMn" ("table输入"), "日志信息"=w1611, "流程参数"=w1610) -> (w1621:T5)
                n1055 = call "流程日志字段定义.vi"("table输入"="操作日志", "data in"=w1621) -> ("table输出"=w1626:string, "columns"=w1627:string[], "data out"=w1628:T6)  [unwired: 7 in]
                n1056 = call "插入数据.vi"("data"=w1628, "columns"=w1627, "database"="database3.mdb", "table"=w1626) -> ()  [unwired: 7 in, 1 out]
              }
              frame Error {
              }
            }
            n1057 = One Button Dialog(message=w1598) -> ()  [unwired: 1 in, 1 out]
          }
        }
      }
      event "一键写入": Value Change {
        n1058 = event-data() -> ()  [unwired: 1 in, 6 out]
        n1059 = Two Button Dialog(message="确认是否写入公式，写入会覆盖原有公式！" ("消息")) -> (T button?=w1718:bool)  [unwired: 2 in]
        n1060 = case shown="真" w1718 {
          frame False {
          }
          frame True {
            n1061 = local read "模型"() -> (w1722:enum32{"线性", "多项式"})
            n1062 = case shown="\"线性\", 默认" w1722 {
              tunnel: [w1751 w1802] -> w1720
              frame "线性", Default {
                n1063 = property on="测量模式(公式)" class="Ring (严格)"() -> ("NumItems"=w1752:u32)  [unwired: 2 in, 2 out]
                n1064 = for {
                  N: w1752 -> [_]
                  tunnel: [w1753] -> w1751
                  i -> [w1758]
                  n1065 = Increment(x=w1758) -> (x+1=w1757:i32)
                  n1066 = local read "K"() -> (w1762:dbl)
                  n1067 = local read "b"() -> (w1763:dbl)
                  n1068 = case shown="1" w1757 {
                    tunnel: [u16 4626 ("starting address") w1768 w1773 w1778 w1783 w1788 w1793 w1798] -> w1755
                    frame 0, Default {
                    }
                    frame 1 {
                      n1069 = local read "量程选择"() -> (w1767:enum16{"低量程", "高量程", "0-2量程"})
                      n1070 = case shown="\"低量程\", 默认" w1767 {
                        tunnel: [u16 4626 ("starting address") u16 4632 ("starting address") u16 4638 ("starting address")] -> w1768
                        frame "低量程", Default {
                        }
                        frame "高量程" {
                        }
                        frame "0-2量程" {
                        }
                      }
                    }
                    frame 2 {
                      n1071 = local read "量程选择"() -> (w1772:enum16{"低量程", "高量程", "0-2量程"})
                      n1072 = case shown="\"低量程\", 默认" w1772 {
                        tunnel: [u16 4638 ("starting address") u16 4644 ("starting address") u16 4638 ("starting address")] -> w1773
                        frame "低量程", Default {
                        }
                        frame "高量程" {
                        }
                        frame "0-2量程" {
                        }
                      }
                    }
                    frame 3 {
                      n1073 = local read "量程选择"() -> (w1777:enum16{"低量程", "高量程", "0-2量程"})
                      n1074 = case shown="\"低量程\", 默认" w1777 {
                        tunnel: [u16 4650 ("starting address") u16 4656 ("starting address") u16 4638 ("starting address")] -> w1778
                        frame "低量程", Default {
                        }
                        frame "高量程" {
                        }
                        frame "0-2量程" {
                        }
                      }
                    }
                    frame 4 {
                      n1075 = local read "量程选择"() -> (w1782:enum16{"低量程", "高量程", "0-2量程"})
                      n1076 = case shown="\"高量程\"" w1782 {
                        tunnel: [u16 4662 ("starting address") u16 4668 ("starting address") u16 4638 ("starting address")] -> w1783
                        frame "低量程", Default {
                        }
                        frame "高量程" {
                        }
                        frame "0-2量程" {
                        }
                      }
                    }
                    frame 5 {
                      n1077 = local read "量程选择"() -> (w1787:enum16{"低量程", "高量程", "0-2量程"})
                      n1078 = case shown="\"低量程\", 默认" w1787 {
                        tunnel: [u16 4674 ("starting address") u16 4680 ("starting address") u16 4638 ("starting address")] -> w1788
                        frame "低量程", Default {
                        }
                        frame "高量程" {
                        }
                        frame "0-2量程" {
                        }
                      }
                    }
                    frame 6 {
                      n1079 = local read "量程选择"() -> (w1792:enum16{"低量程", "高量程", "0-2量程"})
                      n1080 = case shown="\"低量程\", 默认" w1792 {
                        tunnel: [u16 4686 ("starting address") u16 4692 ("starting address") u16 4638 ("starting address")] -> w1793
                        frame "低量程", Default {
                        }
                        frame "高量程" {
                        }
                        frame "0-2量程" {
                        }
                      }
                    }
                    frame 7 {
                      n1081 = local read "量程选择"() -> (w1797:enum16{"低量程", "高量程", "0-2量程"})
                      n1082 = case shown="\"低量程\", 默认" w1797 {
                        tunnel: [u16 4698 ("starting address") u16 4704 ("starting address") u16 4638 ("starting address")] -> w1798
                        frame "低量程", Default {
                        }
                        frame "高量程" {
                        }
                        frame "0-2量程" {
                        }
                      }
                    }
                  }
                  n1083 = Build Array(w1762, w1763, 0.0 ("元素")) -> (w1764:dbl[])
                  n1084 = call "浮点转CDAB整形cod.vi"("浮点数"=w1764) -> ("CDAB整形输出"=w1761:u16[])  [unwired: 10 in]
                  n1085 = Insert Into Array(array=u16[] [], index=0 ("索引"), new element=w1761) -> (w1754:u16[])
                  n1086 = call "CODMnMB_api.vi"("STEP"=enum16{"open", "read", "write", "close"}."write", "values"=w1754, "starting address"=w1755) -> ("error out"=w1753:errorcluster)  [unwired: 6 in, 2 out]
                }
              }
              frame "多项式" {
                # "b,k,c"
                n1087 = property on="测量模式(公式)" class="Ring (严格)"() -> ("NumItems"=w1803:u32)  [unwired: 2 in, 2 out]
                n1088 = for {
                  N: w1803 -> [_]
                  tunnel: [w1804] -> w1802
                  i -> [w1809]
                  n1089 = Increment(x=w1809) -> (x+1=w1808:i32)
                  n1090 = local read "多项式系数"() -> (w1813:dbl[])
                  n1091 = case shown="2" w1808 {
                    tunnel: [u16 4626 ("starting address") w1820 w1825 w1830 w1835 w1840 w1845 w1850] -> w1805
                    frame 0, Default {
                    }
                    frame 1 {
                      n1092 = local read "量程选择"() -> (w1819:enum16{"低量程", "高量程", "0-2量程"})
                      n1093 = case shown="\"低量程\", 默认" w1819 {
                        tunnel: [u16 4626 ("starting address") u16 4632 ("starting address") u16 4638 ("starting address")] -> w1820
                        frame "低量程", Default {
                        }
                        frame "高量程" {
                        }
                        frame "0-2量程" {
                        }
                      }
                    }
                    frame 2 {
                      n1094 = local read "量程选择"() -> (w1824:enum16{"低量程", "高量程", "0-2量程"})
                      n1095 = case shown="\"低量程\", 默认" w1824 {
                        tunnel: [u16 4638 ("starting address") u16 4644 ("starting address") u16 4638 ("starting address")] -> w1825
                        frame "低量程", Default {
                        }
                        frame "高量程" {
                        }
                        frame "0-2量程" {
                        }
                      }
                    }
                    frame 3 {
                      n1096 = local read "量程选择"() -> (w1829:enum16{"低量程", "高量程", "0-2量程"})
                      n1097 = case shown="\"低量程\", 默认" w1829 {
                        tunnel: [u16 4650 ("starting address") u16 4656 ("starting address") u16 4638 ("starting address")] -> w1830
                        frame "低量程", Default {
                        }
                        frame "高量程" {
                        }
                        frame "0-2量程" {
                        }
                      }
                    }
                    frame 4 {
                      n1098 = local read "量程选择"() -> (w1834:enum16{"低量程", "高量程", "0-2量程"})
                      n1099 = case shown="\"低量程\", 默认" w1834 {
                        tunnel: [u16 4662 ("starting address") u16 4668 ("starting address") u16 4638 ("starting address")] -> w1835
                        frame "低量程", Default {
                        }
                        frame "高量程" {
                        }
                        frame "0-2量程" {
                        }
                      }
                    }
                    frame 5 {
                      n1100 = local read "量程选择"() -> (w1839:enum16{"低量程", "高量程", "0-2量程"})
                      n1101 = case shown="\"低量程\", 默认" w1839 {
                        tunnel: [u16 4674 ("starting address") u16 4680 ("starting address") u16 4638 ("starting address")] -> w1840
                        frame "低量程", Default {
                        }
                        frame "高量程" {
                        }
                        frame "0-2量程" {
                        }
                      }
                    }
                    frame 6 {
                      n1102 = local read "量程选择"() -> (w1844:enum16{"低量程", "高量程", "0-2量程"})
                      n1103 = case shown="\"低量程\", 默认" w1844 {
                        tunnel: [u16 4686 ("starting address") u16 4692 ("starting address") u16 4638 ("starting address")] -> w1845
                        frame "低量程", Default {
                        }
                        frame "高量程" {
                        }
                        frame "0-2量程" {
                        }
                      }
                    }
                    frame 7 {
                      n1104 = local read "量程选择"() -> (w1849:enum16{"低量程", "高量程", "0-2量程"})
                      n1105 = case shown="\"低量程\", 默认" w1849 {
                        tunnel: [u16 4698 ("starting address") u16 4704 ("starting address") u16 4638 ("starting address")] -> w1850
                        frame "低量程", Default {
                        }
                        frame "高量程" {
                        }
                        frame "0-2量程" {
                        }
                      }
                    }
                  }
                  n1106 = Index Array(array=w1813) -> (element #1=w1816:dbl, element #2=w1815:dbl, element #3=w1817:dbl)  [unwired: 3 in]
                  n1107 = Build Array(w1815, w1816, w1817) -> (w1814:dbl[])
                  n1108 = call "浮点转CDAB整形cod.vi"("浮点数"=w1814) -> ("CDAB整形输出"=w1812:u16[])  [unwired: 10 in]
                  n1109 = Insert Into Array(array=u16[] [], index=0 ("索引"), new element=w1812) -> (w1806:u16[])
                  n1110 = call "CODMnMB_api.vi"("STEP"=enum16{"open", "read", "write", "close"}."write", "values"=w1806, "starting address"=w1805) -> ("error out"=w1804:errorcluster)  [unwired: 6 in, 2 out]
                }
              }
            }
            n1111 = case shown="无错误" w1720 {
              tunnel: ["写入成功！" "写入失败！"] -> w1721
              frame No Error {
                n1112 = local read "多项式系数"() -> (w1726:dbl[])
                n1113 = Index Array(array=w1726) -> (element #1=w1725:dbl, element #2=w1724:dbl, element #3=w1723:dbl)  [unwired: 3 in]
                n1114 = Number To Fractional String(number=w1725) -> (F-format string=w1729:string)  [unwired: 3 in]
                n1115 = Number To Fractional String(number=w1724) -> (F-format string=w1730:string)  [unwired: 3 in]
                n1116 = Number To Fractional String(number=w1723) -> (F-format string=w1728:string)  [unwired: 3 in]
                n1117 = property on="模型" class="Enum (严格)"() -> ("RingText.Text"=w1739:string)  [unwired: 2 in, 2 out]
                n1118 = property on="量程选择" class="Enum (严格)"() -> ("RingText.Text"=w1738:string)  [unwired: 2 in, 2 out]
                n1119 = Concatenate Strings("变更后:" ("table输入"), "K:" ("字符串"), w1730, "B:" ("字符串"), w1729, "X^2:" ("字符串"), w1728) -> (w1731:string)
                n1120 = Concatenate Strings(w1739, "【一键写入全部模式】" ("日志信息"), w1738, "公式改变" ("日志信息")) -> (w1732:string)
                n1121 = Get Date/Time In Seconds() -> (seconds since 1Jan1904=w1743:timestamp)
                n1122 = Bundle(cluster=T5 {"时间标识"=timestamp(0 s since 1904-01-01), "参数"="", "日志信息"="", "流程参数"=""} ("data in"), "时间标识"=w1743, "参数"="CODMn" ("table输入"), "日志信息"=w1732, "流程参数"=w1731) -> (w1741:T5)
                n1123 = call "流程日志字段定义.vi"("table输入"="操作日志", "data in"=w1741) -> ("table输出"=w1746:string, "columns"=w1747:string[], "data out"=w1748:T6)  [unwired: 7 in]
                n1124 = call "插入数据.vi"("data"=w1748, "columns"=w1747, "database"="database3.mdb", "table"=w1746) -> ()  [unwired: 7 in, 1 out]
              }
              frame Error {
              }
            }
            n1125 = One Button Dialog(message=w1721) -> ()  [unwired: 1 in, 1 out]
          }
        }
      }
      event "滴定曲线": Value Change {
        n1126 = event-data() -> ()  [unwired: 1 in, 6 out]
        n1127 = property on="窗格" class="Pane"("Origin"=T2 {"Horizontal"=0, "Vertical"=3200} ("原点")) -> ()  [unwired: 2 in, 2 out]
      }
      event "历史波形": Value Change {
        n1128 = event-data() -> ()  [unwired: 1 in, 6 out]
        n1129 = call-poly <vilib>:"Read Waveforms from File.vi"() -> ("error out"=w1855:errorcluster, "first waveform in record"=w1856:waveform(dbl))  [unwired: 6 in, 2 out]
        n1130 = case shown="无错误" w1855 {
          tunnel: w1856 -> [w1859 _]
          frame No Error {
            n1131 = Unbundle By Name(w1859) -> ("t0"=w1857:timestamp, "Y"=w1858:dbl[])  [unwired: 2 out]
            n1132 = global write "COD内部交互全局.vi" "波形时间"(w1857) -> ()
            n1133 = global write "COD内部交互全局.vi" "ORP滴定曲线"(w1858) -> ()
            n1134 = global write "COD内部交互全局.vi" "滴定数-ORP值"(w1858) -> ()
          }
          frame Error {
            n1135 = One Button Dialog(message="打开失败" ("消息")) -> ()  [unwired: 1 in, 1 out]
          }
        }
      }
      event "释放串口": Value Change {
        n1136 = event-data() -> ()  [unwired: 1 in, 6 out]
        n1137 = Two Button Dialog(message="确认是否释放串口，释放串口将导致通信失败！" ("消息")) -> (T button?=w1861:bool)  [unwired: 2 in]
        n1138 = case shown="真" w1861 {
          tunnel: w1864 -> [_ w1866]
          tunnel: w1863 -> [_ w1865]
          frame False {
          }
          frame True {
            n1139 = Bundle By Name(cluster=cluster{"命令":string} {"命令"=""} ("元素"), "命令"="停用模块" ("名称（未命名）")) -> (w1867:cluster{"命令":string})
            n1140 = Enqueue Element(queue=w1866, element=w1867, error in (no error)=w1865) -> ()  [unwired: 1 in, 3 out]
          }
        }
      }
      event "打开串口": Value Change {
        n1141 = event-data() -> ()  [unwired: 1 in, 6 out]
        n1142 = flat-sequence {
          tunnel: w1871 -> [w1879]
          tunnel: w1870 -> [w1878]
          frame #0 {
            n1143 = global read "CODMn断电保存全局变量.vi" "VISA resource name"() -> (w1882:refnum<visa-resource-name>)
            n1144 = global read "CODMn断电保存全局变量.vi" "MB通信方式选择"() -> (w1875:enum16{"串口", "TCP"})
            n1145 = global read "CODMn断电保存全局变量.vi" "PORT"() -> (w1873:string)
            n1146 = global read "CODMn断电保存全局变量.vi" "IP"() -> (w1874:string)
            n1147 = call "串口配置.vi"("PORT"=w1873, "IP"=w1874, "MB通信方式选择"=w1875, "请选择串口:"=w1882) -> ("PORT 2"=w1876:string, "IP 2"=w1877:string, "确认 2"=w1880:bool, "VISA资源名称 2"=w1881:refnum<visa-resource-name>, "MB通信方式选择 2"=w1872:enum16{"串口", "TCP"})  [unwired: 3 in]
            n1148 = case shown="真" w1880 {
              tunnel: w1881 -> [_ w1891]
              tunnel: w1879 -> [_ w1887]
              tunnel: w1878 -> [_ w1886]
              tunnel: w1877 -> [_ w1885]
              tunnel: w1876 -> [_ w1884]
              tunnel: w1872 -> [_ w1883]
              frame False {
              }
              frame True {
                n1149 = global write "CODMn断电保存全局变量.vi" "IP"(w1885) -> ()
                n1150 = global write "CODMn断电保存全局变量.vi" "PORT"(w1884) -> ()
                n1151 = global write "CODMn断电保存全局变量.vi" "VISA resource name"(w1891) -> ()
                n1152 = global write "CODMn断电保存全局变量.vi" "MB通信方式选择"(w1883) -> ()
                n1153 = Bundle By Name(cluster=cluster{"命令":string} {"命令"=""} ("元素"), "命令"="启用模块" ("名称（未命名）")) -> (w1888:cluster{"命令":string})
                n1154 = Enqueue Element(queue=w1887, element=w1888, error in (no error)=w1886) -> ()  [unwired: 1 in, 3 out]
              }
            }
          }
          frame #1 {
            n1155 = call "配置文件保存.vi"() -> ()  [unwired: 12 in]
          }
        }
      }
      event "更新程序": Value Change {
        n1156 = event-data() -> ("CtlRef"=w1894:refnum<vi>, "NewVal"=w1895:bool)  [unwired: 1 in, 4 out]
        n1157 = case shown="真" w1895 {
          tunnel: w1894 -> [_ w1904]
          tunnel: w1893 -> [w1897 w1903]
          tunnel: w1892 -> [w1896 w1902]
          frame False {
            n1158 = Bundle By Name(cluster=cluster{"命令":string} {"命令"=""} ("元素"), "命令"="启用模块" ("名称（未命名）")) -> (w1898:cluster{"命令":string})
            n1159 = Enqueue Element(queue=w1897, element=w1898, error in (no error)=w1896) -> ()  [unwired: 1 in, 3 out]
          }
          frame True {
            n1160 = Two Button Dialog(message="警告，非专业人士请勿进行此操作！！！\n请确认是否继续？" ("消息")) -> (T button?=w1906:bool)  [unwired: 2 in]
            n1161 = case shown="真" w1906 {
              tunnel: w1904 -> [w1922 _]
              tunnel: w1903 -> [_ w1930]
              tunnel: w1902 -> [_ w1929]
              tunnel: [errorcluster {"status"=TRUE, "code"=0, "source"=""} ("error out") w1923] -> w1901
              frame False {
                n1162 = property class="Bool (严格)"(reference=w1922, "Value"=FALSE ("释放串口")) -> ()  [unwired: 1 in, 2 out]
              }
              frame True {
                n1163 = Bundle By Name(cluster=cluster{"命令":string} {"命令"=""} ("元素"), "命令"="CODMn程序更新" ("名称（未命名）")) -> (w1933:cluster{"命令":string})
                n1164 = Enqueue Element(queue=w1930, element=w1933, error in (no error)=w1929) -> (queue out=w1928:refnum<queue>, error out=w1927:errorcluster)  [unwired: 1 in, 1 out]
                n1165 = Bundle By Name(cluster=cluster{"命令":string} {"命令"=""} ("元素"), "命令"="停用模块" ("名称（未命名）")) -> (w1924:cluster{"命令":string})
                n1166 = Enqueue Element(queue=w1928, element=w1924, error in (no error)=w1927) -> (error out=w1923:errorcluster)  [unwired: 1 in, 2 out]
              }
            }
            n1167 = case shown="无错误" w1901 {
              frame No Error {
                n1168 = call "文件对话框"("start path"=path "D:/SRC") -> ("selected path"=w1909:path, "cancelled"=w1907:bool)  [unwired: 11 in, 2 out]
                n1169 = case shown="假" w1907 {
                  tunnel: w1909 -> [w1914 _]
                  frame False {
                    n1170 = Path To String(path=w1914) -> (string=w1911:string)
                    n1171 = Format Into String(format string="  - \"%s\"" ("格式字符串"), initial string="\"C:\\Program Files\\Fatek\\WinProladder\\WProlad.exe\"" ("command line"), w1911) -> (resulting string=w1912:string)  [unwired: 1 in, 1 out]
                    n1172 = call <vilib>:"System Exec.vi"("command line"=w1912) -> ("error out"=w1915:errorcluster)  [unwired: 7 in, 3 out]
                    n1173 = case shown="错误" w1915 {
                      tunnel: w1911 -> [_ w1918]
                      frame No Error {
                      }
                      frame Error {
                        n1174 = Format Into String(format string="  - \"%s\"" ("格式字符串"), initial string="\"C:\\Program Files (x86)\\Fatek\\WinProladder\\WProlad.exe\"" ("command line"), w1918) -> (resulting string=w1916:string)  [unwired: 1 in, 1 out]
                        n1175 = call <vilib>:"System Exec.vi"("command line"=w1916) -> ()  [unwired: 7 in, 4 out]
                      }
                    }
                  }
                  frame True {
                  }
                }
              }
              frame Error {
              }
            }
          }
        }
      }
      event "序列号变更": Value Change {
        n1176 = event-data() -> ()  [unwired: 1 in, 6 out]
        n1177 = local read "CODMn序列号"() -> (w1937:string)
        n1178 = call "序列号写入.vi"("序列号:"=w1937) -> ("确认 2"=w1934:bool, "序列号输出"=w1938:string)  [unwired: 9 in]
        n1179 = case shown="真" w1934 {
          tunnel: w1938 -> [_ w1944]
          tunnel: w1936 -> [_ w1940]
          tunnel: w1935 -> [_ w1939]
          frame False {
          }
          frame True {
            n1180 = global write "COD内部交互全局.vi" "序列号:"(w1944) -> ()
            n1181 = Bundle By Name(cluster=cluster{"命令":string} {"命令"=""} ("元素"), "命令"="CODMn序列号写入" ("名称（未命名）")) -> (w1941:cluster{"命令":string})
            n1182 = Enqueue Element(queue=w1940, element=w1941, error in (no error)=w1939) -> ()  [unwired: 1 in, 3 out]
          }
        }
      }
      event Timeout {
        n1183 = event-data() -> ()  [unwired: 1 in, 3 out]
      }
    }
  }
  n1184 = while {
    stop <- FALSE stop-if-true
    n1185 = global read "COD内部交互全局.vi" "待机"() -> (w1946:bool)
    n1186 = Wait (ms)(milliseconds to wait=u32 1000 ("等待时间（毫秒）")) -> ()  [unwired: 1 out]
    n1187 = case shown="假" w1946 {
      tunnel: [w1963 T7."Enabled" ("禁用")] -> w1948
      tunnel: [w1962 _] -> w1947
      frame False {
        # "运行中"
        n1188 = local read "校标标记"() -> (w1961:bool)
        n1189 = local read "校零标记"() -> (w1960:bool)
        n1190 = Or(x=w1961, y=w1960) -> (x .or. y?=w1964:bool)
        n1191 = case shown="真" w1964 {
          tunnel: [T7."Enabled" ("禁用") T7."Disabled and Grayed Out" ("禁用")] -> w1963
          tunnel: [_ TRUE] -> w1962
          frame False {
          }
          frame True {
          }
        }
      }
      frame True {
      }
    }
    n1192 = control-ref of="量程选择"() -> (w1954:refnum<vi>)
    n1193 = property on="校准内容显示" class="Str"("Visible"=w1947) -> ()  [unwired: 2 in, 2 out]
    n1194 = control-ref of="选用水样"() -> (w1955:refnum<vi>)
    n1195 = control-ref of="校准5"() -> (w1949:refnum<vi>)
    n1196 = control-ref of="校准4"() -> (w1950:refnum<vi>)
    n1197 = control-ref of="校准3"() -> (w1951:refnum<vi>)
    n1198 = control-ref of="校准2"() -> (w1952:refnum<vi>)
    n1199 = control-ref of="校准1"() -> (w1953:refnum<vi>)
    n1200 = Build Array(w1949, w1950, w1951, w1952, w1953, w1955, w1954) -> (w1956:refnum<vi>[])
    n1201 = for {
      tunnel: w1956 -> [w1959] mode=indexing
      tunnel: w1948 -> [w1958]
      n1202 = property class="Ctl"(reference=w1959, "DisabledEnum"=w1958) -> ()  [unwired: 1 in, 2 out]
    }
  }
  n1203 = while {
    stop <- FALSE stop-if-true
    # "滚动显示"
    n1204 = global read "COD内部交互全局.vi" "待机"() -> (w1969:bool)
    n1205 = case shown="假" w1969 {
      frame False {
        # "运行中"
        n1206 = global read "COD内部交互全局.vi" "校准内容显示"() -> (w1972:string)
        n1207 = while {
          shift-right: [w1974] -> _
          shift-left: w1972 -> [w1979]
          stop <- w1973 stop-if-true
          (unwired) "仪器校准中!\n当前校准浓度为:3mg/L" ("校准内容显示")
          n1208 = Wait (ms)(milliseconds to wait=u32 500 ("等待时间（毫秒）")) -> ()  [unwired: 1 out]
          n1209 = Spreadsheet String To Array(delimiter (Tab)="\n" ("分隔符(Tab)"), format string="" ("格式字符串"), spreadsheet string=w1979, array type (2D Dbl)=string[] []) -> (array=w1982:string[])
          n1210 = for {
            tunnel: w1982 -> [w1990] mode=indexing
            tunnel: [w1988] -> _ mode=indexing
            shift-right: [w1986] -> w1977
            shift-left: "" ("格式字符串") -> [w1987]
            n1211 = call "字符串移位显示.vi"("字符框大小"=36, "字符串输入"=w1990) -> ("移位后字符串"=w1988:string)  [unwired: 8 in, 1 out]
            n1212 = Concatenate Strings(w1987, w1988, "\n" ("分隔符(Tab)")) -> (w1986:string)
          }
          n1213 = String Length(string=w1977) -> (length=w1976:i32)
          n1214 = Decrement(x=w1976) -> (x-1=w1975:i32)
          n1215 = String Subset(string=w1977, length (rest)=w1975) -> (substring=w1974:string)  [unwired: 1 in]
          "校准内容显示" <- w1974
          n1216 = global read "COD内部交互全局.vi" "待机"() -> (w1973:bool)
        }
      }
      frame True {
      }
    }
    n1217 = Wait (ms)(milliseconds to wait=u32 1000 ("等待时间（毫秒）")) -> ()  [unwired: 1 out]
  }
  n1218 = while {
    stop <- FALSE stop-if-true
    w2024 = T16 0 items=["最小二乘", "最小绝对残差", "Bisquare"] ("method")
    # "计算线性、多项式公式、远程校准"
    n1219 = local read "浓度1"() -> (w1997:dbl)
    n1220 = local read "浓度2"() -> (w2026:dbl)
    n1221 = local read "浓度3"() -> (w2027:dbl)
    n1222 = local read "浓度4"() -> (w2019:dbl)
    n1223 = local read "浓度5"() -> (w2018:dbl)
    n1224 = Build Array("泵滴定数1", "泵滴定数2", "泵滴定数3", "泵滴定数4", "泵滴定数5") -> (w2025:dbl[])
    n1225 = Build Array(w1997, w2026, w2027, w2019, w2018) -> (w1993:dbl[])
    n1226 = Build Array("启用1", "启用2", "启用3", "启用4", "启用5") -> (w1996:bool[])
    n1227 = global read "CODMN外部API.vi" "远程反控校准CODMn"() -> (w1994:bool)
    n1228 = call "将启用的浓度作为新的浓度数组.vi"("启用布尔数组"=w1996, "输入浓度数组"=w1993) -> ("启用的浓度数组"=w1995:dbl[])  [unwired: 13 in]
    n1229 = Unbundle By Name("方程系数") -> ("K"=w2005:dbl, "b"=w2004:dbl, "X^2"=w2003:dbl)
    n1230 = case shown="\"多项式\"" "模型" {
      tunnel: w2005 -> [w2036 w2039]
      tunnel: w2004 -> [w2035 w2040]
      tunnel: w2003 -> [_ w2038]
      frame "线性", Default {
        "K" <- w2036
        "b" <- w2035
      }
      frame "多项式" {
        n1231 = Build Array(w2040, w2039, w2038) -> (→"多项式系数":dbl[])
      }
    }
    n1232 = call "线性公式CODMn用.vi"("标液浓度"=w1993, "监测浓度"=w2025, "启用"=w1996, "method"=w2024, "模型"="模型", "精度"=6) -> ("拟合方程"=w2011:string, "r^2"=→"r^2":dbl, "slope"=w2009:dbl, "intercept"=w2010:dbl, "XY图"=→"XY图":cluster{"X Values":dbl[], "Y Values":dbl[]}[], "Polynomial Coefficients"=w2020:dbl[])  [unwired: 8 in]
    "拟合公式" <- w2011
    n1233 = call <vilib>:"Boolean Crossing PtByPt.vi"("direction"=enum16{"either", "false-true", "true-false"}."false-true", "input"=w1994) -> ("crossing"=w1992:bool)  [unwired: 1 in]
    n1234 = case shown="真" w1992 {
      tunnel: w1993 -> [_ w2030]
      frame False {
      }
      frame True {
        n1235 = global read "CODMn断电保存全局变量.vi" "远程自动校准浓度"() -> (w2031:dbl)
        n1236 = Search 1D Array(1D array=w2030, element=w2031) -> (index of element=w2032:i32)  [unwired: 1 in]
        n1237 = case shown="0, 默认" w2032 {
          selector: w2032 -> [_ w2034]
          frame -1 {
          }
          frame 0, Default {
            n1238 = Increment(x=w2034) -> (x+1=w2033:i32)
            n1239 = global write "COD内部交互全局.vi" "当前校准"(w2033) -> ()
          }
        }
      }
    }
    n1240 = feedback #3(w2011) -> (w2012:string)
    n1241 = feedback-in #3(w2011) -> ()
    n1242 = Not Equal?(x=w2011, y=w2012) -> (x != y?=w2008:bool)
    n1243 = global write "COD内部交互全局.vi" "启用的浓度数组"(w1995) -> ()
    n1244 = case shown="真" w2008 {
      tunnel: w2020 -> [_ w2047]
      tunnel: w2010 -> [_ w2048]
      tunnel: w2009 -> [_ w2049]
      frame False {
      }
      frame True {
        # "当公式发生改变时赋值到右侧公式"
        n1245 = local read "模型"() -> (w2050:enum32{"线性", "多项式"})
        n1246 = case shown="\"多项式\"" w2050 {
          tunnel: [w2055 w2057] -> w2043
          tunnel: w2049 -> [w2055 _]
          tunnel: w2048 -> [w2054 _]
          tunnel: [w2054 w2058] -> w2044
          tunnel: w2047 -> [_ w2059]
          tunnel: [0.0 ("数值") w2056] -> w2042
          frame "线性", Default {
          }
          frame "多项式" {
            # "B,K,X^2"
            n1247 = Index Array(array=w2059) -> (element #1=w2058:dbl, element #2=w2057:dbl, element #3=w2056:dbl)  [unwired: 3 in]
          }
        }
        n1248 = global read "CODMn断电保存全局变量.vi" "CODMn仪器参数"() -> (w2046:T14)
        n1249 = local read "r^2"() -> (w2041:dbl)
        n1250 = Bundle By Name(cluster=cluster{"K":dbl, "b":dbl, "X^2":dbl} {"K"=0.0, "b"=0.0, "X^2"=0.0} ("方程系数"), "K"=w2043, "b"=w2044, "X^2"=w2042) -> (w2051:cluster{"K":dbl, "b":dbl, "X^2":dbl})
        n1251 = Bundle By Name(cluster=w2046, "曲线截距"=w2044, "曲线斜率"=w2043, "二次多项式系数"=w2042, "线性相关系数"=w2041) -> (w2045:T14)
        n1252 = global write "CODMn断电保存全局变量.vi" "CODMn仪器参数"(w2045) -> ()
        n1253 = local write "方程系数"(w2051) -> ()
      }
    }
    n1254 = Wait (ms)(milliseconds to wait=u32 1000 ("等待时间（毫秒）")) -> ()  [unwired: 1 out]
  }
  n1255 = property class="VI"(reference=w55, error in=w54) -> ("Name"=w56:string)  [unwired: 2 out]
  n1256 = Open VI Reference(type specifier VI Refnum (for type only)=refnum<vi> refnum, vi path=w56, options=128 ("选项")) -> (vi reference=w58:refnum<vi>, error out=w60:errorcluster)  [unwired: 3 in]
  n1257 = property class="VI"(reference=w40, error in=errorcluster {"status"=FALSE, "code"=0, "source"=""} ("错误输出")) -> ("Name"=w41:string)  [unwired: 2 out]
  n1258 = call-by-ref "?"(reference=w58, error in=w60) -> (reference out=w62:refnum<vi>, error out=w61:errorcluster)  [unwired: 12 in]
  n1259 = property class="VI"(reference=w39, error in=errorcluster {"status"=FALSE, "code"=0, "source"=""} ("错误输出")) -> ("Name"=w38:string)  [unwired: 2 out]
  n1260 = property class="VI"(reference=w26, error in=errorcluster {"status"=FALSE, "code"=0, "source"=""} ("错误输出")) -> ("Name"=w27:string)  [unwired: 2 out]
  n1261 = Open VI Reference(type specifier VI Refnum (for type only)=refnum<vi> refnum, vi path=w41, options=128 ("选项")) -> (vi reference=w21:refnum<vi>, error out=w43:errorcluster)  [unwired: 3 in]
  n1262 = Close Reference(reference=w62, error in (no error)=w61) -> ()  [unwired: 1 out]
  n1263 = property class="VI"(reference=w53, error in=errorcluster {"status"=FALSE, "code"=0, "source"=""} ("错误输出")) -> ("Name"=w52:string)  [unwired: 2 out]
  n1264 = call-by-ref "?"(reference=w21, error in=w43) -> (reference out=w45:refnum<vi>, error out=w44:errorcluster)  [unwired: 12 in]
  n1265 = Open VI Reference(type specifier VI Refnum (for type only)=refnum<vi> refnum, vi path=w38, options=128 ("选项")) -> (vi reference=w22:refnum<vi>, error out=w36:errorcluster)  [unwired: 3 in]
  n1266 = Open VI Reference(type specifier VI Refnum (for type only)=refnum<vi> refnum, vi path=w27, options=128 ("选项")) -> (vi reference=w25:refnum<vi>, error out=w29:errorcluster)  [unwired: 3 in]
  n1267 = call-by-ref "?"(reference=w22, error in=w36) -> (reference out=w34:refnum<vi>, error out=w35:errorcluster)  [unwired: 12 in]
  n1268 = Close Reference(reference=w45, error in (no error)=w44) -> ()  [unwired: 1 out]
  n1269 = call-by-ref "?"(reference=w25, error in=w29) -> (reference out=w31:refnum<vi>, error out=w30:errorcluster)  [unwired: 12 in]
  n1270 = Open VI Reference(type specifier VI Refnum (for type only)=refnum<vi> refnum, vi path=w52, options=128 ("选项")) -> (vi reference=w18:refnum<vi>, error out=w50:errorcluster)  [unwired: 3 in]
  n1271 = Close Reference(reference=w34, error in (no error)=w35) -> ()  [unwired: 1 out]
  n1272 = call-by-ref "?"(reference=w18, error in=w50) -> (reference out=w48:refnum<vi>, error out=w49:errorcluster)  [unwired: 12 in]
  n1273 = Close Reference(reference=w31, error in (no error)=w30) -> ()  [unwired: 1 out]
  n1274 = Close Reference(reference=w48, error in (no error)=w49) -> ()  [unwired: 1 out]
  n1275 = vi-ref "斯坦道CODMn.lvlib:关键参数交互.vi"() -> (w13:refnum<vi>)
  n1276 = control-ref of="测量模式(公式)"() -> (w5:refnum<vi>)
  n1277 = control-ref of="量程选择"() -> (w3:refnum<vi>)
  n1278 = control-ref of="模型"() -> (w6:refnum<vi>)
  n1279 = property class="VI"(reference=w13, error in=errorcluster {"status"=FALSE, "code"=0, "source"=""} ("错误输出")) -> ("Name"=w12:string)  [unwired: 2 out]
  n1280 = property class="Enum (严格)"(reference=w6) -> ("Value"=w4:enum32{"线性", "多项式"})  [unwired: 1 in, 2 out]
  n1281 = property class="Ring (严格)"(reference=w5) -> ("Value"=w1:u16)  [unwired: 1 in, 2 out]
  n1282 = property class="Enum (严格)"(reference=w3) -> ("Value"=w2:enum16{"低量程", "高量程", "0-2量程"})  [unwired: 1 in, 2 out]
  n1283 = Open VI Reference(type specifier VI Refnum (for type only)=refnum<vi> refnum, vi path=w12, options=128 ("选项")) -> (vi reference=w14:refnum<vi>, error out=w10:errorcluster)  [unwired: 3 in]
  n1284 = call-by-ref "?"(reference=w14, error in=w10, "量程选择"=w2, "测量模式(公式)"=w1, "模型"=w4) -> (reference out=w8:refnum<vi>, error out=w9:errorcluster)  [unwired: 9 in]
  n1285 = Close Reference(reference=w8, error in (no error)=w9) -> ()  [unwired: 1 out]
